vi "Text control 2 v5.8_pump-specific.vi"() -> ()   [LabVIEW 2016]
panel:
  in  "Tab Control":enum32{"Main", "Other parameters"}(tab)
  out "Line running":i32
  out "Total lines":i32
  out "Path":path=path "C:/users/rlp38/09Apr2009LTtesting/test2.txt"
  out "I vs Vg":cluster{"Y data in":dbl[], "X data in":dbl[]}[](graph)
  out "Is max":dbl format="%.2e"
  out "Id max":dbl format="%.2e"
  out "Ig max":dbl format="%.2e"
  out "Imax vs time":cluster{"Y data in":dbl[], "X data in":dbl[]}[](graph)
  out "Imin vs time":cluster{"Y data in":dbl[], "X data in":dbl[]}[](graph)
  out "I vs Vd":cluster{"Y data in":dbl[], "X data in":dbl[]}[](graph)
  in  "Script":string="#-------------------------------------------------------\n# SPM pump cleaning script\n#\n# Version 0.5\n# Author: Dimitrios Simatos\n# Last updated: 2018-01-05\n#-------------------------------------------------------\n# Description\n#\n# This script is designed to run the cleaning sequence of the SPM OEM pump.\n# This script needs to be run 4 times!\n#-------------------------------------------------------\n# Changes\n#\n# Placed initialization and hard stop commands in the beginning.\n#-------------------------------------------------------\n# Important points\n#\n# Never leave any liquid in the pump to dry after the experiments. If they dry, the residue may block the valve.\n# Always run the cleaning cycle after the experiments.\n# Use clockwise rotation when going up in valve port numbers and vice versa.\n#-------------------------------------------------------\n# Things to do before running the script\n#\n# Set time units to minutes.\n# Set filenames.\n# Replace the tubing, if necessary.\n#-------------------------------------------------------\n# Port connections\n#\n# Port 1: Waste\n# Port 2: Waste\n# Port 3: Various cleaning liquids\n# Port 4: Waste\n# Port 5: Waste\n# Port 6: Waste\n#\n# Between each of the 4 runs, the settings of Port 3 will change, according to the cleaning protocol.\n# The settings for Port 3 are:\n# 1st run: 1% v/v solution of sodium hypochlorite in ultrapure water\n# 2nd run: 0.1% w/v solution of sodium dodecyl sulfate in ultrapure water\n# 3rd run: Ultrapure water\n# 4th run: Waste (in air, not immersed in liquid)\n#-------------------------------------------------------\n# Cleaning protocol for the SPM OEM pump (from the manual)\n#\n# A cleaning procedure should be performed at the end of each day or in between two different experiments.\n# An effective cleaning can be performed in the following manner:\n# • Bleach solution to kill microorganisms\n# 1. Prepare a solution of 1% chlorine bleach and deionized water\n#    NOTE: Prepare a 1% v/v solution of sodium hypochlorite in deionized water\n# 2. Prepare a reservoir and place 1 tubing in the bleach solution and 5 tubings in a waste recipient\n# 3. Pick up the bleach solution through 1 port to entirely fill the syringe\n# 4. Sequentially output the syringe content through the remaining ports and throw it to the waste\n# 5. Repeat operation at least 2 times\n# • Detergent solution to remove debris\n# 1. Prepare a solution of 0.1% detergent and deionized water\n#    NOTE: Prepare a 0.1% w/v solution of sodium dodecyl sulfate in deionized water\n# 2. Move the tubing from the bleach solution reservoir and place it into a reservoir of detergent solution\n# 3. Pick up the detergent solution through 1 port to entirely fill the syringe\n# 4. Sequentially output the detergent solution through the remaining ports into the waste recipient\n# 5. Repeat operation at least 2 times\n# • Rinsing water to prepare the pump for your next experiment\n# 1. Move the tubing from the detergent solution reservoir and place it into a reservoir of deionized water\n# 2. Pick up the rinsing solution through 1 port to entirely fill the syringe\n# 3. Sequentially output the rinse water through the remaining ports into the waste recipient\n# 4. Repeat operation at least 2 times\n# • Replace the tubing, if necessary\n#-------------------------------------------------------\n# Pumping cycles and execution time\n#\n# Execution time for a single cycle: 6 x (1 min + 10 sec) = 7 minutes\n# Total execution time: 4 x 7 = 28 minutes\n# Since the script has to run 4 times, the cleaning lasts for: 4 x 28 = 112 minutes\n# Air must be the last to be pumped through the valve, to remove all liquids.\n# There are 4 pumping cycles. Each one draws a different liquid through port 3 and pumps it sequentially through ports 1,2,4,5,6.\n# During the sequential pumping, each port receives 200 ml of liquid (20% of the total syringe volume = 600 \"plunger units\")\n# The device must be disconnected from the port during the cleaning procedure.\n# All cycles are similar, except cycle 1 has the initialization command uncommented and the first report valve command commented.\n#-------------------------------------------------------\n# Volume of liquid needed\n#\n# Volume of liquid needed per cycle: 1 ml\n# Total volume of liquid needed per script run: 4 x 1 = 4 ml\n# Since the script has to run 4 times, the first 3 with different liquids, I need:\n# 4 ml of 1% v/v solution of sodium hypochlorite in ultrapure water\n# 4 ml of 0.1% w/v solution of sodium dodecyl sulfate in ultrapure water\n# 4 ml of ultrapure water\n#-------------------------------------------------------\n# Parameters\n#\n# Syringe size: 1 ml\n# Step resolution N = 0.01 mm\n# Drawing flow V = 300 pulses/second (6000 ul/min)\n# Pumping flow V = 300 pulses/second (6000 ul/min)\n#-------------------------------------------------------\n# Pump initialization\npump /1T #hard stop pump\npump /1ZR #initialize pump\n#-------------------------------------------------------\n# Cycle 1\n# Fill the syringe\npump /1Q #query pump\npump /1? #report absolute plunger position\n#pump /1?6 #report valve position\nwait-min 1 #wait 1 minute\npump /1N0R #set step resolution: 0.01 mm\npump /1Q #query pump\npump /1? #report absolute plunger position (the plunger should be at 0)\npump /1?6 #report valve position\nwait 1000 #wait 1 second\npump /1V300R #choose speed: 300 steps/s (6000 ul/min)\npump /1Q #query pump\nwait 1000 #wait 1 second\npump /1I3R #go to port 3, clockwise rotation\npump /1Q #query pump\npump /1?6 #report valve position\nwait 1000 #wait 1 second\npump /1A3000R #go to absolute position 3000 (= draw 1 ml)\nwait 30000 #wait 30 seconds\npump /1Q #query pump\npump /1? #report absolute plunger position (the plunger should have finished moving)\n#pump /1?6 #report valve position\n# The sequential pumping begins\n# Port 1\npump /1O1R #switch to port 1, counterclockwise rotation\npump /1Q #query pump\npump /1?6 #report valve position\npump /1A2400R #go to absolute position 2400 (= pump 200 ul)\npump /1Q #query pump\npump /1? #report absolute plunger position (the plunger should be moving to 0)\nwait-min 1 #wait 1 minute\npump /1? #report absolute plunger position (the plunger should have finished moving)\n# Port 2\npump /1I2R #switch to port 2, clockwise rotation\npump /1Q #query pump\npump /1?6 #report valve position\npump /1A1800R #go to absolute position 1800 (= pump 200 ul)\npump /1Q #query pump\npump /1? #report absolute plunger position (the plunger should be moving to 0)\nwait-min 1 #wait 1 minute\npump /1? #report absolute plunger position (the plunger should have finished moving)\n# Port 4\npump /1I4R #switch to port 4, clockwise rotation\npump /1Q #query pump\npump /1?6 #report valve position\npump /1A1200R #go to absolute position 1200 (= pump 200 ul)\npump /1Q #query pump\npump /1? #report absolute plunger position (the plunger should be moving to 0)\nwait-min 1 #wait 1 minute\npump /1? #report absolute plunger position (the plunger should have finished moving)\n# Port 5\npump /1I5R #switch to port 5, clockwise rotation\npump /1Q #query pump\npump /1?6 #report valve position\npump /1A600R #go to absolute position 600 (= pump 200 ul)\npump /1Q #query pump\npump /1? #report absolute plunger position (the plunger should be moving to 0)\nwait-min 1 #wait 1 minute\npump /1? #report absolute plunger position (the plunger should have finished moving)\n# Port 6\npump /1I6R #switch to port 6, clockwise rotation\npump /1Q #query pump\npump /1?6 #report valve position\npump /1A0R #go to absolute position 0 (= pump 200 ul)\npump /1Q #query pump\npump /1? #report absolute plunger position (the plunger should be moving to 0)\nwait-min 1 #wait 1 minute\npump /1? #report absolute plunger position (the plunger should have finished moving)\n#-------------------------------------------------------\n# Cycle 2\n# Fill the syringe\n#pump /1ZR #initialize pump\npump /1Q #query pump\npump /1? #report absolute plunger position\npump /1?6 #report valve position\nwait-min 1 #wait 1 minute\npump /1N0R #set step resolution: 0.01 mm\npump /1Q #query pump\npump /1? #report absolute plunger position (the plunger should be at 0)\npump /1?6 #report valve position\nwait 1000 #wait 1 second\npump /1V300R #choose speed: 300 steps/s (6000 ul/min)\npump /1Q #query pump\nwait 1000 #wait 1 second\npump /1O3R #go to port 3, counterclockwise rotation\npump /1Q #query pump\npump /1?6 #report valve position\nwait 1000 #wait 1 second\npump /1A3000R #go to absolute position 3000 (= draw 1 ml)\nwait 30000 #wait 30 seconds\npump /1Q #query pump\npump /1? #report absolute plunger position (the plunger should have finished moving)\n#pump /1?6 #report valve position\n# The sequential pumping begins\n# Port 1\npump /1O1R #switch to port 1, counterclockwise rotation\npump /1Q #query pump\npump /1?6 #report valve position\npump /1A2400R #go to absolute position 2400 (= pump 200 ul)\npump /1Q #query pump\npump /1? #report absolute plunger position (the plunger should be moving to 0)\nwait-min 1 #wait 1 minute\npump /1? #report absolute plunger position (the plunger should have finished moving)\n# Port 2\npump /1I2R #switch to port 2, clockwise rotation\npump /1Q #query pump\npump /1?6 #report valve position\npump /1A1800R #go to absolute position 1800 (= pump 200 ul)\npump /1Q #query pump\npump /1? #report absolute plunger position (the plunger should be moving to 0)\nwait-min 1 #wait 1 minute\npump /1? #report absolute plunger position (the plunger should have finished moving)\n# Port 4\npump /1I4R #switch to port 4, clockwise rotation\npump /1Q #query pump\npump /1?6 #report valve position\npump /1A1200R #go to absolute position 1200 (= pump 200 ul)\npump /1Q #query pump\npump /1? #report absolute plunger position (the plunger should be moving to 0)\nwait-min 1 #wait 1 minute\npump /1? #report absolute plunger position (the plunger should have finished moving)\n# Port 5\npump /1I5R #switch to port 5, clockwise rotation\npump /1Q #query pump\npump /1?6 #report valve position\npump /1A600R #go to absolute position 600 (= pump 200 ul)\npump /1Q #query pump\npump /1? #report absolute plunger position (the plunger should be moving to 0)\nwait-min 1 #wait 1 minute\npump /1? #report absolute plunger position (the plunger should have finished moving)\n# Port 6\npump /1I6R #switch to port 6, clockwise rotation\npump /1Q #query pump\npump /1?6 #report valve position\npump /1A0R #go to absolute position 0 (= pump 200 ul)\npump /1Q #query pump\npump /1? #report absolute plunger position (the plunger should be moving to 0)\nwait-min 1 #wait 1 minute\npump /1? #report absolute plunger position (the plunger should have finished moving)\n#-------------------------------------------------------\n# Cycle 3\n# Fill the syringe\n#pump /1ZR #initialize pump\npump /1Q #query pump\npump /1? #report absolute plunger position\npump /1?6 #report valve position\nwait-min 1 #wait 1 minute\npump /1N0R #set step resolution: 0.01 mm\npump /1Q #query pump\npump /1? #report absolute plunger position (the plunger should be at 0)\npump /1?6 #report valve position\nwait 1000 #wait 1 second\npump /1V300R #choose speed: 300 steps/s (6000 ul/min)\npump /1Q #query pump\nwait 1000 #wait 1 second\npump /1O3R #go to port 3, counterclockwise rotation\npump /1Q #query pump\npump /1?6 #report valve position\nwait 1000 #wait 1 second\npump /1A3000R #go to absolute position 3000 (= draw 1 ml)\nwait 30000 #wait 30 seconds\npump /1Q #query pump\npump /1? #report absolute plunger position (the plunger should have finished moving)\n#pump /1?6 #report valve position\n# The sequential pumping begins\n# Port 1\npump /1O1R #switch to port 1, counterclockwise rotation\npump /1Q #query pump\npump /1?6 #report valve position\npump /1A2400R #go to absolute position 2400 (= pump 200 ul)\npump /1Q #query pump\npump /1? #report absolute plunger position (the plunger should be moving to 0)\nwait-min 1 #wait 1 minute\npump /1? #report absolute plunger position (the plunger should have finished moving)\n# Port 2\npump /1I2R #switch to port 2, clockwise rotation\npump /1Q #query pump\npump /1?6 #report valve position\npump /1A1800R #go to absolute position 1800 (= pump 200 ul)\npump /1Q #query pump\npump /1? #report absolute plunger position (the plunger should be moving to 0)\nwait-min 1 #wait 1 minute\npump /1? #report absolute plunger position (the plunger should have finished moving)\n# Port 4\npump /1I4R #switch to port 4, clockwise rotation\npump /1Q #query pump\npump /1?6 #report valve position\npump /1A1200R #go to absolute position 1200 (= pump 200 ul)\npump /1Q #query pump\npump /1? #report absolute plunger position (the plunger should be moving to 0)\nwait-min 1 #wait 1 minute\npump /1? #report absolute plunger position (the plunger should have finished moving)\n# Port 5\npump /1I5R #switch to port 5, clockwise rotation\npump /1Q #query pump\npump /1?6 #report valve position\npump /1A600R #go to absolute position 600 (= pump 200 ul)\npump /1Q #query pump\npump /1? #report absolute plunger position (the plunger should be moving to 0)\nwait-min 1 #wait 1 minute\npump /1? #report absolute plunger position (the plunger should have finished moving)\n# Port 6\npump /1I6R #switch to port 6, clockwise rotation\npump /1Q #query pump\npump /1?6 #report valve position\npump /1A0R #go to absolute position 0 (= pump 200 ul)\npump /1Q #query pump\npump /1? #report absolute plunger position (the plunger should be moving to 0)\nwait-min 1 #wait 1 minute\npump /1? #report absolute plunger position (the plunger should have finished moving)\n#-------------------------------------------------------\n# Cycle 4\n# Fill the syringe\n#pump /1ZR #initialize pump\npump /1Q #query pump\npump /1? #report absolute plunger position\npump /1?6 #report valve position\nwait-min 1 #wait 1 minute\npump /1N0R #set step resolution: 0.01 mm\npump /1Q #query pump\npump /1? #report absolute plunger position (the plunger should be at 0)\npump /1?6 #report valve position\nwait 1000 #wait 1 second\npump /1V300R #choose speed: 300 steps/s (6000 ul/min)\npump /1Q #query pump\nwait 1000 #wait 1 second\npump /1O3R #go to port 3, counterclockwise rotation\npump /1Q #query pump\npump /1?6 #report valve position\nwait 1000 #wait 1 second\npump /1A3000R #go to absolute position 3000 (= draw 1 ml)\nwait 30000 #wait 30 seconds\npump /1Q #query pump\npump /1? #report absolute plunger position (the plunger should have finished moving)\n#pump /1?6 #report valve position\n# The sequential pumping begins\n# Port 1\npump /1O1R #switch to port 1, counterclockwise rotation\npump /1Q #query pump\npump /1?6 #report valve position\npump /1A2400R #go to absolute position 2400 (= pump 200 ul)\npump /1Q #query pump\npump /1? #report absolute plunger position (the plunger should be moving to 0)\nwait-min 1 #wait 1 minute\npump /1? #report absolute plunger position (the plunger should have finished moving)\n# Port 2\npump /1I2R #switch to port 2, clockwise rotation\npump /1Q #query pump\npump /1?6 #report valve position\npump /1A1800R #go to absolute position 1800 (= pump 200 ul)\npump /1Q #query pump\npump /1? #report absolute plunger position (the plunger should be moving to 0)\nwait-min 1 #wait 1 minute\npump /1? #report absolute plunger position (the plunger should have finished moving)\n# Port 4\npump /1I4R #switch to port 4, clockwise rotation\npump /1Q #query pump\npump /1?6 #report valve position\npump /1A1200R #go to absolute position 1200 (= pump 200 ul)\npump /1Q #query pump\npump /1? #report absolute plunger position (the plunger should be moving to 0)\nwait-min 1 #wait 1 minute\npump /1? #report absolute plunger position (the plunger should have finished moving)\n# Port 5\npump /1I5R #switch to port 5, clockwise rotation\npump /1Q #query pump\npump /1?6 #report valve position\npump /1A600R #go to absolute position 600 (= pump 200 ul)\npump /1Q #query pump\npump /1? #report absolute plunger position (the plunger should be moving to 0)\nwait-min 1 #wait 1 minute\npump /1? #report absolute plunger position (the plunger should have finished moving)\n# Port 6\npump /1I6R #switch to port 6, clockwise rotation\npump /1Q #query pump\npump /1?6 #report valve position\npump /1A0R #go to absolute position 0 (= pump 200 ul)\npump /1Q #query pump\npump /1? #report absolute plunger position (the plunger should be moving to 0)\nwait-min 1 #wait 1 minute\npump /1? #report absolute plunger position (the plunger should have finished moving)\n#-------------------------------------------------------"
  out "Command running:":string
  out "Serial port data":string
  out "Elapsed Time":dbl caption="Elapsed Time (s)"
  in  "Units":u16(ring)=1 items=["Seconds", "Minutes", "Hours"]
  in  "Time Offset":dbl caption="Set Start Time (s)"
  in  "Reset":bool
  in  "Auto Reset":bool
  in  "integration time":u32(slide) max=2 step=1 scale=0.0..2.0
  in  "Interrupt run":bool
  out "Absolute plunger position vs time":cluster{"Y data in":dbl[], "X data in":dbl[]}[](graph)
  out "Valve position vs time":cluster{"Y data in":dbl[], "X data in":dbl[]}[](graph)
  out "Is on":dbl format="%.2e"
  out "Id on":dbl format="%.2e"
  out "Ig on":dbl format="%.2e"
  out "Ion vs time":cluster{"Y data in":dbl[], "X data in":dbl[]}[](graph)
  out "Ioff vs time":cluster{"Y data in":dbl[], "X data in":dbl[]}[](graph)
  out "Ig min":dbl format="%.2e"
  out "Id min":dbl format="%.2e"
  out "Is min":dbl format="%.2e"
  out "Is off":dbl format="%.2e"
  out "Id off":dbl format="%.2e"
  out "Ig off":dbl format="%.2e"
  in  "Integration time (long)":dbl=0.32 min=0.04 max=2.0 step=0.02 format="%.2f"
  in  "Integration time (short)":dbl=0.0019 min=8e-05 max=0.0019 step=8e-05 format="%^.0e"
  in  "Gate: Compliance":dbl=0.001 format="%.8f"
  in  "Drain: Compliance":dbl=0.001 format="%.8f"
  in  "Hard stop pump":bool
  in  "Halt pump":bool
  in  "Gate Range\nmode":u16(ring) items=["Auto", "Limited", "Fixed"]
  in  "Gate Range":u8(slide)=6 max=11 scale=0.0..11.0
  in  "Source/Drain\nRange mode":u16(ring) items=["Auto", "Limited", "Fixed"]
  in  "Source/Drain Range":u8(slide)=6 max=11 scale=0.0..11.0
  in  "Panel Controls":T1={"Emergency Stop"=refnum, "TransGraph Max"=1e-05, "Text/Graph (text=false)"=TRUE} {"TransGraph Max" format="%.2e"}
  in  "Panel Controls 2":T2={"Emergency Stop"=refnum, "TransGraph Max"=1e-05, "Text/Graph (text=false)"=TRUE, "TransGraph Min"=1e-11} {"TransGraph Min" format="%.2e"; "TransGraph Max" format="%.2e"}
  in  "SMU4":cluster{"on/off":bool, "Voltage":dbl} {"Voltage" min=-100.0 max=100.0 format="%.2f"}
  in  "Full Reset":bool
  in  "Standby":T3
  out "error out":errorcluster
  in  "Delay before read (ms)":u32=1000
  in  "byte count":u32=64
  in  "Serial End Mode for Reads":u16(ring)=2 items=["None", "LastBit", "TermChar"]
  in  "Timeout (ms)":u32=10000
  in  "Enable Termination\nChar (T)":bool=TRUE
  in  "Termination char\n(0xA = '\\n' = LF)\n(0xD = '\\r' = CR)":u8=13 format="%.0x"
  in  "flow control":u16(ring) items=["None"=0, "XON/XOFF"=1, "RTS/CTS"=2, "DTR/DSR"=4]
  in  "stop bits":u16(ring)=10 items=["1.0"=10, "1.5"=15, "2.0"=20]
  in  "parity":u16(ring) items=["None", "Odd", "Even", "Mark", "Space"]
  in  "data bits":u16=8 min=5 max=8 step=1
  in  "VISA resource name":refnum<visa-resource-name>="COM6"
  in  "baud rate":u32=9600
  in  "Filename (variable part)":string="step_1_up-H2O_initial_"
  in  "Suffix (script)":string="step_1_up-H2O_initial_script.txt"
  out "Timings Indicator":T4
  in  "Timings (overwritten by the Front Panel)":T5={"integration time"=0, "Short/Long integration time"=0.00064, "hold time (sec)"=0.0, "delay time (sec)"=0.0, "Step Time (0 disables)"=0.0, "sweep method"=0, "Pulse period"=0.005, "Base voltage"=0.0, "Pulse width"=0.0005} {"Pulse width" min=0.0005 max=0.1 step=0.0001 format="%.4f"; "Base voltage" format="%^.4e"; "Pulse period" min=0.005 max=1.0 step=0.0001 format="%.4f"; "sweep method" items=["Continuous", "Pulsed"]; "Step Time (0 disables)" format="%.2f"; "delay time (sec)" format="%.4f"; "hold time (sec)" format="%.4f"; "Short/Long integration time" format="%^.0e"; "integration time" scale=0.0..2.0}
  in  "Gate":T6={"Gate Start"=0.0, "Gate Stop"=2.0, "Gate Step (linear only)"=1.0, "Gate Compliance"=0.0001, "Gate PComp"=0.0, "Range mode"=0, "Range"=6} {"Range" max=11 scale=0.0..11.0; "Range mode" items=["Auto", "Limited", "Fixed"]; "Gate PComp" format="%^.2e"; "Gate Compliance" format="%^.2e"; "Gate Step (linear only)" format="%^.4e"; "Gate Stop" format="%^.4e"; "Gate Start" format="%^.4e"}
  in  "Drain 2":T7={"Drain Start"=0.0, "Drain Stop"=2.0, "Drain Compliance"=0.0001, "Drain Step"=1.0, "Drain PComp"=0.0, "Range mode"=0, "Range"=6} {"Range" max=11 scale=0.0..11.0; "Range mode" items=["Auto", "Limited", "Fixed"]; "Drain PComp" format="%^.2e"; "Drain Step" format="%^.4e"; "Drain Compliance" format="%^.2e"; "Drain Stop" format="%^.4e"; "Drain Start" format="%^.4e"}
  # "Syntax:\nitime [s|m|l] time(sec): [s|m|l] determines the integration time setting (small|medium|long) and time sets the value.\nNOTE: The value of the integration time has to be within the range allowed by its category, otherwise, the closest value will be used. (e.g. if the itime is set to short with a very long integration time value, the actual value used will be the maximum short integration time.\nIntegration times:\n    Short: Default: 640 us. Range: 8E-5 - 1.92E-3 seconds.\n    Medium: Fixed at 1 NPL cycle (0.02 seconds).\n    Long: Default: 16 NPL cycles (0.32 seconds). Range: 2-100 NPL cycles (0.04 seconds - 2 seconds).\ngaterangemode [a|l|f]\ndrainrangemode [a|l|f]\npulsed [on|off] PulsePeriod(sec) PulseBaseVoltage PulseONWidth(sec)\nstandby [on l off]\nwait NumMilliseconds\nwait-min NumMinutes\n# texthere = comment\ntransfer [s|d] VgStart VgStop VgStep VdStart VdStop VdStep\noutput [s|d] VgStart VgStop VgStep VdStart VdStop VdStep\nsample Vg Vd NumSamples Time(s) SampleInterval(s)\nsamplei Idg NumSamples Time(s) SampleInterval(s) VDGcompliance\n100 samples is approximately 13 seconds with medium integration\n# if in doubt use SampleInterval(s) = 0.004\nstressV VG VD IGcompliance IDcompliance Duration(sec)\nstressI IDG VDGcompliance Duration(sec)\nvsu2pulse Bias Duration(s)\npulsedstressV [s|d] VEstop VgON VgOFF Period(s) PulseONwidth(s) Vd\nsample-fpp Vg Vd NumSamples Time\nresample-fpp Vg Vd\ntransfer-fpp [s|d] VgStart VgStop VgStep VdStart VdStop VdStep\noutput-fpp [s|d] VgStart VgStop VgStep VdStart VdStop VdStep\nserial SerialPortCommand\npump SerialPortCommand for the SPM pump\n\nSPM Pump Syntax (<x>: pump number, use 1 if only one pump):\nif the command syntax contains [R], then append the letter R to the command\n/<x>Q: query (a query command should follow each command)\n/<x>Z[R] or /<x>Y[R]: initialize pump\n/<x>N<n>[R] (<n>=0,1): <0> (<1>) microstep 0.01 mm (0.00125 mm) resolution\n/<x>I<n> (<n>=0-6): turn to port number n (clockwise)\n/<x>O<n> (<n>=0-6): turn to port number n (counterclockwise)\n/<x>X: Re-execute last command string\n/<x>G<n>[R] (<n>=0-60000): repeat command sequence (default: 0, 0=loop forever)\n/<x>g: Mark the start of a repeat sequence (max = 10)\n/<x>M<n>[R] (<n>=0-86400000): delay command execution by n milliseconds\n/<x>H: Halt; Pause the sequence after finishing the current move\n/<x>T: Hardstop; Interrupt the current move and suppress it from the sequence\n/<x>A<n>[R] (<n>=0-3000 with N=0, 0-24000 with N=1): absolute position\n/<x>P<n>[R] (<n>=0-3000 with N=0, 0-24000 with N=1): relative pickup\n/<x>D<n>[R] (<n>=0-3000 with N=0, 0-24000 with N=1): relative dispense\n/<x>V<n>[R] (<n>=1-1600 default: 150): set peak speed (pulses/sec)\nNOTE: The lowest speed limit is 1 pulse/sec, not 5, as the manual states.\n/<x>S<n>[R] (<n>=10-40 default: 22): set speed (NOT in pulses/sec, look in manual)\nNOTE: When controlled with absolute position, one does not need to pay special attention to the syringe that is mounted on the pump.\nWithdraw from lower stage (ports 3, 5), dispense from higher stage (ports 2, 4, 6).\nConnect Port 1 to waste."
  # "Time"
  # "1\n2\n3\n4\n5\n6\n7\n8\n9\n10\n11\n12\n13\n14\n15\n16\n17\n18\n19\n20"
  # "Serial port settings"
  # "Filename settings"
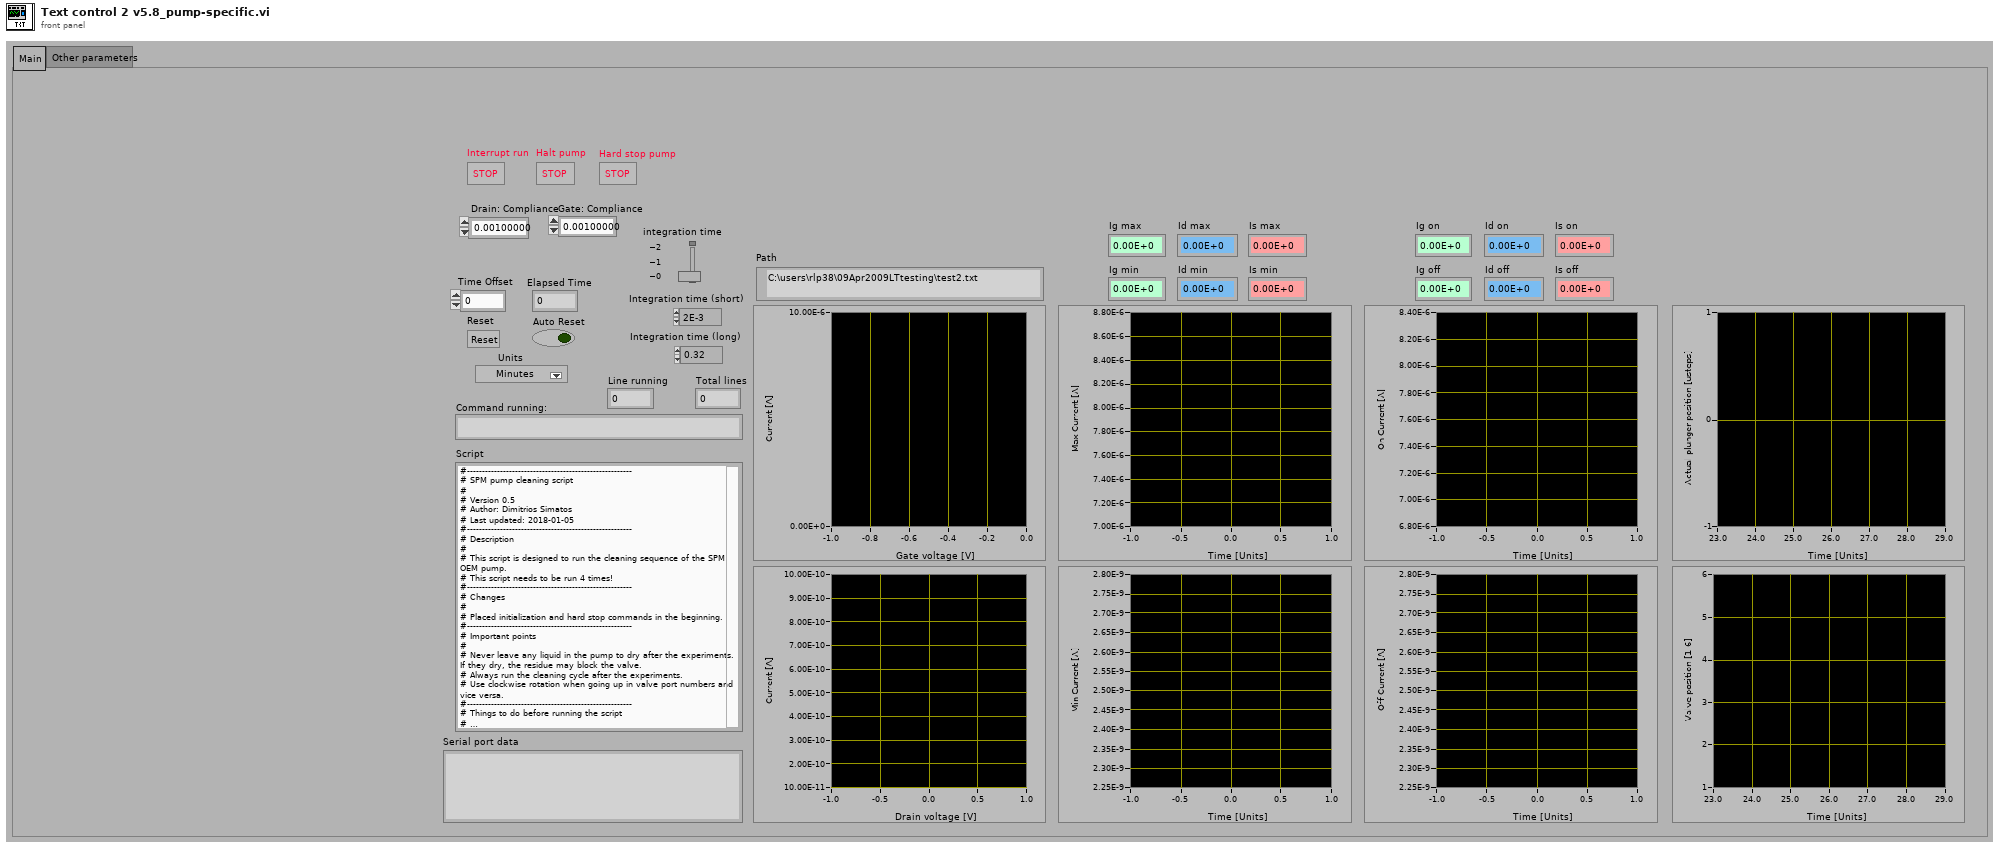
[diagram p1: front panel]
types:
  T1 = cluster{"Emergency Stop":refnum<vi>, "TransGraph Max":dbl, "Text/Graph (text=false)":bool}
  T2 = cluster{"Emergency Stop":refnum<vi>, "TransGraph Max":dbl, "Text/Graph (text=false)":bool, "TransGraph Min":dbl}
  T3 = cluster{"Gate Standby":bool, "Drain Standby":bool}
  T4 = cluster{"integration time (0:s, 1:m, 2:l)":u32, "Short/Long integration time":dbl, "hold time (sec)":dbl, "delay time (sec)":dbl, "Step Time (0 disables)":dbl, "sweep method":u16, "Pulse period":dbl, "Base voltage":dbl, "Pulse width":dbl}
  T5 = cluster{"integration time":u32, "Short/Long integration time":dbl, "hold time (sec)":dbl, "delay time (sec)":dbl, "Step Time (0 disables)":dbl, "sweep method":u16, "Pulse period":dbl, "Base voltage":dbl, "Pulse width":dbl}
  T6 = cluster{"Gate Start":dbl, "Gate Stop":dbl, "Gate Step (linear only)":dbl, "Gate Compliance":dbl, "Gate PComp":dbl, "Range mode":u16, "Range":u8}
  T7 = cluster{"Drain Start":dbl, "Drain Stop":dbl, "Drain Compliance":dbl, "Drain Step":dbl, "Drain PComp":dbl, "Range mode":u16, "Range":u8}
  T8 = enum16{"open", "replace", "create", "open or create", "replace or create", "replace or create with confirmation"}
  T9 = cluster{"V2 Start":dbl, "V2 Step":dbl, "Number of points":i32}
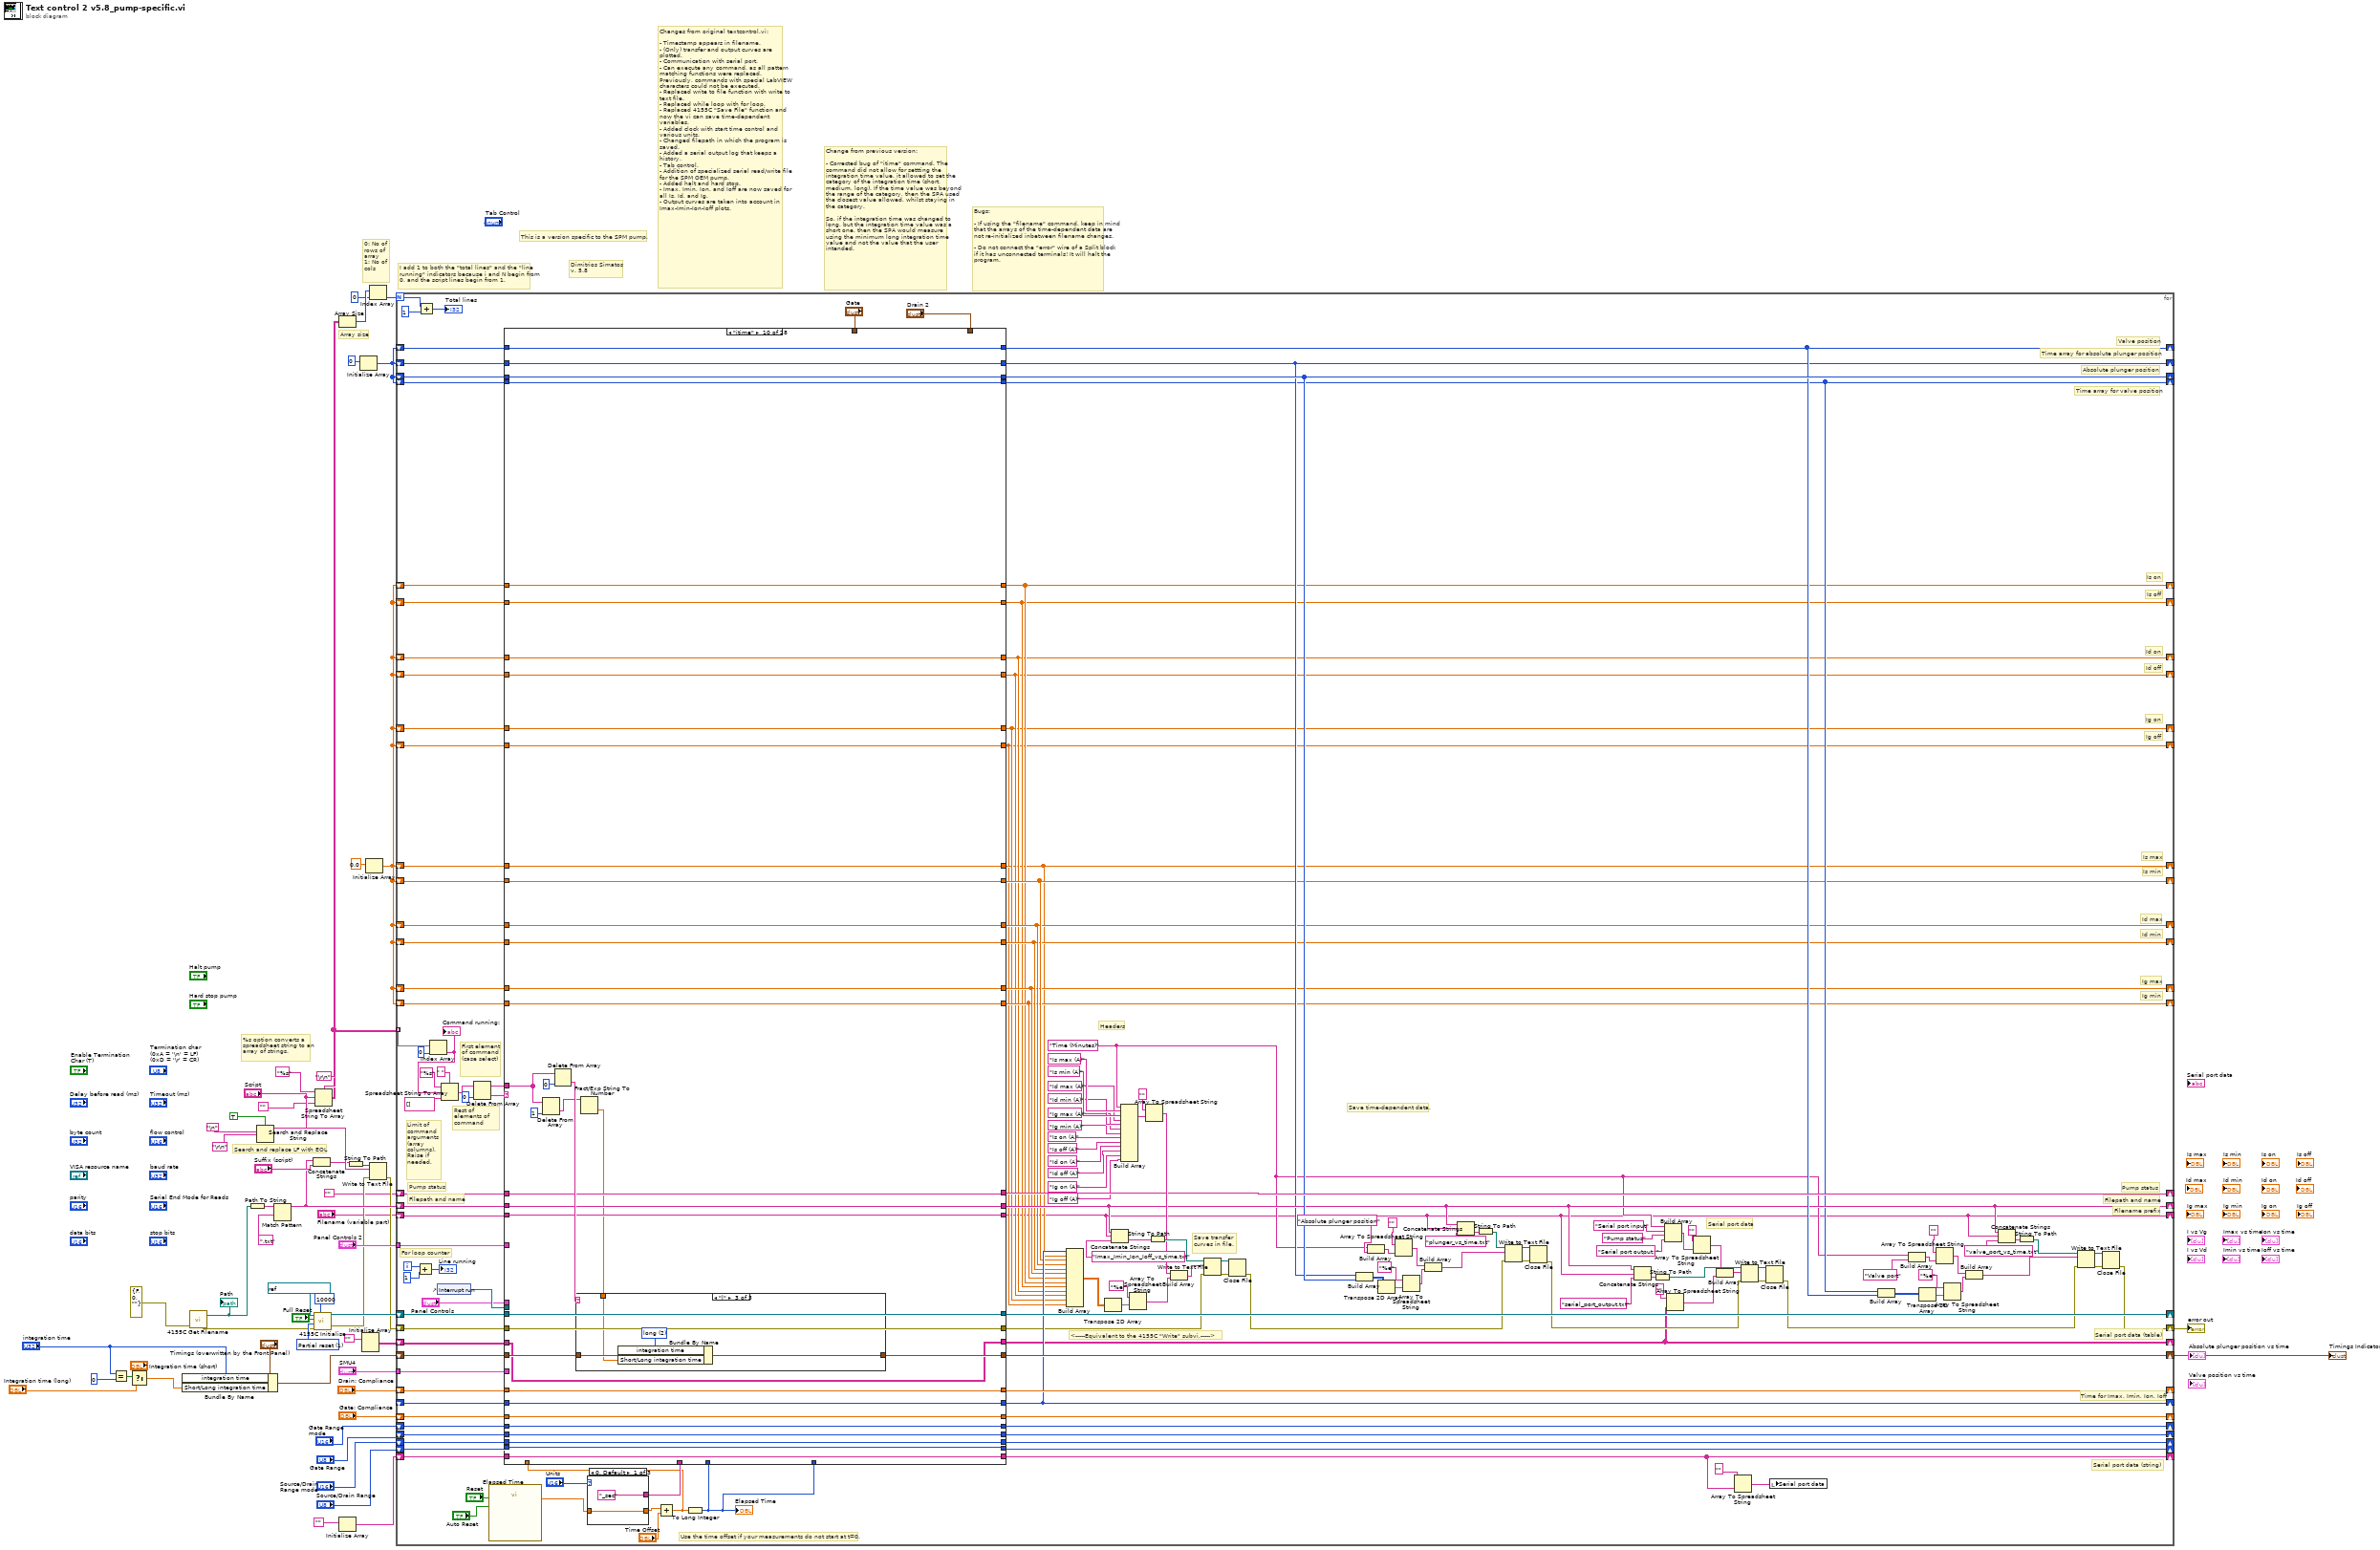
[diagram p0: block diagram]
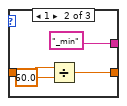
[diagram p2: hidden frame]
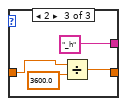
[diagram p3: hidden frame]
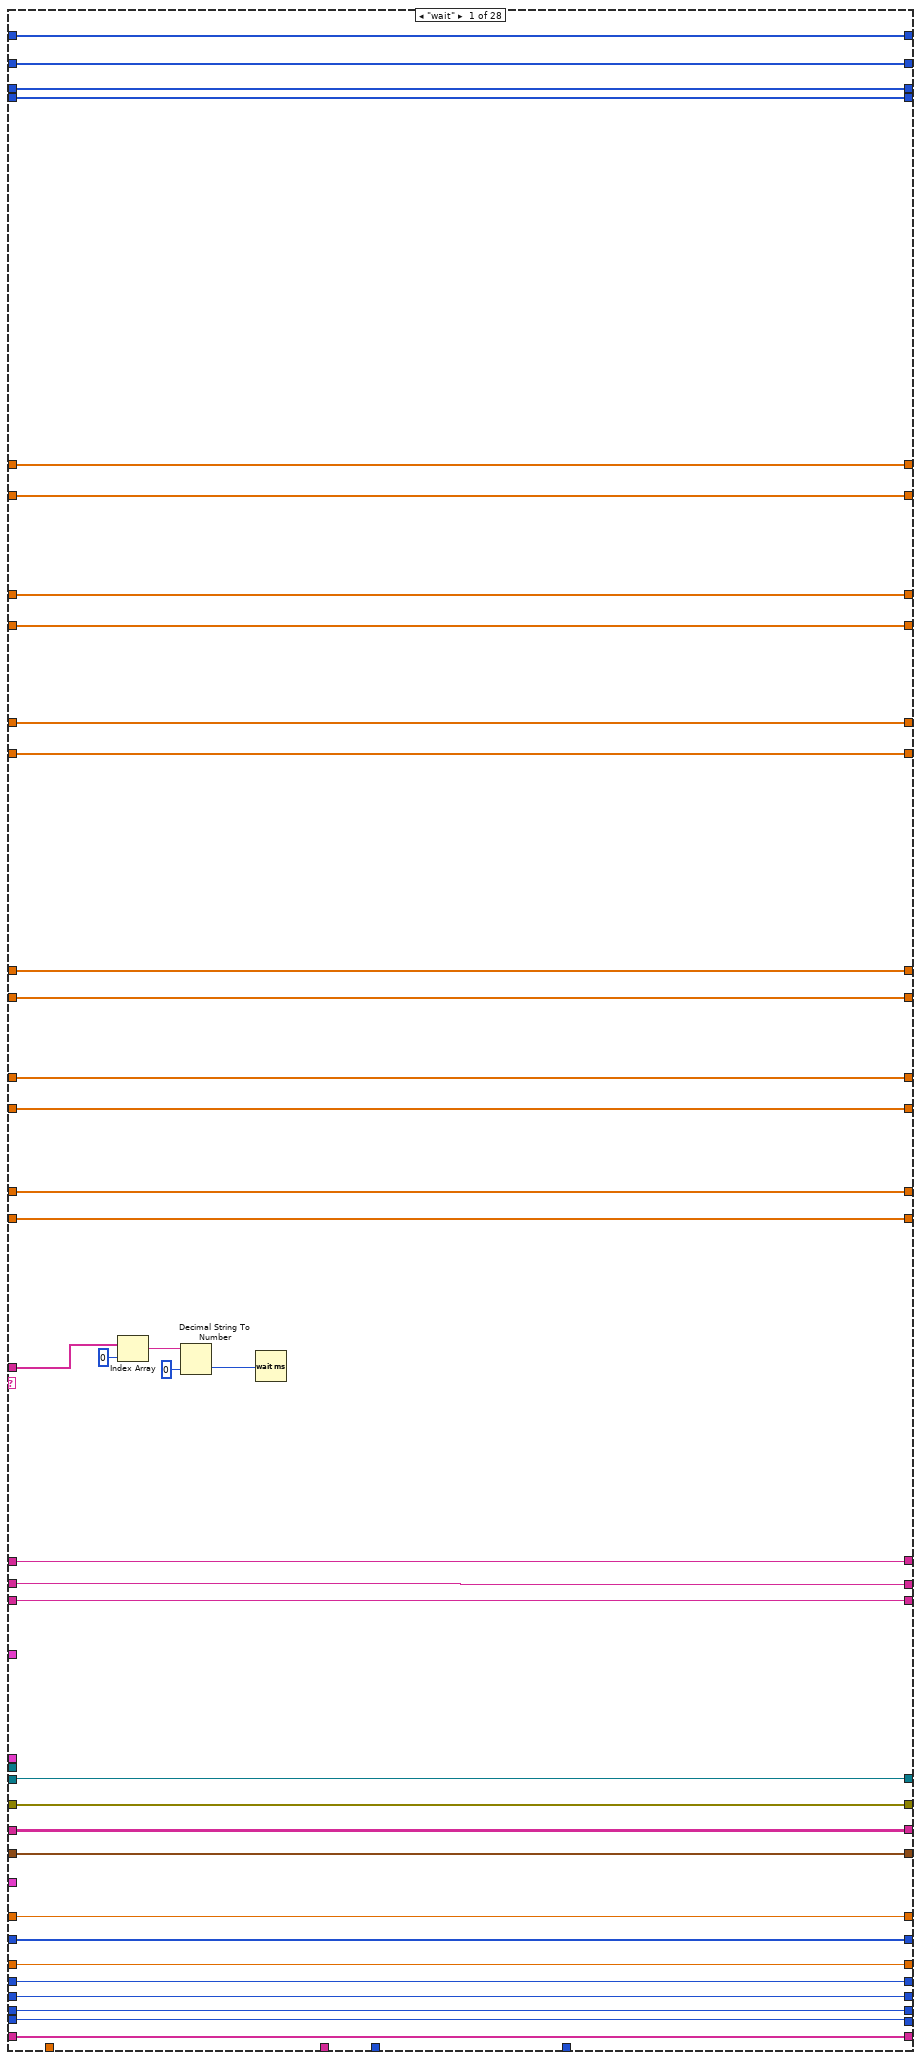
[diagram p4: hidden frame]
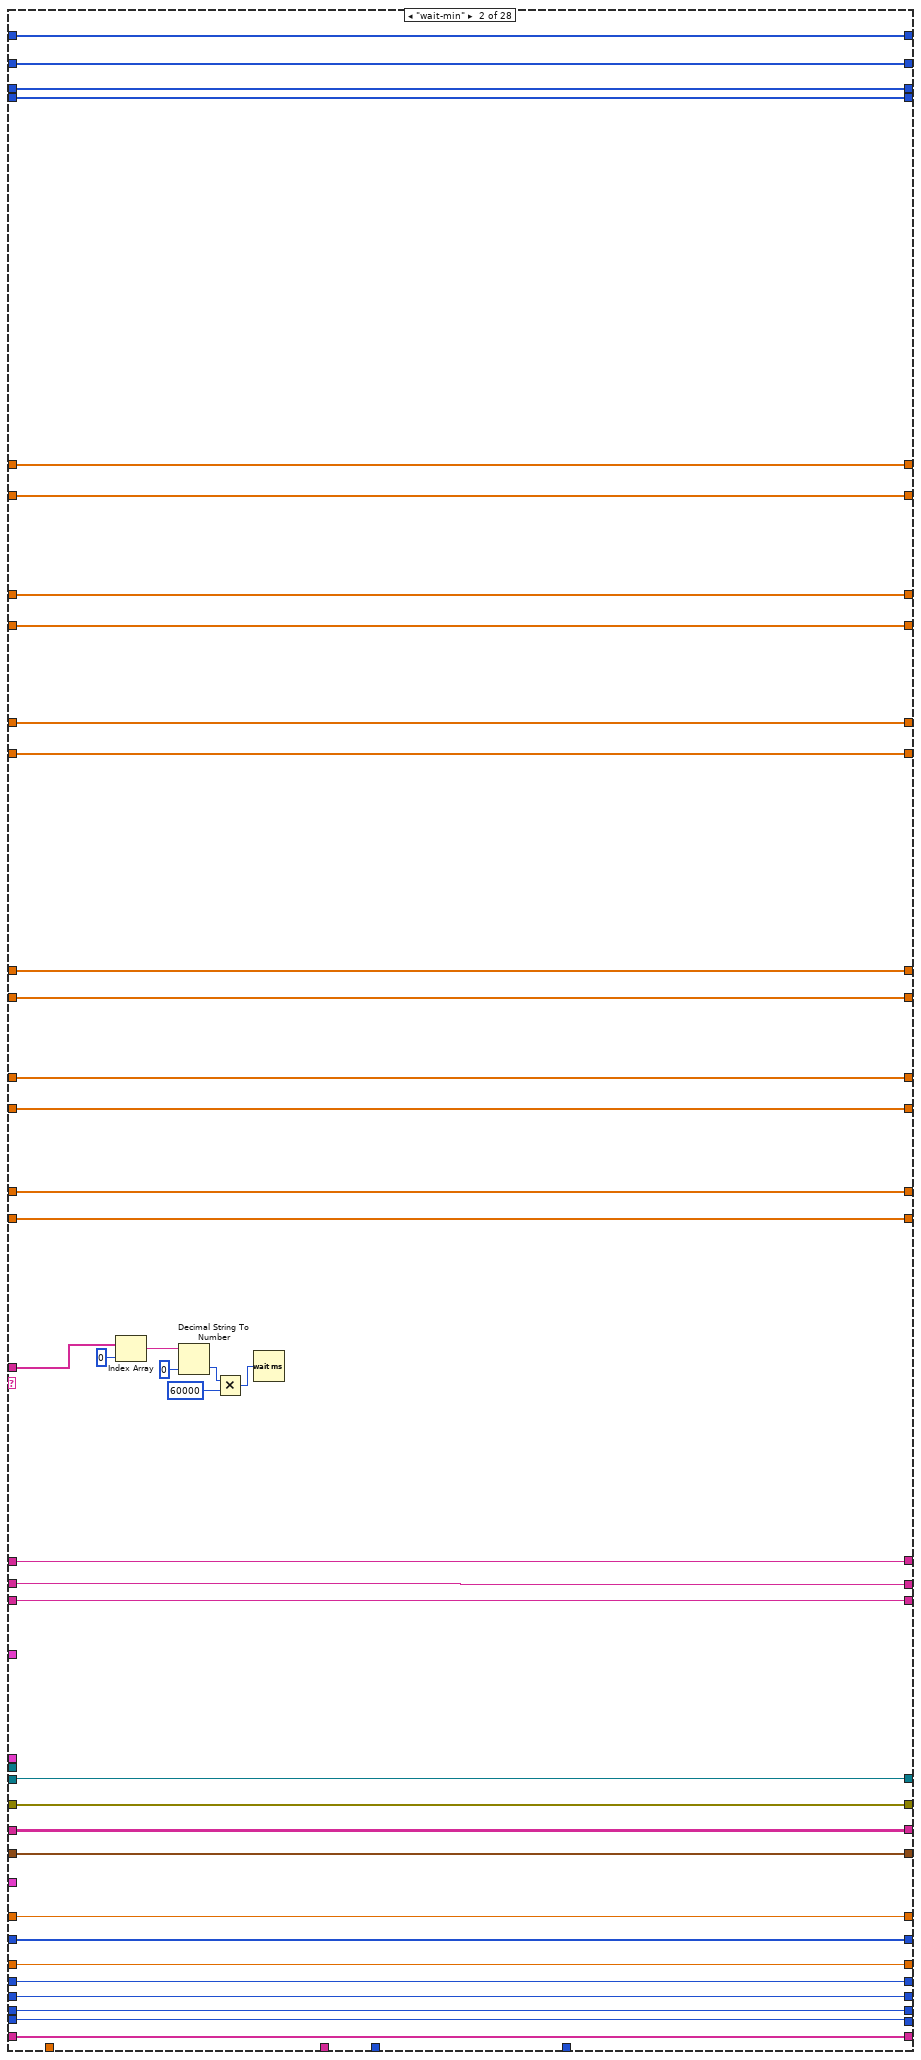
[diagram p5: hidden frame]
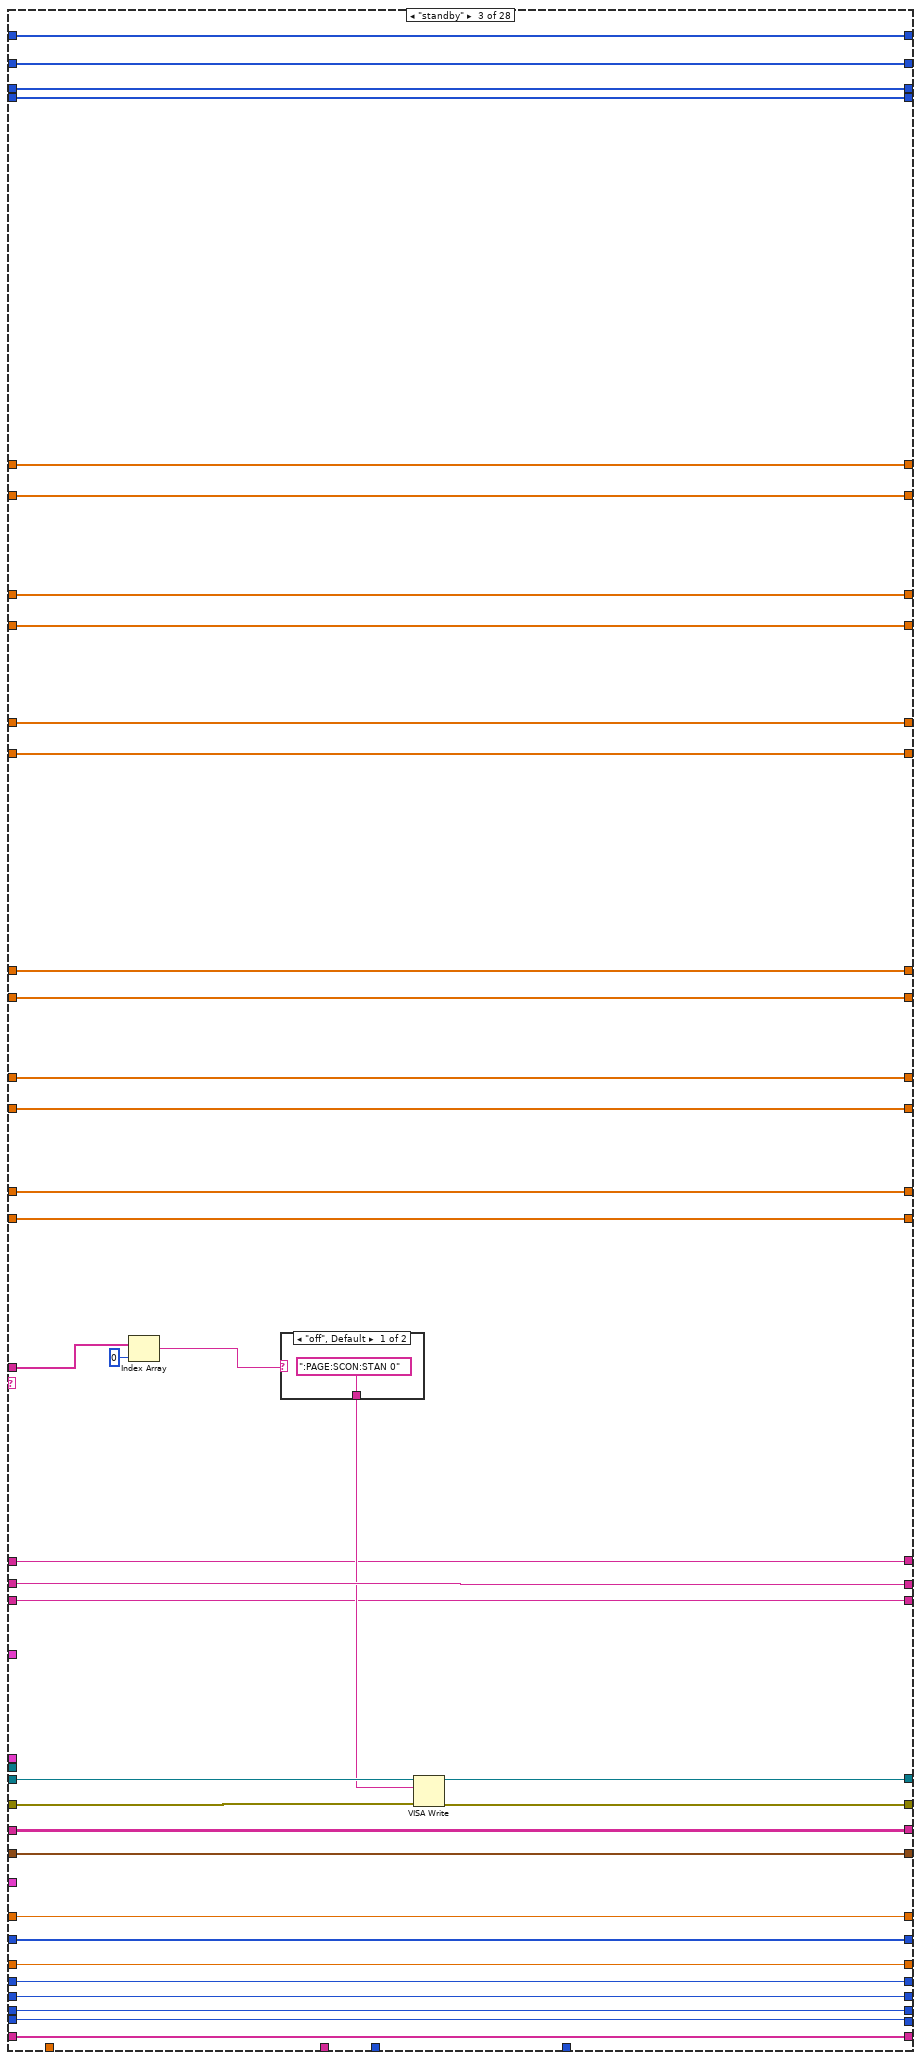
[diagram p6: hidden frame]
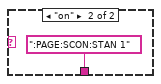
[diagram p7: hidden frame]
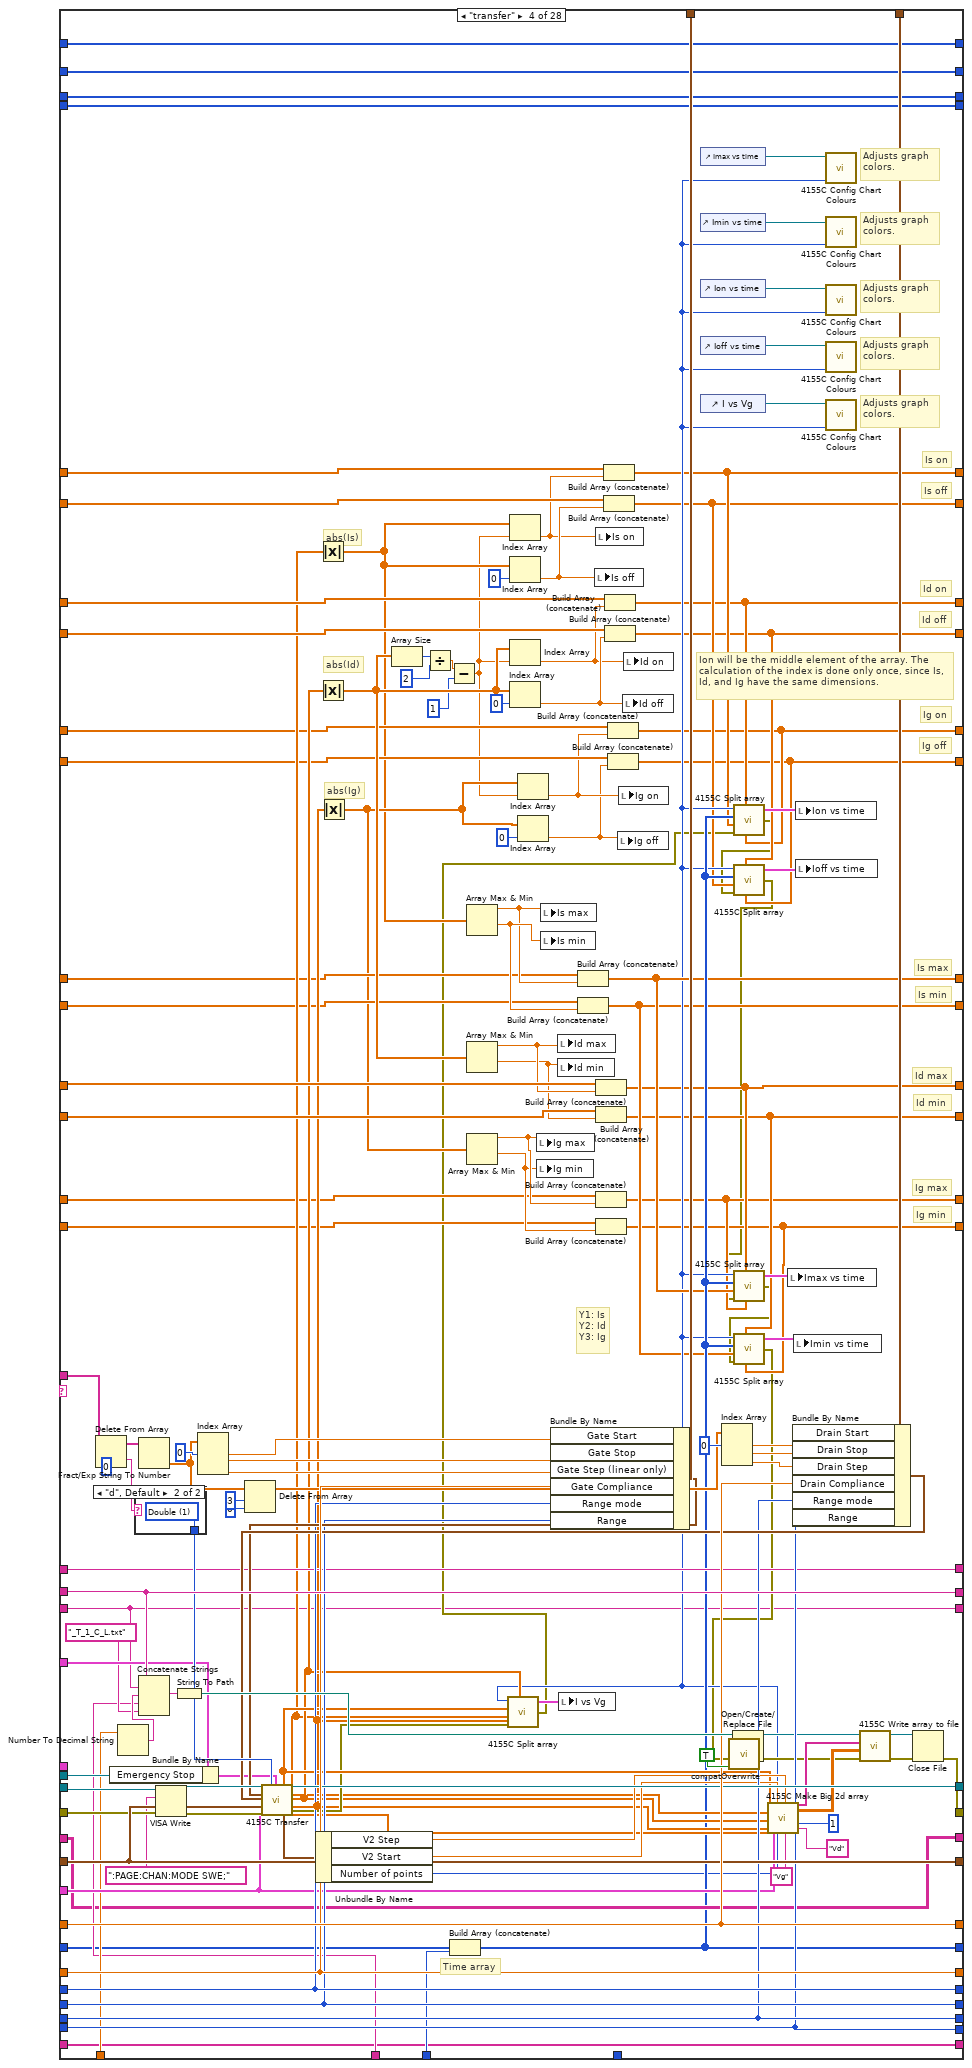
[diagram p8: hidden frame]
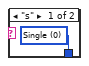
[diagram p9: hidden frame]
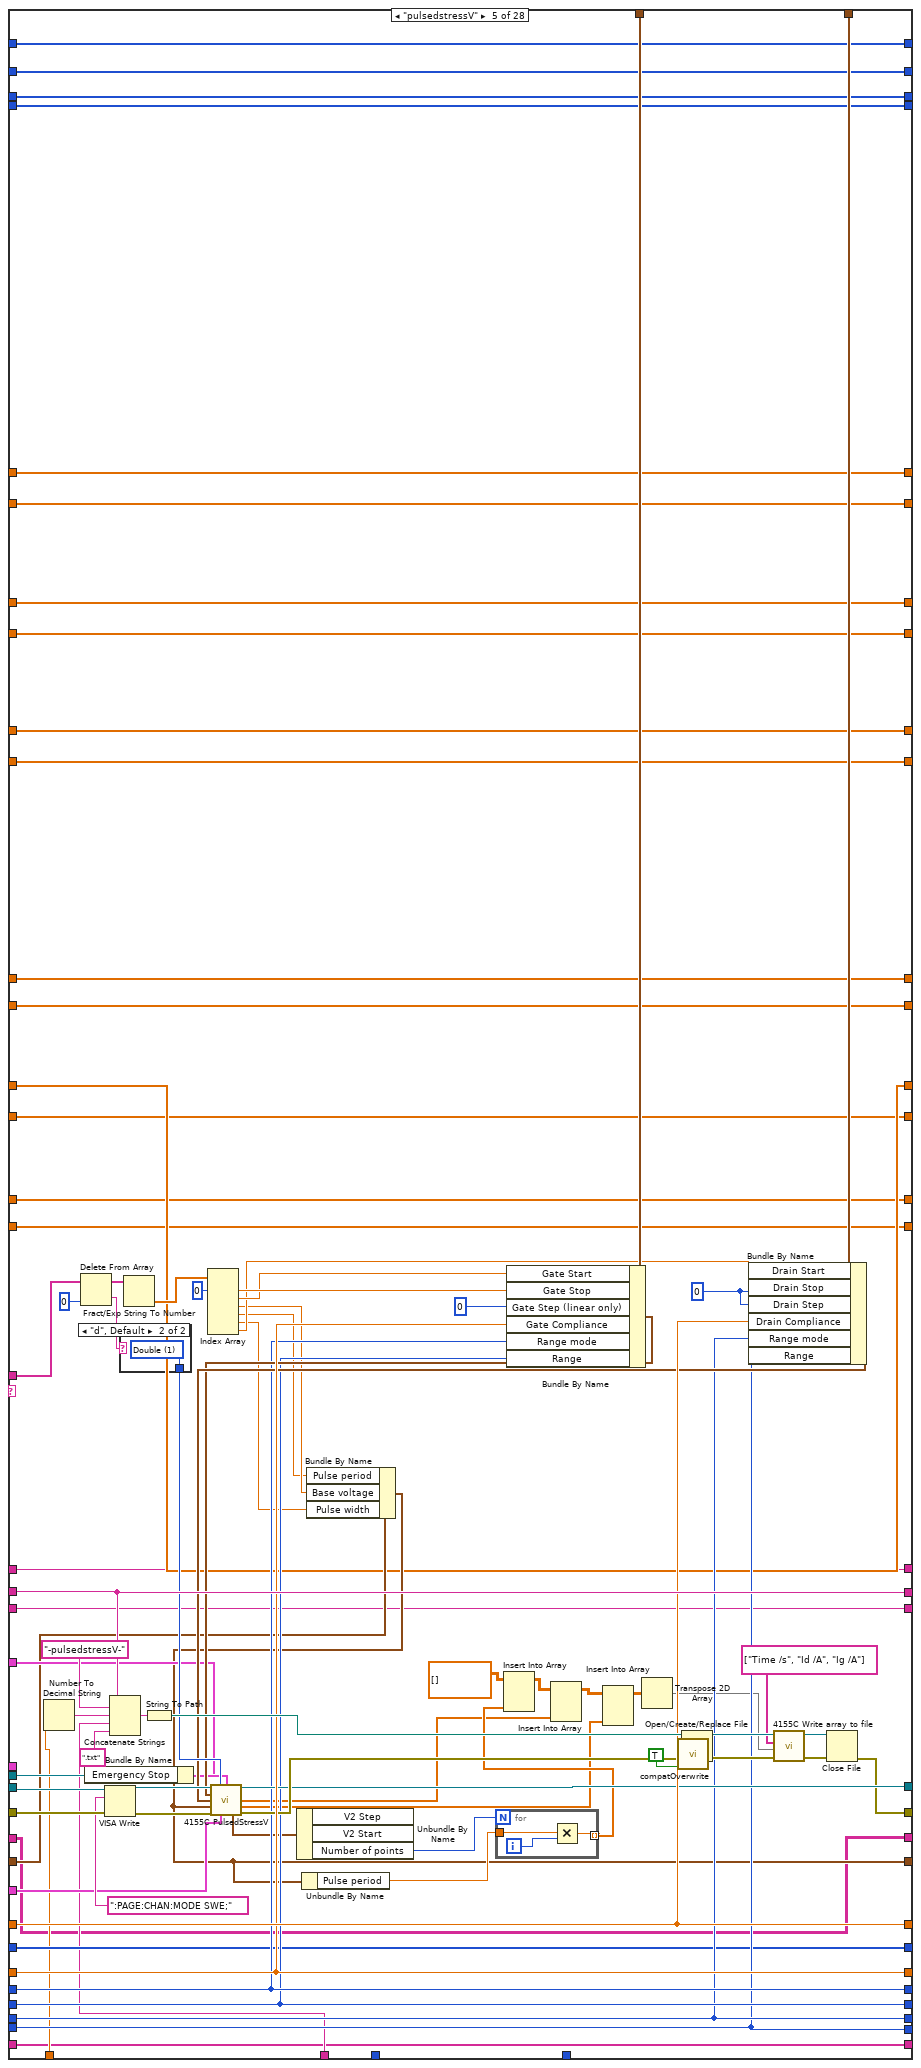
[diagram p10: hidden frame]
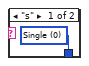
[diagram p11: hidden frame]
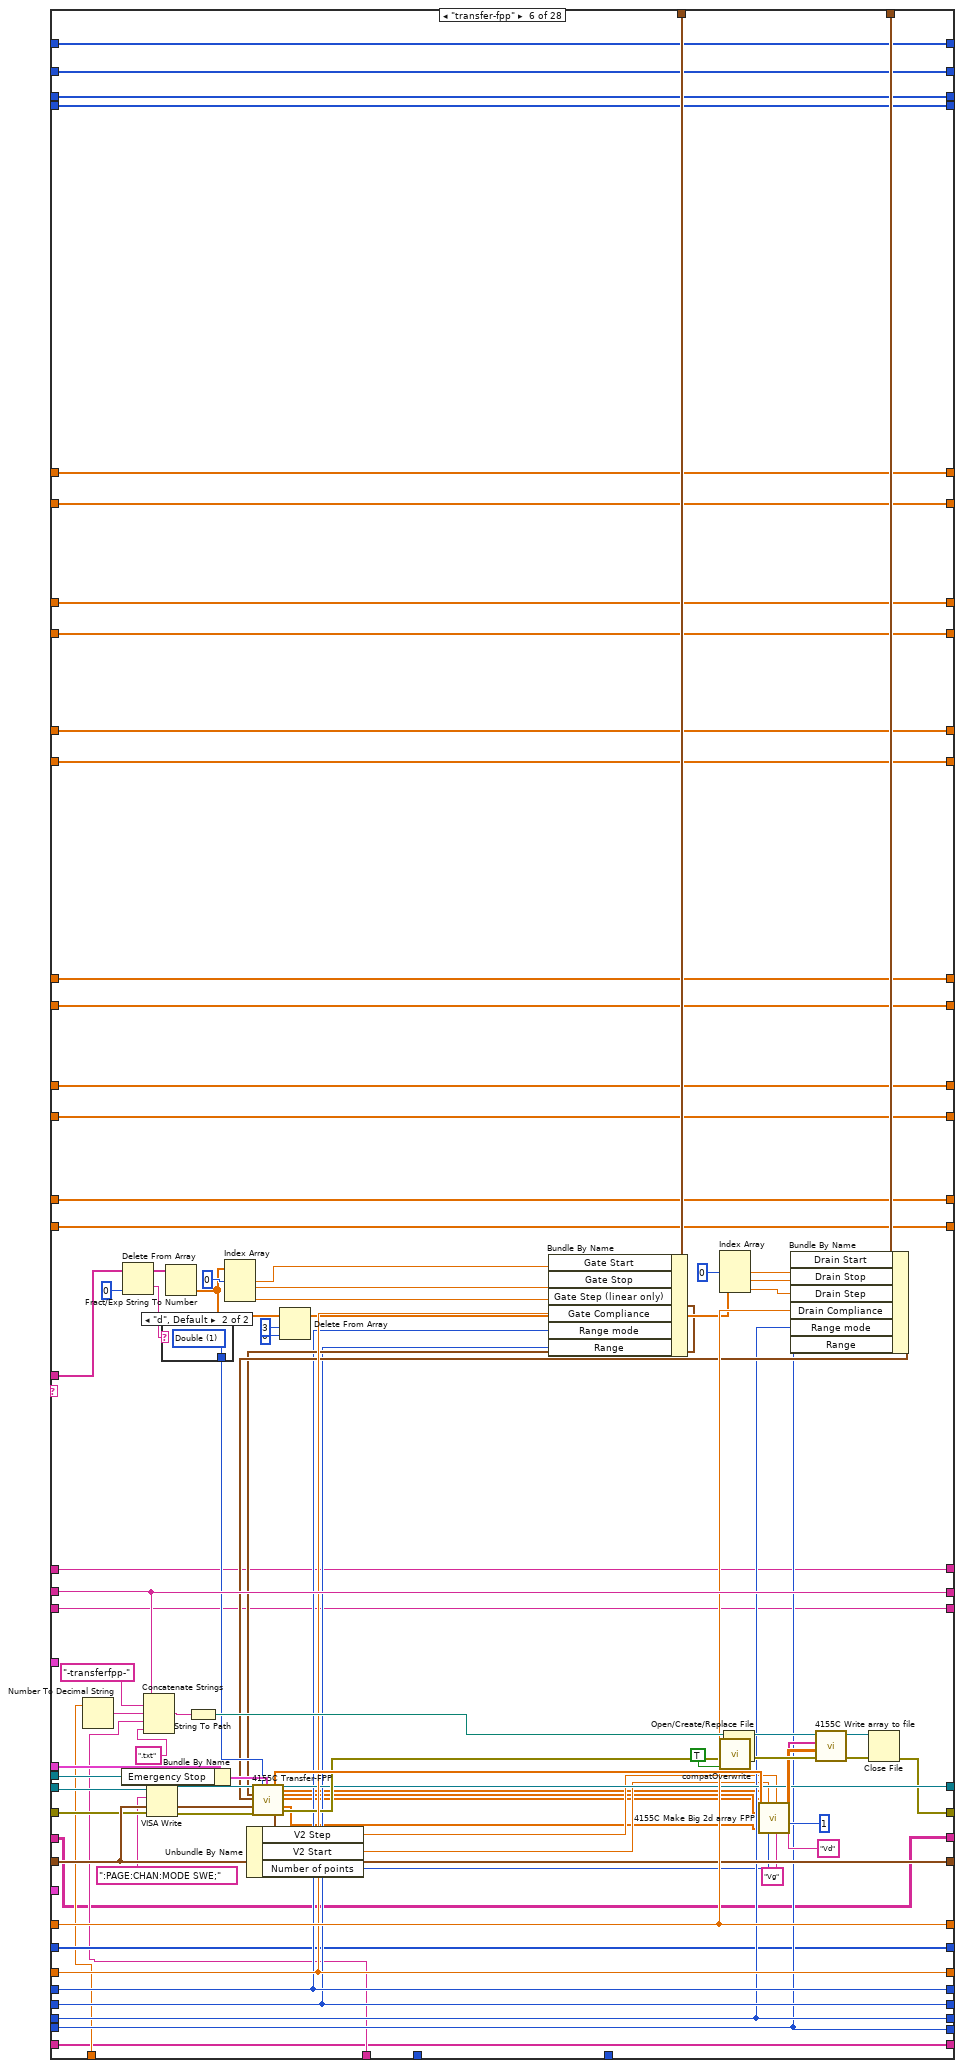
[diagram p12: hidden frame]
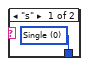
[diagram p13: hidden frame]
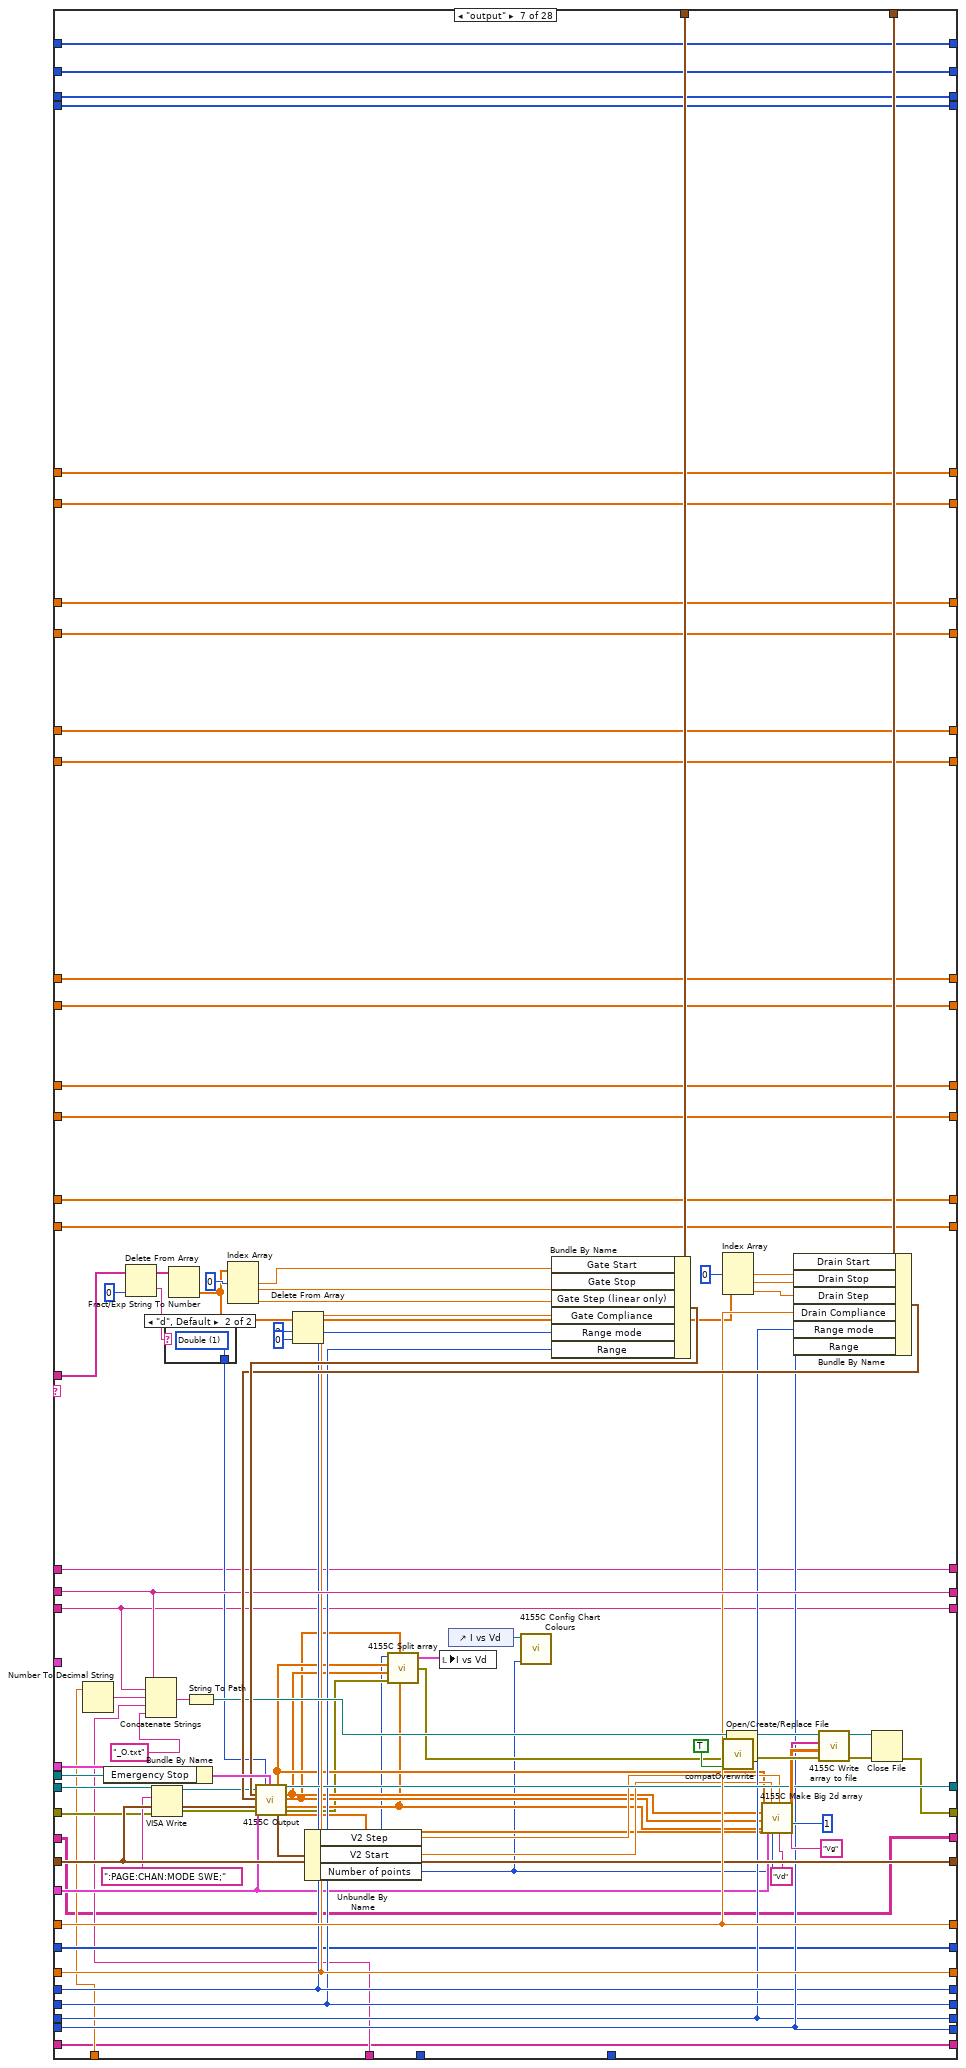
[diagram p14: hidden frame]
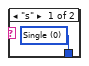
[diagram p15: hidden frame]
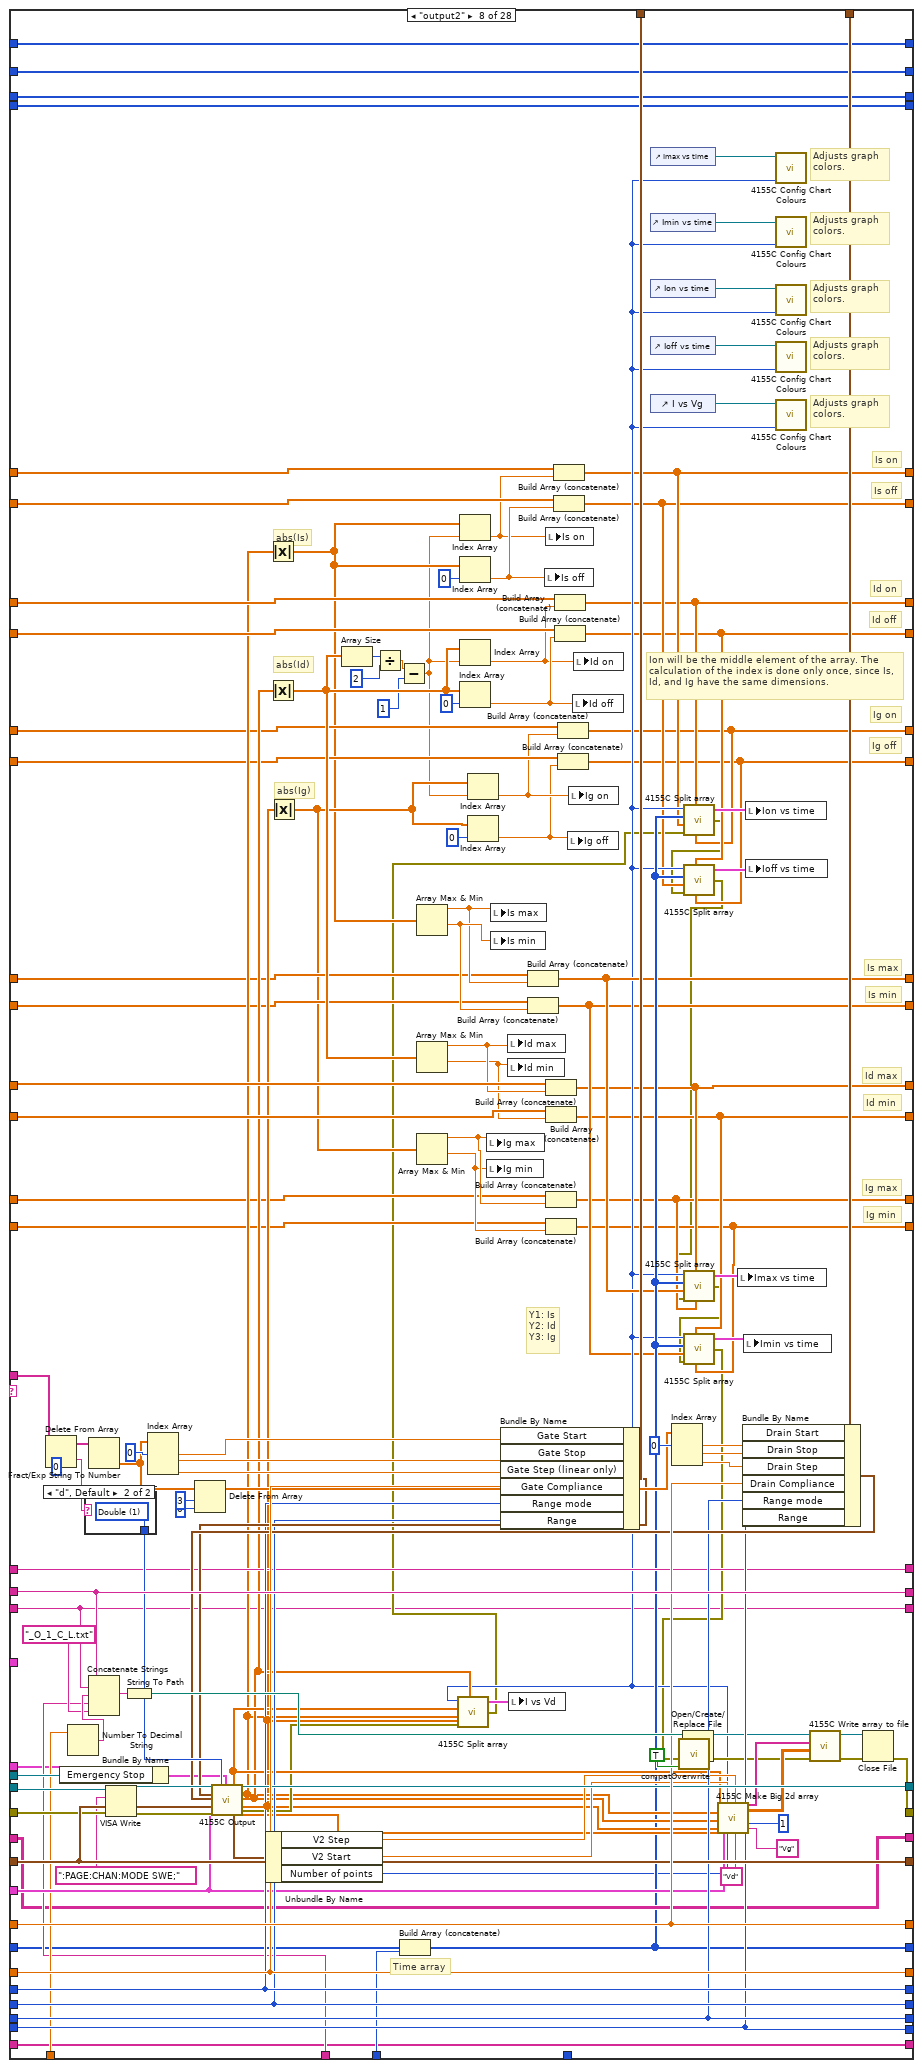
[diagram p16: hidden frame]
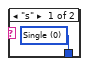
[diagram p17: hidden frame]
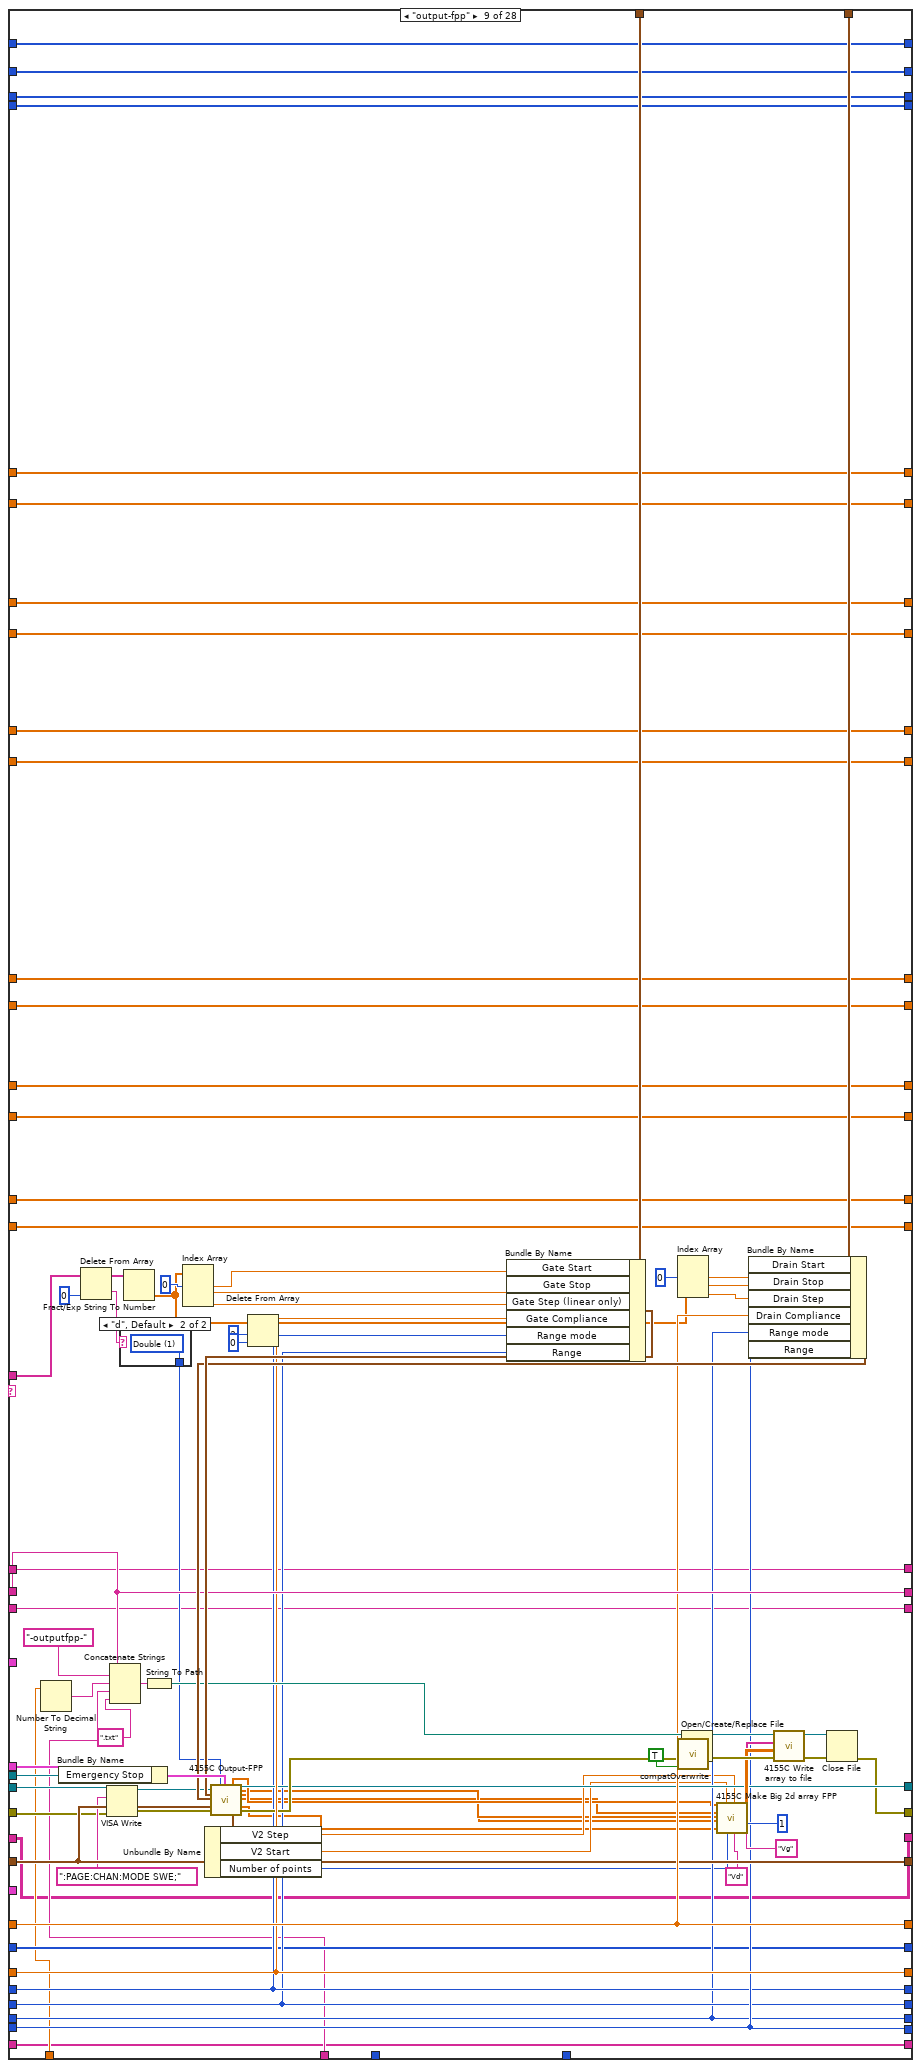
[diagram p18: hidden frame]
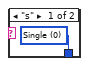
[diagram p19: hidden frame]
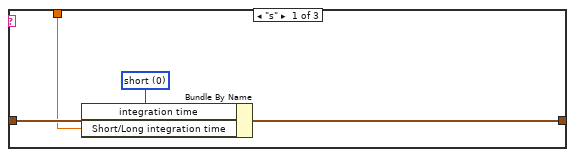
[diagram p20: hidden frame]
diagram:
  w51 = u16 1 items=["Reset All", "Partial reset"] ("Type of reset")
  # "Change from previous version:\n\n- Corrected bug of \"itime\" command. The command did not allow for settting the integration time value, it allowed to set the category of the integration time (short, medium, long). If the time value was beyond the range of the category, then the SPA used the closest value allowed, whilst staying in the category. \n\nSo, if the integration time was changed to long, but the integration time value was a short one, then the SPA would measure using the minimum long integration time value and not the value that the user intended."
  # "This is a version specific to the SPM pump."
  # "I add 1 to both the \"total lines\" and the \"line running\" indicators because i and N begin from 0, and the script lines begin from 1."
  # "Bugs:\n\n- If using the \"filename\" command, keep in mind that the arrays of the time-dependent data are not re-initialized inbetween filename changes. \n\n- Do not connect the \"error\" wire of a Split block if it has unconnected terminals! It will halt the program."
  # "Array size"
  # "%s option converts a spreadsheet string to an array of strings."
  # "0: No of rows of array\n1: No of cols"
  # "Dimitrios Simatos\nv. 5.8"
  # "Changes from original textcontrol.vi:\n\n- Timestamp appears in filename.\n- (Only) transfer and output curves are plotted.\n- Communication with serial port.\n- Can execute any command, as all pattern matching functions were replaced. Previously, commands with special LabVIEW characters could not be executed.\n- Replaced write to file function with write to text file.\n- Replaced while loop with for loop.\n- Replaced 4155C \"Save File\" function and now the vi can save time-dependent variables.\n- Added clock with start time control and various units.\n- Changed filepath in which the program is saved.\n- Added a serial output log that keeps a history.\n- Tab control.\n- Addition of specialized serial read/write file for the SPM OEM pump.\n- Added halt and hard stop.\n- Imax, Imin, Ion, and Ioff are now saved for all Is, Id, and Ig.\n- Output curves are taken into account in Imax-Imin-Ion-Ioff plots."
  # "Search and replace LF with EOL"
  n1 = Equal?(x="integration time", y=u32 0) -> (x = y?=w52:bool)
  n2 = Select(t="Integration time (short)", s=w52, f="Integration time (long)") -> (s? t:f=w1:dbl)
  n3 = Bundle By Name(cluster="Timings (overwritten by the Front Panel)", "integration time"="integration time", "Short/Long integration time"=w1) -> (w44:T5)
  n4 = call "4155C Get Filename.vi"("error in (no error)"=errorcluster {"status"=FALSE, "code"=0, "source"=""}) -> ("error out"=w46:errorcluster, "path"=w21:path)  [unwired: 2 in, 1 out]
  "Path" <- w21
  n5 = Path To String(path=w21) -> (string=w22:string)
  n6 = Search and Replace String(replace all?=TRUE ("replace all? (F)"), input string="Script", search string="\n", replace string="\r\n") -> (result string=w34:string)  [unwired: 4 in, 3 out]
  n7 = Match Pattern(string=w22, regular expression=".txt") -> (before substring=w17:string)  [unwired: 1 in, 3 out]
  n8 = Concatenate Strings(w17, "Suffix (script)") -> (w16:string)
  n9 = call "4155C Initialise.vi"("VISA resource name in"=refnum<visa-resource-name> "GPIB0::14::INSTR", "Reset"="Full Reset", "Type of reset"=w51, "error in (no error)"=w46, "VISA Timeout Value"=u32 10000) -> ("VISA Resource Name out"=w45:refnum<visa-resource-name>, "error out"=w14:errorcluster)
  n10 = Spreadsheet String To Array(delimiter (Tab)="\r\n", format string="%s", spreadsheet string="Script", array type (2D Dbl)="") -> (array=w25:string[][])
  n11 = Array Size(array=w25) -> (size(s)=w29:i32[])
  n12 = Initialize Array("") -> (w6:string[])  [unwired: 1 in]
  n13 = String To Path(string=w16) -> (path=w15:path)
  n14 = Initialize Array(0 ("element")) -> (w8:i32[])  [unwired: 1 in]
  n15 = Initialize Array("") -> (w4:string[][])  [unwired: 2 in]
  n16 = Initialize Array(0.0 ("element")) -> (w10:dbl[])  [unwired: 1 in]
  n17 = Index Array(array=w29, index=0) -> (element=w27:i32)
  n18 = Write to Text File(file (use dialog)=w15, text=w34, error in=w14) -> (error out=w13:errorcluster)  [unwired: 1 in, 2 out]
  n19 = for {
    N: w27 -> [w165]
    tunnel: "SMU4" -> [w201]
    shift-left: "Source/Drain Range" -> [w206]
    shift-right: [w202] -> _
    shift-left: "Source/Drain\nRange mode" -> [w207]
    shift-right: [w203] -> _
    shift-left: "Gate Range" -> [w208]
    shift-right: [w204] -> _
    shift-left: "Gate Range\nmode" -> [w209]
    shift-right: [w205] -> _
    shift-left: "Gate: Compliance" -> [w218]
    shift-right: [w214] -> _
    shift-left: "Drain: Compliance" -> [w219]
    shift-right: [w215] -> _
    shift-left: w44 -> [w220]
    shift-right: [w216] -> w2
    shift-left: w13 -> [w221]
    shift-right: [w111] -> w20
    shift-left: w45 -> [w222]
    shift-right: [w217] -> _
    shift-left: w17 -> [w223]
    shift-right: [w115] -> _
    tunnel: "Panel Controls 2" -> [w200]
    shift-right: [w73] -> _
    shift-left: w10 -> [w199]
    shift-right: [w135] -> _
    shift-left: _ -> [w195]
    tunnel: w25 -> [w194] mode=indexing
    shift-right: [w72] -> _
    shift-left: w10 -> [w171]
    shift-right: [w105] -> _
    shift-left: w6 -> [w157]
    shift-right: [w136] -> _
    shift-left: w8 -> [w152]
    shift-right: [w117] -> _
    shift-left: w8 -> [w151]
    shift-right: [w150] -> _
    shift-left: "" -> [w149]
    shift-right: [w110] -> _
    shift-left: w8 -> [w132]
    shift-right: [w109] -> _
    shift-left: w8 -> [w116]
    shift-right: [w106] -> _
    shift-left: w4 -> [w108]
    shift-right: [w66] -> _
    shift-left: w10 -> [w94]
    shift-right: [w67] -> _
    shift-left: w10 -> [w93]
    shift-right: [w71] -> _
    shift-left: w10 -> [w82]
    shift-right: [w70] -> _
    shift-left: w10 -> [w81]
    shift-right: [w64] -> _
    shift-left: w10 -> [w80]
    shift-right: [w74] -> _
    shift-left: w10 -> [w79]
    shift-right: [w65] -> _
    shift-left: w10 -> [w78]
    shift-right: [w63] -> _
    shift-left: w10 -> [w77]
    shift-right: [w69] -> _
    shift-left: w10 -> [w76]
    shift-right: [w68] -> _
    shift-left: w10 -> [w75]
    shift-right: [w58] -> _
    shift-left: "Filename (variable part)" -> [w57]
    i -> [w160]
    w96 = "Time (Minutes)" ("element")
    # "Filename prefix"
    # "Is off"
    # "Is on"
    # "Ig off"
    # "Ig on"
    # "Is min"
    # "Is max"
    # "Ig min"
    # "Ig max"
    # "Id min"
    # "Id max"
    # "Id off"
    # "Id on"
    # "Pump status"
    # "Filepath and name"
    # "Pump status"
    # "Limit of command arguments (array columns). Raise if needed."
    # "Serial port data (string)"
    # "Serial port data (table)"
    # "Time array for valve position"
    # "Time array for absolute plunger position"
    # "Valve position"
    # "Absolute plunger position"
    # "Serial port data"
    # "For loop counter"
    # "<-----Equivalent to the 4155C \"Write\" subvi.----->"
    # "Headers"
    # "Save transfer curves in file."
    # "Filepath and name"
    # "Save time-dependent data."
    # "Use the time offset if your measurements do not start at t=0."
    # "Time for Imax, Imin, Ion, Ioff"
    # "Rest of elements of command"
    # "First element of command\n(case select)"
    n20 = Add(x=w160, y=1) -> (x+y=→"Line running":i32)
    n21 = Add(x=w165, y=1) -> (x+y=→"Total lines":i32)
    n22 = Index Array(array=w194, index=0 ("line index")) -> (element=w189:string)
    "Command running:" <- w189
    n23 = control-ref of="Interrupt run"() -> (w213:refnum<vi>)
    n24 = Spreadsheet String To Array(delimiter (Tab)=" ", format string="%s", spreadsheet string=w189, array type (2D Dbl)=string[] []) -> (array=w187:string[])
    n25 = Delete From Array(array=w187, index=0) -> (deleted portion=w95:string, array with subset deleted=w186:string[])  [unwired: 1 in]
    n26 = call "Elapsed Time"("Reset"="Reset", "Auto Reset"="Auto Reset") -> ("Elapsed Time (s)"=w196:dbl)  [unwired: 10 in, 7 out]
    n27 = case shown="0, Default" "Units" {
      tunnel: ["_sec" "_min" "_h"] -> w197
      tunnel: [w224 w228 w231] -> w167
      tunnel: w196 -> [w224 w227 w232]
      frame 0, Default {
      }
      frame 1 {
        n28 = Divide(x=w227, y=60.0) -> (x/y=w228:dbl)
      }
      frame 2 {
        n29 = Divide(x=w232, y=3600.0) -> (x/y=w231:dbl)
      }
    }
    n30 = Add(x=w167, y="Time Offset") -> (x+y=w166:dbl)
    n31 = To Long Integer(number=w166) -> (32bit integer=w133:i32)
    "Elapsed Time" <- w133
    n32 = case shown="\"itime\"" w95 {
      tunnel: w186 -> [w269 w307 w344 w476 w500 w646 w740 w892 w970 w997 w1077 w1123 w1167 w1207 w1240 _ _ w1401 w1481 _ w1584 w1647 w1708 w1797 w1878 w1917 w1987 w2041]
      tunnel: w223 -> [w264 w303 w342 w483 w565 w654 w747 w899 w978 w1020 w1066 w1115 w1160 w1201 w1233 w1271 w1332 w1379 w1463 w1513 w1571 w1634 w1696 w1791 w1874 w1919 w1989 w2043]
      tunnel: w222 -> [w263 w302 w333 w454 w550 w623 w716 w870 w946 w1021 w1067 w1116 w1161 w1202 w1234 w1276 w1334 w1407 w1487 w1517 w1590 w1653 w1714 w1803 w1832 w1923 w1993 w2045]
      tunnel: w221 -> [w262 w301 w332 w453 w549 w622 w713 w869 w943 w1022 w1068 w1117 w1162 w1203 w1235 w1275 w1305 w1406 w1486 w1516 w1589 w1652 w1713 w1802 w1831 w1922 w1992 w2046]
      tunnel: w220 -> [w261 w300 w341 w479 w525 w650 w743 w895 w974 w1030 w1076 w1114 w1159 w1200 w1232 w1274 w1329 w1370 w1455 w1522 w1564 w1627 w1689 w1790 w1873 w1924 w1994 w2048]
      tunnel: w219 -> [w260 w299 w340 w481 w563 w652 w745 w897 w976 w1029 w1075 w1122 w1166 w1206 w1239 w1273 w1314 w1405 w1485 w1525 w1588 w1651 w1712 w1801 w1882 w1925 w1995 w2049]
      tunnel: w218 -> [w259 w298 w339 w480 w562 w651 w744 w896 w975 w1028 w1074 w1121 w1165 w1205 w1238 w1272 w1315 w1380 w1464 w1524 w1572 w1635 w1697 w1792 w1875 w1927 w1996 w2051]
      tunnel: [w263 w302 w331 w478 w560 w648 w742 w894 w972 w1021 w1067 w1116 w1161 w1202 w1234 w1276 w1334 w1371 w1437 w1515 w1565 w1628 w1690 w1743 w1834 w1923 w1993 w2045] -> w217
      tunnel: [w262 w301 w330 w477 w559 w647 w741 w893 w971 w1022 w1068 w1117 w1162 w1203 w1235 w1275 w1304 w1381 w1438 w1514 w1573 w1636 w1698 w1742 w1833 w1921 w1991 w2046] -> w131
      tunnel: [w261 w300 w341 w479 w521 w650 w743 w895 w974 w1023 w1069 w1114 w1159 w1200 w1232 w1274 w1329 w1370 w1455 w1522 w1564 w1627 w1689 w1790 w1873 w1924 w1994 w2048] -> w216
      tunnel: [w260 w299 w340 w481 w563 w652 w745 w897 w976 w1029 w1075 w1122 w1166 w1206 w1239 w1273 w1314 w1405 w1485 w1525 w1588 w1651 w1712 w1801 w1882 w1925 w1995 w2049] -> w215
      tunnel: [w259 w298 w339 w480 w562 w651 w744 w896 w975 w1028 w1074 w1121 w1165 w1205 w1238 w1272 w1315 w1380 w1464 w1524 w1572 w1635 w1697 w1792 w1875 w1927 w1996 w2051] -> w214
      tunnel: [w264 w303 w342 w483 w565 w654 w747 w899 w978 w1020 w1066 w1115 w1160 w1201 w1233 w1271 w1332 w1379 w1463 w1513 w1571 w1634 w1696 w1791 w1874 w1919 w1989 w2043] -> w115
      tunnel: w213 -> [_ _ _ w485 w569 w659 w750 w901 w982 _ _ _ _ _ _ _ _ w1376 w1460 _ w1570 w1633 w1695 w1763 w1850 _ _ _]
      tunnel: "Gate" -> [_ _ _ w463 w553 w633 w727 w879 w957 _ _ _ _ _ _ _ _ _ _ _ _ _ _ _ _ _ _ _]
      tunnel: "Drain 2" -> [_ _ _ w462 w552 w632 w726 w878 w956 _ _ _ _ _ _ _ _ _ _ _ _ _ _ _ _ _ _ _]
      tunnel: "Panel Controls" -> [_ _ _ _ _ w631 w725 w763 w955 _ _ _ _ _ _ _ _ _ _ _ _ _ _ _ _ _ _ _]
      tunnel: w209 -> [w258 w297 w338 w447 w543 w616 w711 w863 w941 w1027 w1073 _ w1158 w1199 w1231 w1270 w1316 w1366 w1451 w1518 w1560 w1623 w1685 w1786 w1869 w1928 w1997 w2052]
      tunnel: w208 -> [w257 w296 w337 w446 w542 w615 w710 w862 w940 w1026 w1072 w1120 _ w1190 w1237 w1269 w1317 w1367 w1452 w1519 w1561 w1624 w1686 w1787 w1870 w1929 w1998 w2053]
      tunnel: w207 -> [w256 w295 w336 w445 w541 w614 w709 w861 w939 w1025 w1071 w1119 w1164 w1204 _ w1268 w1318 w1368 w1453 w1520 w1562 w1625 w1687 w1788 w1871 w1930 w1999 w2054]
      tunnel: w206 -> [w255 w294 w335 w444 w540 w613 w712 w860 w942 w1024 w1070 w1118 w1163 _ w1236 w1267 w1319 w1369 w1454 w1521 w1563 w1626 w1688 w1789 w1872 w1931 w2000 w2055]
      tunnel: [w258 w297 w338 w447 w543 w616 w711 w863 w941 w1027 w1073 w1113 w1158 w1199 w1231 w1270 w1316 w1366 w1451 w1518 w1560 w1623 w1685 w1786 w1869 w1928 w1997 w2052] -> w205
      tunnel: [w257 w296 w337 w446 w542 w615 w710 w862 w940 w1026 w1072 w1120 w1150 w1190 w1237 w1269 w1317 w1367 w1452 w1519 w1561 w1624 w1686 w1787 w1870 w1929 w1998 w2053] -> w204
      tunnel: [w256 w295 w336 w445 w541 w614 w709 w861 w939 w1025 w1071 w1119 w1164 w1204 w1230 w1268 w1318 w1368 w1453 w1520 w1562 w1625 w1687 w1788 w1871 w1930 w1999 w2054] -> w203
      tunnel: [w255 w294 w335 w444 w540 w613 w712 w860 w942 w1024 w1070 w1118 w1163 w1191 w1236 w1267 w1319 w1369 w1454 w1521 w1563 w1626 w1688 w1789 w1872 w1931 w2000 w2055] -> w202
      tunnel: w201 -> [_ _ _ w439 w537 _ w705 w855 _ _ _ _ _ _ _ _ _ _ _ _ _ _ _ _ _ _ _ _]
      tunnel: w200 -> [_ _ _ w437 w536 _ _ _ _ _ _ _ _ _ _ _ _ _ _ _ _ _ _ _ _ _ _ _]
      tunnel: [w254 w290 w328 w365 w513 w603 w702 w782 w928 w1019 w1064 w1112 w1149 w1189 w1229 w1266 w1300 w1358 w1416 w1512 w1549 w1616 w1679 w1740 w1827 w1920 w1990 w2060] -> w73
      tunnel: w199 -> [w254 w290 w328 w434 w513 w603 w702 w851 w928 w1019 w1064 w1112 w1149 w1189 w1229 w1266 w1300 w1358 w1416 w1512 w1549 w1616 w1679 w1740 w1827 w1920 w1990 w2060]
      tunnel: w166 -> [_ _ _ w431 w510 w601 w699 w848 w925 _ _ _ _ _ _ _ w1298 w1356 w1433 _ w1546 w1613 w1676 w1737 w1823 _ _ _]
      tunnel: w197 -> [_ _ _ w428 w509 w599 w698 w845 w924 _ _ _ _ _ _ _ w1296 w1354 w1432 _ w1545 w1612 w1675 w1736 w1824 _ w1958 _]
      tunnel: w133 -> [_ _ _ w423 _ _ _ w840 _ _ _ _ _ _ _ _ _ _ _ _ _ _ _ _ _ _ w1961 _]
      tunnel: [w253 w289 w327 w373 w512 w602 w701 w790 w927 w1018 w1063 w1111 w1148 w1188 w1228 w1265 w1299 w1357 w1435 w1511 w1548 w1615 w1678 w1739 w1826 w1926 w1970 w2050] -> w135
      tunnel: w195 -> [w253 w289 w327 w427 w512 w602 w701 w844 w927 w1018 w1063 w1111 w1148 w1188 w1228 w1265 w1299 w1357 w1435 w1511 w1548 w1615 w1678 w1739 w1826 w1926 w1970 w2050]
      tunnel: [w252 w288 w326 w364 w508 w598 w697 w781 w923 w1017 w1062 w1110 w1147 w1187 w1227 w1264 w1295 w1353 w1415 w1510 w1544 w1611 w1674 w1735 w1822 w1915 w1986 w2059] -> w72
      tunnel: w171 -> [w252 w288 w326 w421 w508 w598 w697 w838 w923 w1017 w1062 w1110 w1147 w1187 w1227 w1264 w1295 w1353 w1415 w1510 w1544 w1611 w1674 w1735 w1822 w1915 w1986 w2059]
      tunnel: [w251 w287 w325 w414 w507 w597 w687 w831 w922 w1016 w1061 w1109 w1146 w1186 w1226 w1263 w1294 w1352 w1431 w1509 w1543 w1610 w1673 w1734 w1821 w1914 w1985 w2056] -> w105
      tunnel: w157 -> [w251 w287 w325 w414 w507 w597 w687 w831 w922 w1016 w1061 w1109 w1146 w1186 w1226 w1263 w1294 w1352 w1431 w1509 w1543 w1610 w1673 w1734 w1821 w1913 w1959 w2056]
      tunnel: [w250 w286 w324 w413 w506 w596 w686 w830 w921 w1015 w1060 w1108 w1145 w1185 w1225 w1262 w1293 w1351 w1430 w1508 w1542 w1609 w1672 w1733 w1820 w1899 w1972 w2070] -> w136
      tunnel: w152 -> [w250 w286 w324 w413 w506 w596 w686 w830 w921 w1015 w1060 w1108 w1145 w1185 w1225 w1262 w1293 w1351 w1430 w1508 w1542 w1609 w1672 w1733 w1820 w1899 w1971 w2070]
      tunnel: [w249 w285 w323 w412 w505 w595 w685 w829 w920 w1014 w1059 w1107 w1144 w1184 w1224 w1261 w1292 w1350 w1429 w1507 w1541 w1608 w1671 w1732 w1819 w1898 w1954 w2072] -> w117
      tunnel: w151 -> [w249 w285 w323 w412 w505 w595 w685 w829 w920 w1014 w1059 w1107 w1144 w1184 w1224 w1261 w1292 w1350 w1429 w1507 w1541 w1608 w1671 w1732 w1819 w1898 w1952 w2072]
      tunnel: [w248 w284 w322 w411 w504 w594 w684 w828 w919 w1013 w1058 w1106 w1143 w1183 w1223 w1260 w1291 w1349 w1428 w1506 w1540 w1607 w1670 w1731 w1818 w1897 w1951 w2044] -> w150
      tunnel: w149 -> [w248 w284 w322 w411 w504 w594 w684 w828 w919 w1013 w1058 w1106 w1143 w1183 w1223 w1260 w1291 w1349 w1428 w1506 w1540 w1607 w1670 w1731 w1818 w1897 w1962 w2044]
      tunnel: w133 -> [_ _ _ _ _ _ _ _ _ _ _ _ _ _ _ _ _ _ _ _ _ _ _ _ _ _ w1950 _]
      tunnel: w132 -> [w247 w283 w321 w410 w503 w593 w683 w827 w918 w1012 w1057 w1105 w1142 w1182 w1222 w1259 w1290 w1348 w1427 w1505 w1539 w1606 w1669 w1730 w1817 w1896 w1949 w2071]
      tunnel: [w247 w283 w321 w410 w503 w593 w683 w827 w918 w1012 w1057 w1105 w1142 w1182 w1222 w1259 w1290 w1348 w1427 w1505 w1539 w1606 w1669 w1730 w1817 w1896 w1948 w2071] -> w110
      tunnel: [w246 w282 w320 w409 w502 w592 w682 w826 w917 w1011 w1056 w1104 w1141 w1181 w1221 w1258 w1289 w1347 w1426 w1504 w1538 w1605 w1668 w1729 w1816 w1895 w1947 w2069] -> w109
      tunnel: w116 -> [w246 w282 w320 w409 w502 w592 w682 w826 w917 w1011 w1056 w1104 w1141 w1181 w1221 w1258 w1289 w1347 w1426 w1504 w1538 w1605 w1668 w1729 w1816 w1895 w1946 w2069]
      tunnel: [w245 w281 w319 w408 w501 w591 w681 w825 w916 w1010 w1055 w1103 w1140 w1180 w1220 w1257 w1288 w1346 w1425 w1503 w1537 w1604 w1667 w1728 w1815 w1894 w1944 w2047] -> w106
      tunnel: w108 -> [w245 w281 w319 w408 w501 w591 w681 w825 w916 w1010 w1055 w1103 w1140 w1180 w1220 w1257 w1288 w1346 w1425 w1503 w1537 w1604 w1667 w1728 w1815 w1894 w1943 w2047]
      tunnel: [w243 w279 w317 w358 w498 w589 w679 w775 w914 w1008 w1054 w1102 w1138 w1178 w1218 w1255 w1286 w1345 w1424 w1502 w1536 w1603 w1665 w1727 w1814 w1893 w1942 w2065] -> w66
      tunnel: w94 -> [w243 w279 w317 w404 w498 w589 w679 w821 w914 w1008 w1054 w1102 w1138 w1178 w1218 w1255 w1286 w1345 w1424 w1502 w1536 w1603 w1665 w1727 w1814 w1893 w1942 w2065]
      tunnel: [w244 w280 w318 w359 w499 w590 w680 w776 w915 w1009 w1053 w1101 w1139 w1179 w1219 w1256 w1287 w1344 w1423 w1501 w1535 w1602 w1666 w1726 w1813 w1892 w1941 w2066] -> w67
      tunnel: w93 -> [w244 w280 w318 w403 w499 w590 w680 w820 w915 w1009 w1053 w1101 w1139 w1179 w1219 w1256 w1287 w1344 w1423 w1501 w1535 w1602 w1666 w1726 w1813 w1892 w1941 w2066]
      tunnel: [w236 w272 w310 w363 w495 w587 w677 w780 w912 w1001 w1051 w1099 w1136 w1176 w1216 w1253 w1279 w1337 w1414 w1500 w1528 w1595 w1658 w1719 w1808 w1885 w1940 w2058] -> w71
      tunnel: w82 -> [w236 w272 w310 w393 w495 w587 w677 w810 w912 w1001 w1051 w1099 w1136 w1176 w1216 w1253 w1279 w1337 w1414 w1500 w1528 w1595 w1658 w1719 w1808 w1885 w1940 w2058]
      tunnel: [w235 w271 w309 w362 w496 w588 w678 w779 w913 w1000 w1052 w1100 w1137 w1177 w1217 w1254 w1278 w1336 w1413 w1499 w1527 w1594 w1657 w1718 w1807 w1884 w1939 w2057] -> w70
      tunnel: w81 -> [w235 w271 w309 w392 w496 w588 w678 w809 w913 w1000 w1052 w1100 w1137 w1177 w1217 w1254 w1278 w1336 w1413 w1499 w1527 w1594 w1657 w1718 w1807 w1884 w1939 w2057]
      tunnel: [w238 w274 w312 w368 w494 w585 w675 w785 w910 w1006 w1049 w1097 w1134 w1174 w1214 w1251 w1281 w1339 w1418 w1494 w1530 w1597 w1660 w1721 w1806 w1889 w1937 w2062] -> w64
      tunnel: w80 -> [w238 w274 w312 w389 w494 w585 w675 w806 w910 w1006 w1049 w1097 w1134 w1174 w1214 w1251 w1281 w1339 w1418 w1494 w1530 w1597 w1660 w1721 w1806 w1889 w1937 w2062]
      tunnel: [w237 w273 w311 w366 w497 w586 w676 w783 w911 w1007 w1050 w1098 w1135 w1175 w1215 w1252 w1280 w1338 w1417 w1493 w1529 w1596 w1659 w1720 w1805 w1888 w1938 w2061] -> w74
      tunnel: w79 -> [w237 w273 w311 w388 w497 w586 w676 w805 w911 w1007 w1050 w1098 w1135 w1175 w1215 w1252 w1280 w1338 w1417 w1493 w1529 w1596 w1659 w1720 w1805 w1888 w1938 w2061]
      tunnel: [w240 w276 w314 w357 w493 w583 w673 w774 w908 w1004 w1047 w1095 w1132 w1172 w1212 w1249 w1283 w1341 w1420 w1496 w1532 w1599 w1662 w1723 w1810 w1891 w1935 w2064] -> w65
      tunnel: w78 -> [w240 w276 w314 w385 w493 w583 w673 w802 w908 w1004 w1047 w1095 w1132 w1172 w1212 w1249 w1283 w1341 w1420 w1496 w1532 w1599 w1662 w1723 w1810 w1891 w1935 w2064]
      tunnel: [w239 w275 w313 w356 w492 w584 w674 w773 w909 w1005 w1048 w1096 w1133 w1173 w1213 w1250 w1282 w1340 w1419 w1495 w1531 w1598 w1661 w1722 w1809 w1890 w1936 w2063] -> w63
      tunnel: w77 -> [w239 w275 w313 w384 w492 w584 w674 w801 w909 w1005 w1048 w1096 w1133 w1173 w1213 w1250 w1282 w1340 w1419 w1495 w1531 w1598 w1661 w1722 w1809 w1890 w1936 w2063]
      tunnel: [w242 w278 w316 w361 w491 w581 w671 w778 w906 w1002 w1045 w1093 w1130 w1170 w1210 w1247 w1285 w1343 w1422 w1498 w1534 w1601 w1664 w1725 w1812 w1887 w1933 w2068] -> w69
      tunnel: w76 -> [w242 w278 w316 w381 w491 w581 w671 w798 w906 w1002 w1045 w1093 w1130 w1170 w1210 w1247 w1285 w1343 w1422 w1498 w1534 w1601 w1664 w1725 w1812 w1887 w1933 w2068]
      tunnel: [w241 w277 w315 w360 w490 w582 w672 w777 w907 w1003 w1046 w1094 w1131 w1171 w1211 w1248 w1284 w1342 w1421 w1497 w1533 w1600 w1663 w1724 w1811 w1886 w1934 w2067] -> w68
      tunnel: w75 -> [w241 w277 w315 w380 w490 w582 w672 w797 w907 w1003 w1046 w1094 w1131 w1171 w1211 w1248 w1284 w1342 w1421 w1497 w1533 w1600 w1663 w1724 w1811 w1886 w1934 w2067]
      tunnel: w57 -> [w234 w270 w308 w347 w489 w580 w670 w764 w905 w999 w1044 w1092 w1129 w1169 w1209 w1246 w1277 w1335 w1412 w1492 w1526 w1593 w1656 w1717 w1804 w1883 w1932 _]
      tunnel: [w234 w270 w308 w347 w489 w580 w670 w764 w905 w999 w1044 w1092 w1129 w1169 w1209 w1246 w1277 w1335 w1412 w1492 w1526 w1593 w1656 w1717 w1804 w1883 w1932 w2040] -> w58
      frame "wait" {
        n33 = Index Array(array=w269, index=0 ("Index")) -> (element=w267:string)
        n34 = Decimal String To Number(string=w267, default (0L)=u32 0) -> (number=w266:u32)  [unwired: 1 in, 1 out]
        n35 = Wait (ms)(milliseconds to wait=w266) -> ()  [unwired: 1 out]
      }
      frame "wait-min" {
        n36 = Index Array(array=w307, index=0 ("Index")) -> (element=w305:string)
        n37 = Decimal String To Number(string=w305, default (0L)=u32 0) -> (number=w293:u32)  [unwired: 1 in, 1 out]
        n38 = Multiply(x=w293, y=u32 60000) -> (x*y=w292:u32)
        n39 = Wait (ms)(milliseconds to wait=w292) -> ()  [unwired: 1 out]
      }
      frame "standby" {
        n40 = Index Array(array=w344, index=0 ("Index")) -> (element=w334:string)
        n41 = case shown="\"off\", Default" w334 {
          tunnel: [":PAGE:SCON:STAN 0" ":PAGE:SCON:STAN 1"] -> w329
          frame "off", Default {
          }
          frame "on" {
          }
        }
        n42 = VISA Write(VISA resource name=w333, write buffer=w329, error in (no error)=w332) -> (VISA resource name out=w331:refnum<visa-resource-name>, error out=w330:errorcluster)  [unwired: 1 out]
      }
      frame "transfer" {
        # "Adjusts graph colors."
        # "Adjusts graph colors."
        # "Is off"
        # "Is on"
        # "Ion will be the middle element of the array. The calculation of the index is done only once, since Is, Id, and Ig have the same dimensions."
        # "Ig off"
        # "Ig on"
        # "Is min"
        # "Is max"
        # "Ig min"
        # "Ig max"
        # "abs(Ig)"
        # "abs(Is)"
        # "Id min"
        # "Id max"
        # "Y1: Is\nY2: Id\nY3: Ig"
        # "abs(Id)"
        # "Adjusts graph colors."
        # "Adjusts graph colors."
        # "Id off"
        # "Id on"
        # "Adjusts graph colors."
        # "Time array"
        n43 = Delete From Array(array=w476, index=0 ("Index")) -> (deleted portion=w474:string, array with subset deleted=w473:string[])  [unwired: 1 in]
        n44 = Bundle By Name(cluster=w437, "Emergency Stop"=w485) -> (w438:T2)
        n45 = Number To Decimal String(number=w431) -> (decimal integer string=w430:string)  [unwired: 1 in]
        n46 = case shown="\"d\", Default" w474 {
          tunnel: [w487 w488] -> w472
          frame "s" {
            w487 = u16 0 items=["Single", "Double"] ("sweep mode")
          }
          frame "d", Default {
            w488 = u16 1 items=["Single", "Double"] ("sweep mode")
          }
        }
        n47 = Fract/Exp String To Number(string=w473) -> (number=w458:dbl[])  [unwired: 3 in, 1 out]
        n48 = Concatenate Strings(w483, w347, w430, w428, "_T_1_C_L.txt" ("Suffix (transfer)")) -> (w484:string)
        n49 = VISA Write(VISA resource name=w454, write buffer=":PAGE:CHAN:MODE SWE;" ("write buffer (\"\")"), error in (no error)=w453) -> (VISA resource name out=w451:refnum<visa-resource-name>, error out=w452:errorcluster)  [unwired: 1 out]
        n50 = String To Path(string=w484) -> (path=w482:path)
        n51 = Index Array(array=w458, index #1=0 ("Index")) -> (element #1=w471:dbl, element #2=w470:dbl, element #3=w469:dbl)  [unwired: 2 in]
        n52 = Delete From Array(array=w458, length=3 ("Length"), index=0 ("Index")) -> (array with subset deleted=w456:dbl[])  [unwired: 1 out]
        n53 = Build Array (concatenate)(w427, w423) -> (w373:i32[])
        n54 = Bundle By Name(cluster=w463, "Gate Start"=w471, "Gate Stop"=w470, "Gate Step (linear only)"=w469, "Gate Compliance"=w480, "Range mode"=w447, "Range"=w446) -> (w448:T6)
        n55 = control-ref of="Imax vs time"() -> (w402:refnum<vi>)
        n56 = control-ref of="Imin vs time"() -> (w401:refnum<vi>)
        n57 = control-ref of="Ion vs time"() -> (w370:refnum<vi>)
        n58 = control-ref of="Ioff vs time"() -> (w369:refnum<vi>)
        n59 = control-ref of="I vs Vg"() -> (w432:refnum<vi>)
        n60 = Index Array(array=w456, index #1=0 ("Index")) -> (element #1=w466:dbl, element #2=w465:dbl, element #3=w464:dbl)  [unwired: 2 in]
        n61 = call <vilib>:"compatOverwrite.vi"("overwrite (F)"=TRUE) -> ("overwrite?"=w436:T8)
        n62 = Bundle By Name(cluster=w462, "Drain Start"=w466, "Drain Stop"=w465, "Drain Step"=w464, "Drain Compliance"=w481, "Range mode"=w445, "Range"=w444) -> (w449:T7)
        n63 = call "4155C Transfer.vi"("VISA resource name in"=w451, "Gate"=w448, "Drain"=w449, "Timings"=w479, "error in (no error)"=w452, "SMU4"=w439, "sweep mode"=w472, "Panel Controls"=w438) -> ("VG"=w435:dbl[], "Outparams"=w443:T9, "VISA Resource Name out"=w478:refnum<visa-resource-name>, "IS"=w398:dbl[], "ID"=w400:dbl[], "IG"=w397:dbl[], "error out"=w424:errorcluster, "SMU4"=w440:dbl[])  [unwired: 12 in]
        n64 = Unbundle By Name(w443) -> ("V2 Step"=w442:dbl, "V2 Start"=w441:dbl, "Number of points"=w367:i32)
        n65 = Absolute Value(x=w398) -> (abs(x)=w383:dbl[])
        n66 = Absolute Value(x=w400) -> (abs(x)=w399:dbl[])
        n67 = Absolute Value(x=w397) -> (abs(x)=w386:dbl[])
        n68 = Array Size(array=w399) -> (size(s)=w407:i32)
        n69 = Divide(x=w407, y=2) -> (x/y=w350:dbl)
        n70 = Subtract(x=w350, y=1) -> (x-y=w349:dbl)
        n71 = Array Max & Min(array=w383) -> (max value=w390:dbl, min value=w391:dbl)  [unwired: 2 out]
        n72 = Array Max & Min(array=w399) -> (max value=w433:dbl, min value=w396:dbl)  [unwired: 2 out]
        n73 = Array Max & Min(array=w386) -> (max value=w395:dbl, min value=w394:dbl)  [unwired: 2 out]
        n74 = call "4155C Split array.vi"("Number of VAR2 steps"=w367, "Y2 data in"=w400, "X data in"=w435, "Y1 data in"=w398, "Y3 data in"=w397, "error in (no error)"=w424) -> ("Array of clusters"=w426:cluster{"Y data in":dbl[], "X data in":dbl[]}[], "error out"=w355:errorcluster)  [unwired: 1 in]
        n75 = Index Array(array=w383, index=w349) -> (element=w374:dbl)
        n76 = Index Array(array=w383, index=0) -> (element=w375:dbl)
        n77 = Index Array(array=w399, index=w349) -> (element=w376:dbl)
        n78 = Index Array(array=w399, index=0) -> (element=w377:dbl)
        n79 = Index Array(array=w386, index=w349) -> (element=w379:dbl)
        n80 = Index Array(array=w386, index=0) -> (element=w378:dbl)
        n81 = local write "Ig max"(w395) -> ()
        n82 = local write "Ig min"(w394) -> ()
        n83 = local write "Is max"(w390) -> ()
        n84 = local write "Is min"(w391) -> ()
        n85 = local write "Id max"(w433) -> ()
        n86 = local write "Id min"(w396) -> ()
        n87 = local write "I vs Vg"(w426) -> ()
        n88 = Build Array (concatenate)(w389, w390) -> (w368:dbl[])
        n89 = Build Array (concatenate)(w388, w391) -> (w366:dbl[])
        n90 = local write "Is off"(w375) -> ()
        n91 = local write "Is on"(w374) -> ()
        n92 = Build Array (concatenate)(w434, w433) -> (w365:dbl[])
        n93 = Build Array (concatenate)(w421, w396) -> (w364:dbl[])
        n94 = Build Array (concatenate)(w393, w395) -> (w363:dbl[])
        n95 = Build Array (concatenate)(w392, w394) -> (w362:dbl[])
        n96 = Build Array (concatenate)(w381, w374) -> (w361:dbl[])
        n97 = Build Array (concatenate)(w380, w375) -> (w360:dbl[])
        n98 = Build Array (concatenate)(w403, w376) -> (w359:dbl[])
        n99 = Build Array (concatenate)(w404, w377) -> (w358:dbl[])
        n100 = Build Array (concatenate)(w385, w379) -> (w357:dbl[])
        n101 = Build Array (concatenate)(w384, w378) -> (w356:dbl[])
        n102 = local write "Ig off"(w378) -> ()
        n103 = local write "Ig on"(w379) -> ()
        n104 = local write "Id off"(w377) -> ()
        n105 = local write "Id on"(w376) -> ()
        n106 = call "4155C Split array.vi"("Number of VAR2 steps"=w367, "Y2 data in"=w359, "X data in"=w373, "Y1 data in"=w361, "Y3 data in"=w357, "error in (no error)"=w355) -> ("Array of clusters"=w371:cluster{"Y data in":dbl[], "X data in":dbl[]}[], "error out"=w354:errorcluster)  [unwired: 1 in]
        n107 = call "4155C Split array.vi"("Number of VAR2 steps"=w367, "Y2 data in"=w358, "X data in"=w373, "Y1 data in"=w360, "Y3 data in"=w356, "error in (no error)"=w354) -> ("Array of clusters"=w372:cluster{"Y data in":dbl[], "X data in":dbl[]}[], "error out"=w353:errorcluster)  [unwired: 1 in]
        n108 = call "4155C Split array.vi"("Number of VAR2 steps"=w367, "Y2 data in"=w365, "X data in"=w373, "Y1 data in"=w368, "Y3 data in"=w363, "error in (no error)"=w353) -> ("Array of clusters"=w425:cluster{"Y data in":dbl[], "X data in":dbl[]}[], "error out"=w352:errorcluster)  [unwired: 1 in]
        n109 = call "4155C Split array.vi"("Number of VAR2 steps"=w367, "Y2 data in"=w364, "X data in"=w373, "Y1 data in"=w366, "Y3 data in"=w362, "error in (no error)"=w352) -> ("Array of clusters"=w422:cluster{"Y data in":dbl[], "X data in":dbl[]}[], "error out"=w351:errorcluster)  [unwired: 1 in]
        n110 = Open/Create/Replace File(file path (use dialog)=w482, error in=w351, operation (0:open)=w436) -> (refnum out=w419:refnum<file>, error out=w417:errorcluster)  [unwired: 3 in, 1 out]
        n111 = call "4155C Make Big 2d array.vi"("1D Var1"=w435, "1d IS"=w398, "1d ID"=w400, "1d IG"=w397, "1d SMU4"=w440, "SMU4"=w439, "VAR2 START"=w441, "Number of VAR2 steps"=w367, "VAR2 STEP"=w442, "VAR1 Name"="Vg", "Decimal places in header"=i8 1, "VAR2 Name"="Vd") -> ("Header array"=w420:string[], "Data array"=w418:dbl[][])  [unwired: 14 in]
        n112 = local write "Imax vs time"(w425) -> ()
        n113 = local write "Imin vs time"(w422) -> ()
        n114 = local write "Ion vs time"(w371) -> ()
        n115 = local write "Ioff vs time"(w372) -> ()
        n116 = call "4155C Config Chart Colours.vi"("Numeric"=w367, "XY Graph 2"=w402) -> ()  [unwired: 6 in]
        n117 = call "4155C Config Chart Colours.vi"("Numeric"=w367, "XY Graph 2"=w401) -> ()  [unwired: 6 in]
        n118 = call "4155C Config Chart Colours.vi"("Numeric"=w367, "XY Graph 2"=w370) -> ()  [unwired: 6 in]
        n119 = call "4155C Config Chart Colours.vi"("Numeric"=w367, "XY Graph 2"=w369) -> ()  [unwired: 6 in]
        n120 = call "4155C Config Chart Colours.vi"("Numeric"=w367, "XY Graph 2"=w432) -> ()  [unwired: 6 in]
        n121 = call "4155C Write array to file.vi"("Byte Stream File Refnum"=w419, "Header"=w420, "Data Array"=w418, "error in (no error)"=w417) -> ("dup refnum"=w416:refnum<file>, "error out"=w415:errorcluster)  [unwired: 1 in]
        n122 = Close File(refnum=w416, error in=w415) -> (error out=w477:errorcluster)  [unwired: 1 out]
      }
      frame "pulsedstressV" {
        w519 = 0
        n123 = Number To Decimal String(number=w510) -> (decimal integer string=w566:string)  [unwired: 1 in]
        n124 = Delete From Array(array=w500, index=0 ("Index")) -> (deleted portion=w557:string, array with subset deleted=w556:string[])  [unwired: 1 in]
        n125 = Bundle By Name(cluster=w536, "Emergency Stop"=w569) -> (w538:T2)
        n126 = VISA Write(VISA resource name=w550, write buffer=":PAGE:CHAN:MODE SWE;" ("write buffer (\"\")"), error in (no error)=w549) -> (VISA resource name out=w547:refnum<visa-resource-name>, error out=w548:errorcluster)  [unwired: 1 out]
        n127 = Concatenate Strings(w565, "-pulsedstressV-" ("Substring"), w566, w509, ".txt" ("Substring")) -> (w568:string)
        n128 = case shown="\"d\", Default" w557 {
          tunnel: [w578 w579] -> w555
          frame "s" {
            w578 = u16 0 items=["Single", "Double"] ("sweep mode")
          }
          frame "d", Default {
            w579 = u16 1 items=["Single", "Double"] ("sweep mode")
          }
        }
        n129 = Fract/Exp String To Number(string=w556) -> (number=w551:dbl[])  [unwired: 3 in, 1 out]
        n130 = String To Path(string=w568) -> (path=w564:path)
        n131 = Index Array(array=w551, index #1=0 ("Index")) -> (element #1=w528:dbl, element #2=w527:dbl, element #3=w524:dbl, element #4=w523:dbl, element #5=w522:dbl, element #6=w526:dbl)  [unwired: 5 in]
        n132 = Bundle By Name(cluster=w525, "Pulse period"=w523, "Base voltage"=w524, "Pulse width"=w522) -> (w521:T5)
        n133 = Unbundle By Name(w521) -> ("Pulse period"=w529:dbl)
        n134 = Bundle By Name(cluster=w553, "Gate Start"=w527, "Gate Stop"=w528, "Gate Step (linear only)"=0, "Gate Compliance"=w562, "Range mode"=w543, "Range"=w542) -> (w544:T6)
        n135 = call <vilib>:"compatOverwrite.vi"("overwrite (F)"=TRUE) -> ("overwrite?"=w514:T8)
        n136 = Bundle By Name(cluster=w552, "Drain Start"=w526, "Drain Stop"=w519, "Drain Step"=w519, "Drain Compliance"=w563, "Range mode"=w541, "Range"=w540) -> (w545:T7)
        n137 = call "4155C PulsedStressV.vi"("VISA resource name in"=w547, "sweep mode"=w555, "Panel Controls"=w538, "Gate"=w544, "Drain"=w545, "Timings"=w521, "error in (no error)"=w548, "SMU4"=w537) -> ("VISA Resource Name out"=w560:refnum<visa-resource-name>, "ID"=w517:dbl[], "IG"=w515:dbl[], "Outparams"=w539:T9, "error out"=w561:errorcluster)  [unwired: 3 in]
        n138 = Unbundle By Name(w539) -> ("Number of points"=w516:i32)  [unwired: 2 out]
        n139 = for {
          N: w516 -> [_]
          tunnel: [w575] -> w518 mode=indexing
          tunnel: w529 -> [w577]
          i -> [w576]
          n140 = Multiply(x=w577, y=w576) -> (x*y=w575:dbl)
        }
        n141 = Insert Into Array(array=dbl[][] [] ("Input Array"), new element=w518) -> (w530:dbl[][])  [unwired: 2 in]
        n142 = Insert Into Array(array=w530, new element=w517) -> (w535:dbl[][])  [unwired: 2 in]
        n143 = Insert Into Array(array=w535, new element=w515) -> (w534:dbl[][])  [unwired: 2 in]
        n144 = Transpose 2D Array(2D array=w534) -> (transposed array=w533:dbl[][])
        n145 = Open/Create/Replace File(file path (use dialog)=w564, error in=w561, operation (0:open)=w514) -> (refnum out=w572:refnum<file>, error out=w573:errorcluster)  [unwired: 3 in, 1 out]
        n146 = call "4155C Write array to file.vi"("Byte Stream File Refnum"=w572, "Header"=string[] ["Time /s", "Id /A", "Ig /A"], "Data Array"=w533, "error in (no error)"=w573) -> ("dup refnum"=w570:refnum<file>, "error out"=w571:errorcluster)  [unwired: 1 in]
        n147 = Close File(refnum=w570, error in=w571) -> (error out=w559:errorcluster)  [unwired: 1 out]
      }
      frame "transfer-fpp" {
        n148 = Number To Decimal String(number=w601) -> (decimal integer string=w655:string)  [unwired: 1 in]
        n149 = Bundle By Name(cluster=w631, "Emergency Stop"=w659) -> (w667:T1)
        n150 = Delete From Array(array=w646, index=0 ("Index")) -> (deleted portion=w644:string, array with subset deleted=w643:string[])  [unwired: 1 in]
        n151 = Concatenate Strings(w654, "-transferfpp-" ("Substring"), w655, w599, ".txt" ("Substring")) -> (w657:string)
        n152 = VISA Write(VISA resource name=w623, write buffer=":PAGE:CHAN:MODE SWE;" ("write buffer (\"\")"), error in (no error)=w622) -> (VISA resource name out=w620:refnum<visa-resource-name>, error out=w621:errorcluster)  [unwired: 1 out]
        n153 = case shown="\"d\", Default" w644 {
          tunnel: [w668 w669] -> w642
          frame "s" {
            w668 = u16 0 items=["Single", "Double"] ("sweep mode")
          }
          frame "d", Default {
            w669 = u16 1 items=["Single", "Double"] ("sweep mode")
          }
        }
        n154 = Fract/Exp String To Number(string=w643) -> (number=w627:dbl[])  [unwired: 3 in, 1 out]
        n155 = String To Path(string=w657) -> (path=w653:path)
        n156 = Index Array(array=w627, index #1=0 ("Index")) -> (element #1=w641:dbl, element #2=w640:dbl, element #3=w639:dbl)  [unwired: 2 in]
        n157 = Delete From Array(array=w627, length=3 ("Length"), index=0 ("Index")) -> (array with subset deleted=w625:dbl[])  [unwired: 1 out]
        n158 = Bundle By Name(cluster=w633, "Gate Start"=w641, "Gate Stop"=w640, "Gate Step (linear only)"=w639, "Gate Compliance"=w651, "Range mode"=w616, "Range"=w615) -> (w617:T6)
        n159 = Index Array(array=w625, index #1=0 ("Index")) -> (element #1=w636:dbl, element #2=w635:dbl, element #3=w634:dbl)  [unwired: 2 in]
        n160 = call <vilib>:"compatOverwrite.vi"("overwrite (F)"=TRUE) -> ("overwrite?"=w604:T8)
        n161 = Bundle By Name(cluster=w632, "Drain Start"=w636, "Drain Stop"=w635, "Drain Step"=w634, "Drain Compliance"=w652, "Range mode"=w614, "Range"=w613) -> (w618:T7)
        n162 = call "4155C Transfer-FPP.vi"("VISA resource name in"=w620, "Gate"=w617, "Drain"=w618, "Timings"=w650, "error in (no error)"=w621, "sweep mode"=w642, "Panel Controls"=w667) -> ("VG"=w658:dbl[], "Outparams"=w612:T9, "VISA Resource Name out"=w648:refnum<visa-resource-name>, "Vprobe2"=w608:dbl[], "ID"=w607:dbl[], "IG"=w606:dbl[], "Vprobe1"=w605:dbl[], "error out"=w649:errorcluster)  [unwired: 13 in]
        n163 = Unbundle By Name(w612) -> ("V2 Step"=w611:dbl, "V2 Start"=w610:dbl, "Number of points"=w609:i32)
        n164 = Open/Create/Replace File(file path (use dialog)=w653, error in=w649, operation (0:open)=w604) -> (refnum out=w664:refnum<file>, error out=w665:errorcluster)  [unwired: 3 in, 1 out]
        n165 = call "4155C Make Big 2d array FPP.vi"("1D Var1"=w658, "1d ID"=w607, "1d Vp2"=w608, "1d IG"=w606, "1d Vp1"=w605, "VAR2 START"=w610, "Number of VAR2 steps"=w609, "VAR2 STEP"=w611, "VAR1 Name"="Vg", "Decimal places in header"=i8 1, "VAR2 Name"="Vd") -> ("Header array"=w660:string[], "Data array"=w661:dbl[][])  [unwired: 15 in]
        n166 = call "4155C Write array to file.vi"("Byte Stream File Refnum"=w664, "Header"=w660, "Data Array"=w661, "error in (no error)"=w665) -> ("dup refnum"=w662:refnum<file>, "error out"=w663:errorcluster)  [unwired: 1 in]
        n167 = Close File(refnum=w662, error in=w663) -> (error out=w647:errorcluster)  [unwired: 1 out]
      }
      frame "output" {
        n168 = Number To Decimal String(number=w699) -> (decimal integer string=w748:string)  [unwired: 1 in]
        n169 = Bundle By Name(cluster=w725, "Emergency Stop"=w750) -> (w760:T1)
        n170 = Delete From Array(array=w740, index=0 ("Index")) -> (deleted portion=w738:string, array with subset deleted=w737:string[])  [unwired: 1 in]
        n171 = Concatenate Strings(w747, w670, w748, w698, "_O.txt" ("Suffix (output)")) -> (w749:string)
        n172 = VISA Write(VISA resource name=w716, write buffer=":PAGE:CHAN:MODE SWE;" ("write buffer (\"\")"), error in (no error)=w713) -> (VISA resource name out=w715:refnum<visa-resource-name>, error out=w714:errorcluster)  [unwired: 1 out]
        n173 = case shown="\"d\", Default" w738 {
          tunnel: [w761 w762] -> w736
          frame "s" {
            w761 = u16 0 items=["Single", "Double"] ("sweep mode")
          }
          frame "d", Default {
            w762 = u16 1 items=["Single", "Double"] ("sweep mode")
          }
        }
        n174 = Fract/Exp String To Number(string=w737) -> (number=w719:dbl[])  [unwired: 3 in, 1 out]
        n175 = String To Path(string=w749) -> (path=w746:path)
        n176 = Index Array(array=w719, index #1=0 ("Index")) -> (element #1=w735:dbl, element #2=w734:dbl, element #3=w733:dbl)  [unwired: 2 in]
        n177 = Delete From Array(array=w719, length=3 ("Length"), index=0 ("Index")) -> (array with subset deleted=w718:dbl[])  [unwired: 1 out]
        n178 = control-ref of="I vs Vd"() -> (w689:refnum<vi>)
        n179 = Bundle By Name(cluster=w727, "Gate Start"=w735, "Gate Stop"=w734, "Gate Step (linear only)"=w733, "Gate Compliance"=w744, "Range mode"=w711, "Range"=w710) -> (w759:T6)
        n180 = Index Array(array=w718, index #1=0 ("Index")) -> (element #1=w730:dbl, element #2=w729:dbl, element #3=w728:dbl)  [unwired: 2 in]
        n181 = call <vilib>:"compatOverwrite.vi"("overwrite (F)"=TRUE) -> ("overwrite?"=w703:T8)
        n182 = Bundle By Name(cluster=w726, "Drain Start"=w730, "Drain Stop"=w729, "Drain Step"=w728, "Drain Compliance"=w745, "Range mode"=w709, "Range"=w712) -> (w758:T7)
        n183 = call "4155C Output.vi"("VISA resource name in"=w715, "Gate"=w759, "Drain"=w758, "Timings"=w743, "error in (no error)"=w714, "SMU4"=w705, "sweep mode"=w736, "Panel controls"=w760) -> ("VD"=w696:dbl[], "Outparams"=w707:T9, "VISA Resource Name out"=w742:refnum<visa-resource-name>, "IS"=w695:dbl[], "ID"=w694:dbl[], "IG"=w693:dbl[], "error out"=w691:errorcluster, "SMU4"=w704:dbl[])  [unwired: 12 in]
        n184 = Unbundle By Name(w707) -> ("V2 Step"=w708:dbl, "V2 Start"=w706:dbl, "Number of points"=w688:i32)
        n185 = call "4155C Split array.vi"("Number of VAR2 steps"=w688, "Y2 data in"=w694, "X data in"=w696, "Y1 data in"=w695, "Y3 data in"=w693, "error in (no error)"=w691) -> ("Array of clusters"=w692:cluster{"Y data in":dbl[], "X data in":dbl[]}[], "error out"=w690:errorcluster)  [unwired: 1 in]
        n186 = local write "I vs Vd"(w692) -> ()
        n187 = call "4155C Config Chart Colours.vi"("Numeric"=w688, "XY Graph 2"=w689) -> ()  [unwired: 6 in]
        n188 = Open/Create/Replace File(file path (use dialog)=w746, error in=w690, operation (0:open)=w703) -> (refnum out=w755:refnum<file>, error out=w756:errorcluster)  [unwired: 3 in, 1 out]
        n189 = call "4155C Make Big 2d array.vi"("1D Var1"=w696, "1d IS"=w695, "1d ID"=w694, "1d IG"=w693, "1d SMU4"=w704, "SMU4"=w705, "VAR2 START"=w706, "Number of VAR2 steps"=w688, "VAR2 STEP"=w708, "VAR1 Name"="Vd", "Decimal places in header"=i8 1, "VAR2 Name"="Vg") -> ("Header array"=w751:string[], "Data array"=w752:dbl[][])  [unwired: 14 in]
        n190 = call "4155C Write array to file.vi"("Byte Stream File Refnum"=w755, "Header"=w751, "Data Array"=w752, "error in (no error)"=w756) -> ("dup refnum"=w753:refnum<file>, "error out"=w754:errorcluster)  [unwired: 1 in]
        n191 = Close File(refnum=w753, error in=w754) -> (error out=w741:errorcluster)  [unwired: 1 out]
      }
      frame "output2" {
        # "Adjusts graph colors."
        # "Adjusts graph colors."
        # "Is off"
        # "Is on"
        # "Ion will be the middle element of the array. The calculation of the index is done only once, since Is, Id, and Ig have the same dimensions."
        # "Ig off"
        # "Ig on"
        # "Is min"
        # "Is max"
        # "Ig min"
        # "Ig max"
        # "abs(Ig)"
        # "abs(Is)"
        # "Id min"
        # "Id max"
        # "Y1: Is\nY2: Id\nY3: Ig"
        # "abs(Id)"
        # "Adjusts graph colors."
        # "Adjusts graph colors."
        # "Id off"
        # "Id on"
        # "Adjusts graph colors."
        # "Time array"
        n192 = Delete From Array(array=w892, index=0 ("Index")) -> (deleted portion=w890:string, array with subset deleted=w889:string[])  [unwired: 1 in]
        n193 = Bundle By Name(cluster=w763, "Emergency Stop"=w901) -> (w854:T1)
        n194 = Number To Decimal String(number=w848) -> (decimal integer string=w847:string)  [unwired: 1 in]
        n195 = case shown="\"d\", Default" w890 {
          tunnel: [w903 w904] -> w888
          frame "s" {
            w903 = u16 0 items=["Single", "Double"] ("sweep mode")
          }
          frame "d", Default {
            w904 = u16 1 items=["Single", "Double"] ("sweep mode")
          }
        }
        n196 = Fract/Exp String To Number(string=w889) -> (number=w874:dbl[])  [unwired: 3 in, 1 out]
        n197 = Concatenate Strings(w899, w764, w847, w845, "_O_1_C_L.txt" ("Suffix (transfer)")) -> (w900:string)
        n198 = VISA Write(VISA resource name=w870, write buffer=":PAGE:CHAN:MODE SWE;" ("write buffer (\"\")"), error in (no error)=w869) -> (VISA resource name out=w867:refnum<visa-resource-name>, error out=w868:errorcluster)  [unwired: 1 out]
        n199 = String To Path(string=w900) -> (path=w898:path)
        n200 = Index Array(array=w874, index #1=0 ("Index")) -> (element #1=w887:dbl, element #2=w886:dbl, element #3=w885:dbl)  [unwired: 2 in]
        n201 = Delete From Array(array=w874, length=3 ("Length"), index=0 ("Index")) -> (array with subset deleted=w872:dbl[])  [unwired: 1 out]
        n202 = Build Array (concatenate)(w844, w840) -> (w790:i32[])
        n203 = Bundle By Name(cluster=w879, "Gate Start"=w887, "Gate Stop"=w886, "Gate Step (linear only)"=w885, "Gate Compliance"=w896, "Range mode"=w863, "Range"=w862) -> (w864:T6)
        n204 = control-ref of="Imax vs time"() -> (w819:refnum<vi>)
        n205 = control-ref of="Imin vs time"() -> (w818:refnum<vi>)
        n206 = control-ref of="Ion vs time"() -> (w787:refnum<vi>)
        n207 = control-ref of="Ioff vs time"() -> (w786:refnum<vi>)
        n208 = control-ref of="I vs Vg"() -> (w849:refnum<vi>)
        n209 = Index Array(array=w872, index #1=0 ("Index")) -> (element #1=w882:dbl, element #2=w881:dbl, element #3=w880:dbl)  [unwired: 2 in]
        n210 = call <vilib>:"compatOverwrite.vi"("overwrite (F)"=TRUE) -> ("overwrite?"=w853:T8)
        n211 = Bundle By Name(cluster=w878, "Drain Start"=w882, "Drain Stop"=w881, "Drain Step"=w880, "Drain Compliance"=w897, "Range mode"=w861, "Range"=w860) -> (w865:T7)
        n212 = call "4155C Output.vi"("VISA resource name in"=w867, "Gate"=w864, "Drain"=w865, "Timings"=w895, "error in (no error)"=w868, "SMU4"=w855, "sweep mode"=w888, "Panel controls"=w854) -> ("VD"=w852:dbl[], "Outparams"=w859:T9, "VISA Resource Name out"=w894:refnum<visa-resource-name>, "IS"=w815:dbl[], "ID"=w817:dbl[], "IG"=w814:dbl[], "error out"=w841:errorcluster, "SMU4"=w856:dbl[])  [unwired: 12 in]
        n213 = Unbundle By Name(w859) -> ("V2 Step"=w858:dbl, "V2 Start"=w857:dbl, "Number of points"=w784:i32)
        n214 = Absolute Value(x=w815) -> (abs(x)=w800:dbl[])
        n215 = Absolute Value(x=w817) -> (abs(x)=w816:dbl[])
        n216 = Absolute Value(x=w814) -> (abs(x)=w803:dbl[])
        n217 = Array Size(array=w816) -> (size(s)=w824:i32)
        n218 = Divide(x=w824, y=2) -> (x/y=w767:dbl)
        n219 = Subtract(x=w767, y=1) -> (x-y=w766:dbl)
        n220 = Array Max & Min(array=w800) -> (max value=w807:dbl, min value=w808:dbl)  [unwired: 2 out]
        n221 = Array Max & Min(array=w816) -> (max value=w850:dbl, min value=w813:dbl)  [unwired: 2 out]
        n222 = Array Max & Min(array=w803) -> (max value=w812:dbl, min value=w811:dbl)  [unwired: 2 out]
        n223 = call "4155C Split array.vi"("Number of VAR2 steps"=w784, "Y2 data in"=w817, "X data in"=w852, "Y1 data in"=w815, "Y3 data in"=w814, "error in (no error)"=w841) -> ("Array of clusters"=w843:cluster{"Y data in":dbl[], "X data in":dbl[]}[], "error out"=w772:errorcluster)  [unwired: 1 in]
        n224 = Index Array(array=w800, index=w766) -> (element=w791:dbl)
        n225 = Index Array(array=w800, index=0) -> (element=w792:dbl)
        n226 = Index Array(array=w816, index=w766) -> (element=w793:dbl)
        n227 = Index Array(array=w816, index=0) -> (element=w794:dbl)
        n228 = Index Array(array=w803, index=w766) -> (element=w796:dbl)
        n229 = Index Array(array=w803, index=0) -> (element=w795:dbl)
        n230 = local write "Ig max"(w812) -> ()
        n231 = local write "Ig min"(w811) -> ()
        n232 = local write "Is max"(w807) -> ()
        n233 = local write "Is min"(w808) -> ()
        n234 = local write "Id max"(w850) -> ()
        n235 = local write "Id min"(w813) -> ()
        n236 = local write "I vs Vd"(w843) -> ()
        n237 = Build Array (concatenate)(w806, w807) -> (w785:dbl[])
        n238 = Build Array (concatenate)(w805, w808) -> (w783:dbl[])
        n239 = local write "Is off"(w792) -> ()
        n240 = local write "Is on"(w791) -> ()
        n241 = Build Array (concatenate)(w851, w850) -> (w782:dbl[])
        n242 = Build Array (concatenate)(w838, w813) -> (w781:dbl[])
        n243 = Build Array (concatenate)(w810, w812) -> (w780:dbl[])
        n244 = Build Array (concatenate)(w809, w811) -> (w779:dbl[])
        n245 = Build Array (concatenate)(w798, w791) -> (w778:dbl[])
        n246 = Build Array (concatenate)(w797, w792) -> (w777:dbl[])
        n247 = Build Array (concatenate)(w820, w793) -> (w776:dbl[])
        n248 = Build Array (concatenate)(w821, w794) -> (w775:dbl[])
        n249 = Build Array (concatenate)(w802, w796) -> (w774:dbl[])
        n250 = Build Array (concatenate)(w801, w795) -> (w773:dbl[])
        n251 = local write "Ig off"(w795) -> ()
        n252 = local write "Ig on"(w796) -> ()
        n253 = local write "Id off"(w794) -> ()
        n254 = local write "Id on"(w793) -> ()
        n255 = call "4155C Split array.vi"("Number of VAR2 steps"=w784, "Y2 data in"=w776, "X data in"=w790, "Y1 data in"=w778, "Y3 data in"=w774, "error in (no error)"=w772) -> ("Array of clusters"=w788:cluster{"Y data in":dbl[], "X data in":dbl[]}[], "error out"=w771:errorcluster)  [unwired: 1 in]
        n256 = call "4155C Split array.vi"("Number of VAR2 steps"=w784, "Y2 data in"=w775, "X data in"=w790, "Y1 data in"=w777, "Y3 data in"=w773, "error in (no error)"=w771) -> ("Array of clusters"=w789:cluster{"Y data in":dbl[], "X data in":dbl[]}[], "error out"=w770:errorcluster)  [unwired: 1 in]
        n257 = call "4155C Split array.vi"("Number of VAR2 steps"=w784, "Y2 data in"=w782, "X data in"=w790, "Y1 data in"=w785, "Y3 data in"=w780, "error in (no error)"=w770) -> ("Array of clusters"=w842:cluster{"Y data in":dbl[], "X data in":dbl[]}[], "error out"=w769:errorcluster)  [unwired: 1 in]
        n258 = call "4155C Split array.vi"("Number of VAR2 steps"=w784, "Y2 data in"=w781, "X data in"=w790, "Y1 data in"=w783, "Y3 data in"=w779, "error in (no error)"=w769) -> ("Array of clusters"=w839:cluster{"Y data in":dbl[], "X data in":dbl[]}[], "error out"=w768:errorcluster)  [unwired: 1 in]
        n259 = Open/Create/Replace File(file path (use dialog)=w898, error in=w768, operation (0:open)=w853) -> (refnum out=w836:refnum<file>, error out=w834:errorcluster)  [unwired: 3 in, 1 out]
        n260 = call "4155C Make Big 2d array.vi"("1D Var1"=w852, "1d IS"=w815, "1d ID"=w817, "1d IG"=w814, "1d SMU4"=w856, "SMU4"=w855, "VAR2 START"=w857, "Number of VAR2 steps"=w784, "VAR2 STEP"=w858, "VAR1 Name"="Vd", "Decimal places in header"=i8 1, "VAR2 Name"="Vg") -> ("Header array"=w837:string[], "Data array"=w835:dbl[][])  [unwired: 14 in]
        n261 = local write "Imax vs time"(w842) -> ()
        n262 = local write "Imin vs time"(w839) -> ()
        n263 = local write "Ion vs time"(w788) -> ()
        n264 = local write "Ioff vs time"(w789) -> ()
        n265 = call "4155C Config Chart Colours.vi"("Numeric"=w784, "XY Graph 2"=w819) -> ()  [unwired: 6 in]
        n266 = call "4155C Config Chart Colours.vi"("Numeric"=w784, "XY Graph 2"=w818) -> ()  [unwired: 6 in]
        n267 = call "4155C Config Chart Colours.vi"("Numeric"=w784, "XY Graph 2"=w787) -> ()  [unwired: 6 in]
        n268 = call "4155C Config Chart Colours.vi"("Numeric"=w784, "XY Graph 2"=w786) -> ()  [unwired: 6 in]
        n269 = call "4155C Config Chart Colours.vi"("Numeric"=w784, "XY Graph 2"=w849) -> ()  [unwired: 6 in]
        n270 = call "4155C Write array to file.vi"("Byte Stream File Refnum"=w836, "Header"=w837, "Data Array"=w835, "error in (no error)"=w834) -> ("dup refnum"=w833:refnum<file>, "error out"=w832:errorcluster)  [unwired: 1 in]
        n271 = Close File(refnum=w833, error in=w832) -> (error out=w893:errorcluster)  [unwired: 1 out]
      }
      frame "output-fpp" {
        n272 = Number To Decimal String(number=w925) -> (decimal integer string=w979:string)  [unwired: 1 in]
        n273 = Bundle By Name(cluster=w955, "Emergency Stop"=w982) -> (w992:T1)
        n274 = Delete From Array(array=w970, index=0 ("Index")) -> (deleted portion=w968:string, array with subset deleted=w967:string[])  [unwired: 1 in]
        n275 = VISA Write(VISA resource name=w946, write buffer=":PAGE:CHAN:MODE SWE;" ("write buffer (\"\")"), error in (no error)=w943) -> (VISA resource name out=w945:refnum<visa-resource-name>, error out=w944:errorcluster)  [unwired: 1 out]
        n276 = Concatenate Strings(w978, "-outputfpp-" ("Substring"), w979, w924, ".txt" ("Substring")) -> (w981:string)
        n277 = case shown="\"d\", Default" w968 {
          tunnel: [w993 w994] -> w966
          frame "s" {
            w993 = u16 0 items=["Single", "Double"] ("sweep mode")
          }
          frame "d", Default {
            w994 = u16 1 items=["Single", "Double"] ("sweep mode")
          }
        }
        n278 = Fract/Exp String To Number(string=w967) -> (number=w949:dbl[])  [unwired: 3 in, 1 out]
        n279 = String To Path(string=w981) -> (path=w977:path)
        n280 = Index Array(array=w949, index #1=0 ("Index")) -> (element #1=w965:dbl, element #2=w964:dbl, element #3=w963:dbl)  [unwired: 2 in]
        n281 = Delete From Array(array=w949, length=3 ("Length"), index=0 ("Index")) -> (array with subset deleted=w948:dbl[])  [unwired: 1 out]
        n282 = Bundle By Name(cluster=w957, "Gate Start"=w965, "Gate Stop"=w964, "Gate Step (linear only)"=w963, "Gate Compliance"=w975, "Range mode"=w941, "Range"=w940) -> (w991:T6)
        n283 = Index Array(array=w948, index #1=0 ("Index")) -> (element #1=w960:dbl, element #2=w959:dbl, element #3=w958:dbl)  [unwired: 2 in]
        n284 = call <vilib>:"compatOverwrite.vi"("overwrite (F)"=TRUE) -> ("overwrite?"=w929:T8)
        n285 = Bundle By Name(cluster=w956, "Drain Start"=w960, "Drain Stop"=w959, "Drain Step"=w958, "Drain Compliance"=w976, "Range mode"=w939, "Range"=w942) -> (w990:T7)
        n286 = call "4155C Output-FPP.vi"("VISA resource name in"=w945, "Gate"=w991, "Drain"=w990, "Timings"=w974, "error in (no error)"=w944, "sweep mode"=w966, "Panel controls"=w992) -> ("VD"=w934:dbl[], "Outparams"=w937:T9, "VISA Resource Name out"=w972:refnum<visa-resource-name>, "Vprobe2"=w933:dbl[], "ID"=w932:dbl[], "IG"=w931:dbl[], "Vprobe1"=w930:dbl[], "error out"=w973:errorcluster)  [unwired: 13 in]
        n287 = Unbundle By Name(w937) -> ("V2 Step"=w938:dbl, "V2 Start"=w936:dbl, "Number of points"=w935:i32)
        n288 = Open/Create/Replace File(file path (use dialog)=w977, error in=w973, operation (0:open)=w929) -> (refnum out=w987:refnum<file>, error out=w988:errorcluster)  [unwired: 3 in, 1 out]
        n289 = call "4155C Make Big 2d array FPP.vi"("1D Var1"=w934, "1d ID"=w932, "1d Vp2"=w933, "1d IG"=w931, "1d Vp1"=w930, "VAR2 START"=w936, "Number of VAR2 steps"=w935, "VAR2 STEP"=w938, "VAR1 Name"="Vd", "Decimal places in header"=i8 1, "VAR2 Name"="Vg") -> ("Header array"=w983:string[], "Data array"=w984:dbl[][])  [unwired: 15 in]
        n290 = call "4155C Write array to file.vi"("Byte Stream File Refnum"=w987, "Header"=w983, "Data Array"=w984, "error in (no error)"=w988) -> ("dup refnum"=w985:refnum<file>, "error out"=w986:errorcluster)  [unwired: 1 in]
        n291 = Close File(refnum=w985, error in=w986) -> (error out=w971:errorcluster)  [unwired: 1 out]
      }
      frame "itime" {
        n292 = Delete From Array(array=w997, index=1) -> (deleted portion=w996:string)  [unwired: 1 in, 1 out]
        n293 = Delete From Array(array=w997, index=0 ("Index")) -> (deleted portion=w1031:string)  [unwired: 1 in, 1 out]
        n294 = Fract/Exp String To Number(string=w996) -> (number=w995:dbl)  [unwired: 3 in, 1 out]
        n295 = case shown="\"l\"" w1031 {
          tunnel: w1030 -> [w1036 w1038 w1042]
          tunnel: [w1035 w1037 w1041] -> w1023
          tunnel: w995 -> [w1033 _ w1040]
          frame "s" {
            w1034 = u32 0 items=["short  ", "medium  ", "long  "] ("integration time 2")
            n296 = Bundle By Name(cluster=w1036, "integration time"=w1034, "Short/Long integration time"=w1033) -> (w1035:T5)
          }
          frame "m", Default {
            w1039 = u32 1 items=["short  ", "medium  ", "long  "] ("integration time 2")
            n297 = Bundle By Name(cluster=w1038, "integration time"=w1039) -> (w1037:T5)
          }
          frame "l" {
            w1043 = u32 2 items=["short  ", "medium  ", "long  "] ("integration time 2")
            n298 = Bundle By Name(cluster=w1042, "integration time"=w1043, "Short/Long integration time"=w1040) -> (w1041:T5)
          }
        }
      }
      frame "pulsed" {
        n299 = Delete From Array(array=w1077, index=0 ("Index")) -> (deleted portion=w1078:string, array with subset deleted=w1065:string[])  [unwired: 1 in]
        n300 = case shown="\"on\", Default" w1078 {
          tunnel: w1076 -> [w1088 w1091]
          tunnel: [w1087 w1090] -> w1069
          tunnel: w1065 -> [w1085 _]
          frame "on", Default {
            w1086 = u16 1 items=["Continuous", "Pulsed"] ("sweep method")
            n301 = Fract/Exp String To Number(string=w1085) -> (number=w1083:dbl[])  [unwired: 3 in, 1 out]
            n302 = Index Array(array=w1083, index #1=0 ("Index")) -> (element #1=w1082:dbl, element #2=w1081:dbl, element #3=w1080:dbl)  [unwired: 2 in]
            n303 = Bundle By Name(cluster=w1088, "sweep method"=w1086, "Pulse period"=w1082, "Base voltage"=w1081, "Pulse width"=w1080) -> (w1087:T5)
          }
          frame "off" {
            w1089 = u16 0 items=["Continuous", "Pulsed"] ("sweep method")
            n304 = Bundle By Name(cluster=w1091, "sweep method"=w1089) -> (w1090:T5)
          }
        }
      }
      frame "gaterangemode" {
        n305 = Delete From Array(array=w1123, index=0 ("Index")) -> (deleted portion=w1124:string)  [unwired: 1 in, 1 out]
        n306 = case shown="\"f\"" w1124 {
          tunnel: [w1126 w1127 w1128] -> w1113
          frame "a", Default {
            w1126 = u16 0 items=["Auto", "Limited", "Fixed"] ("Gate Range\nmode 2")
          }
          frame "f" {
            w1127 = u16 2 items=["Auto", "Limited", "Fixed"] ("Gate Range\nmode 2")
          }
          frame "l" {
            w1128 = u16 1 items=["Auto", "Limited", "Fixed"] ("Gate Range\nmode 2")
          }
        }
      }
      frame "gaterange" {
        (unwired) u8 11 items=["10fA  ", "100fA  ", "1nA  ", "10nA", "100nA", "1uA", "10uA", "100uA", "1mA", "10mA", "100mA", "1A"] ("Gate Range 2")
        n307 = Delete From Array(array=w1167, index=0 ("Index")) -> (deleted portion=w1157:string)  [unwired: 1 in, 1 out]
        n308 = Scan Value(string=w1157, format string="") -> (value=w1155:dbl)  [unwired: 1 in, 1 out]
        n309 = Logarithm Base 10(1:w1155) -> (0:w1154:dbl)
        n310 = Round To Nearest(number=w1154) -> (nearest integer value=w1153:dbl)
        n311 = Add(x=w1153, y=11.0) -> (x+y=w1151:dbl)
        n312 = To Unsigned Byte Integer(number=w1151) -> (unsigned 8bit integer=w1150:u8)
      }
      frame "drainrange" {
        (unwired) u8 11 items=["10fA  ", "100fA  ", "1nA  ", "10nA", "100nA", "1uA", "10uA", "100uA", "1mA", "10mA", "100mA", "1A"] ("Gate Range 2")
        n313 = Delete From Array(array=w1207, index=0 ("Index")) -> (deleted portion=w1198:string)  [unwired: 1 in, 1 out]
        n314 = Scan Value(string=w1198, format string="") -> (value=w1196:dbl)  [unwired: 1 in, 1 out]
        n315 = Logarithm Base 10(1:w1196) -> (0:w1195:dbl)
        n316 = Round To Nearest(number=w1195) -> (nearest integer value=w1194:dbl)
        n317 = Add(x=w1194, y=11.0) -> (x+y=w1192:dbl)
        n318 = To Unsigned Byte Integer(number=w1192) -> (unsigned 8bit integer=w1191:u8)
      }
      frame "drainrangemode" {
        n319 = Delete From Array(array=w1240, index=0 ("Index")) -> (deleted portion=w1241:string)  [unwired: 1 in, 1 out]
        n320 = case shown="\"f\"" w1241 {
          tunnel: [w1243 w1244 w1245] -> w1230
          frame "a", Default {
            w1243 = u16 0 items=["Auto", "Limited", "Fixed"] ("Gate Range\nmode 2")
          }
          frame "f" {
            w1244 = u16 2 items=["Auto", "Limited", "Fixed"] ("Gate Range\nmode 2")
          }
          frame "l" {
            w1245 = u16 1 items=["Auto", "Limited", "Fixed"] ("Gate Range\nmode 2")
          }
        }
      }
      frame "Error", Default {
      }
      frame "logfile" {
        n321 = Number To Decimal String(number=w1298) -> (decimal integer string=w1333:string)  [unwired: 1 in]
        n322 = Concatenate Strings(w1332, "logfile" ("Substring"), w1333, w1296, ".txt" ("Substring")) -> (w1330:string)
        n323 = String To Path(string=w1330) -> (path=w1303:path)
        n324 = Unbundle(w1329) -> ("integration time"=w1328:u32, "Short/Long integration time"=w1327:dbl, "hold time (sec)"=w1326:dbl, "delay time (sec)"=w1325:dbl, "Step Time (0 disables)"=w1324:dbl, "sweep method"=w1323:u16, "Pulse period"=w1322:dbl, "Base voltage"=w1321:dbl, "Pulse width"=w1320:dbl)
        n325 = Build Array(w1328, w1327, w1326, w1325, w1324, w1323, w1322, w1321, w1320, w1314, w1315, w1316, w1317, w1318, w1319) -> (w1307:dbl[])
        n326 = Insert Into Array(array=dbl[][] [] ("Input Array"), new element=w1307) -> (w1306:dbl[][])  [unwired: 2 in]
        n327 = call <vilib>:"compatOverwrite.vi"("overwrite (F)"=TRUE) -> ("overwrite?"=w1301:T8)
        n328 = Open/Create/Replace File(file path (use dialog)=w1303, error in=w1305, operation (0:open)=w1301) -> (refnum out=w1311:refnum<file>, error out=w1310:errorcluster)  [unwired: 3 in, 1 out]
        n329 = call "4155C Write array to file.vi"("Byte Stream File Refnum"=w1311, "Header"=string[] ["Int Time", "Short/Long Itime", "Hold time", "Delay time", "Step time", "Sweep method", "Pulse period", "Base Voltage", "Pulse width", "Drain compliance", "Gate compliance", "Gate range mode", "Gate range", "S/D range mode", "S/D range"], "Data Array"=w1306, "error in (no error)"=w1310) -> ("dup refnum"=w1313:refnum<file>, "error out"=w1312:errorcluster)  [unwired: 1 in]
        n330 = Close File(refnum=w1313, error in=w1312) -> (error out=w1304:errorcluster)  [unwired: 1 out]
      }
      frame "sample" {
        n331 = Number To Decimal String(number=w1356) -> (decimal integer string=w1404:string)  [unwired: 1 in]
        n332 = Fract/Exp String To Number(string=w1401) -> (number=w1362:dbl[])  [unwired: 3 in, 1 out]
        n333 = Concatenate Strings(w1379, "-sample-" ("Substring"), w1404, w1354, ".txt" ("Substring")) -> (w1402:string)
        n334 = Index Array(array=w1362, index=0 ("Index")) -> (element=w1399:dbl)
        n335 = String To Path(string=w1402) -> (path=w1383:path)
        n336 = Index Array(array=w1362, index=2 ("Index")) -> (element=w1395:dbl)
        n337 = Index Array(array=w1362, index=3 ("Index")) -> (element=w1364:dbl)
        n338 = Index Array(array=w1362, index=4 ("Index")) -> (element=w1361:dbl)
        n339 = call "4155C Config Sampling Measurements.vi"("Sampling interval"=w1361, "Sample time"=w1364, "Display on/off"=TRUE, "Timings"=w1370, "Num Points"=w1395, "error in (no error)"=w1406, "Drain Compliance"=w1405, "Gate Compliance"=w1380, "VISA session"=w1407) -> ("error out"=w1408:errorcluster, "dup VISA resource name"=w1409:refnum<visa-resource-name>)  [unwired: 1 in]
        n340 = Index Array(array=w1362, index=1 ("Index")) -> (element=w1396:dbl)
        n341 = call "4155C Take Sample.vi"("Emergency Stop"=w1376, "error in (no error)"=w1408, "Vd"=w1396, "Vg"=w1399, "VISA resource name in"=w1409) -> ("error out"=w1374:errorcluster, "Id"=w1411:dbl[], "Ig"=w1385:dbl[], "VISA Resource Name out"=w1372:refnum<visa-resource-name>, "Is"=w1410:dbl[], "Time"=w1389:dbl[])  [unwired: 1 in]
        n342 = Insert Into Array(array=dbl[][] [] ("Input Array"), new element=w1389) -> (w1388:dbl[][])  [unwired: 2 in]
        n343 = Insert Into Array(array=w1388, new element=w1385) -> (w1387:dbl[][])  [unwired: 2 in]
        n344 = Insert Into Array(array=w1387, new element=w1411) -> (w1386:dbl[][])  [unwired: 2 in]
        n345 = VISA Write(VISA resource name=w1372, write buffer=":DISP ON" ("write buffer (\"\")"), error in (no error)=w1374) -> (VISA resource name out=w1371:refnum<visa-resource-name>, error out=w1373:errorcluster)  [unwired: 1 out]
        n346 = Insert Into Array(array=w1386, new element=w1410) -> (w1378:dbl[][])  [unwired: 2 in]
        n347 = Transpose 2D Array(2D array=w1378) -> (transposed array=w1377:dbl[][])
        n348 = call <vilib>:"compatOverwrite.vi"("overwrite (F)"=TRUE) -> ("overwrite?"=w1359:T8)
        n349 = Open/Create/Replace File(file path (use dialog)=w1383, error in=w1373, operation (0:open)=w1359) -> (refnum out=w1392:refnum<file>, error out=w1391:errorcluster)  [unwired: 3 in, 1 out]
        n350 = call "4155C Write array to file.vi"("Byte Stream File Refnum"=w1392, "Header"=string[] ["Time /s", "Ig /A", "Id /A", "Is /A"], "Data Array"=w1377, "error in (no error)"=w1391) -> ("dup refnum"=w1394:refnum<file>, "error out"=w1393:errorcluster)  [unwired: 1 in]
        n351 = Close File(refnum=w1394, error in=w1393) -> (error out=w1381:errorcluster)  [unwired: 1 out]
      }
      frame "samplei" {
        n352 = Number To Decimal String(number=w1433) -> (decimal integer string=w1484:string)  [unwired: 1 in]
        n353 = Concatenate Strings(w1463, "-samplei-" ("Substring"), w1484, w1432, ".txt" ("Substring")) -> (w1482:string)
        n354 = Fract/Exp String To Number(string=w1481) -> (number=w1448:dbl[])  [unwired: 3 in, 1 out]
        n355 = String To Path(string=w1482) -> (path=w1466:path)
        n356 = Index Array(array=w1448, index=4 ("Index")) -> (element=w1442:dbl)
        n357 = Index Array(array=w1448, index=3 ("Index")) -> (element=w1443:dbl)
        n358 = Index Array(array=w1448, index=1 ("Index")) -> (element=w1445:dbl)
        n359 = Index Array(array=w1448, index=0 ("Index")) -> (element=w1446:dbl)
        n360 = Index Array(array=w1448, index=2 ("Index")) -> (element=w1444:dbl)
        n361 = call "4155C Config SamplingI Measurements.vi"("Sample time"=w1444, "Display on/off"=TRUE, "Timings"=w1455, "Num Points"=w1445, "error in (no error)"=w1486, "Sampling interval"=w1443, "VISA session"=w1487) -> ("error out"=w1488:errorcluster, "dup VISA resource name"=w1489:refnum<visa-resource-name>)  [unwired: 3 in]
        n362 = call "4155C Take SampleI.vi"("Emergency Stop"=w1460, "error in (no error)"=w1488, "Idg 2"=w1446, "Vdg compliance 2"=w1442, "VISA resource name in"=w1489) -> ("error out"=w1458:errorcluster, "Idg"=w1491:dbl[], "Vdg"=w1468:dbl[], "VISA Resource Name out"=w1456:refnum<visa-resource-name>, "Is"=w1490:dbl[], "Time"=w1472:dbl[])  [unwired: 1 in]
        n363 = Insert Into Array(array=dbl[][] [] ("Input Array"), new element=w1472) -> (w1471:dbl[][])  [unwired: 2 in]
        n364 = Insert Into Array(array=w1471, new element=w1468) -> (w1470:dbl[][])  [unwired: 2 in]
        n365 = Insert Into Array(array=w1470, new element=w1491) -> (w1469:dbl[][])  [unwired: 2 in]
        n366 = VISA Write(VISA resource name=w1456, write buffer=":DISP ON" ("write buffer (\"\")"), error in (no error)=w1458) -> (VISA resource name out=w1441:refnum<visa-resource-name>, error out=w1457:errorcluster)  [unwired: 1 out]
        n367 = Insert Into Array(array=w1469, new element=w1490) -> (w1462:dbl[][])  [unwired: 2 in]
        n368 = call <vilib>:"compatOverwrite.vi"("overwrite (F)"=TRUE) -> ("overwrite?"=w1436:T8)
        n369 = Open/Create/Replace File(file path (use dialog)=w1466, error in=w1457, operation (0:open)=w1436) -> (refnum out=w1475:refnum<file>, error out=w1474:errorcluster)  [unwired: 3 in, 1 out]
        n370 = Transpose 2D Array(2D array=w1462) -> (transposed array=w1461:dbl[][])
        n371 = call "4155C Write array to file.vi"("Byte Stream File Refnum"=w1475, "Header"=string[] ["Time /s", "Vdg /V", "Idg /A", "Is /A"], "Data Array"=w1461, "error in (no error)"=w1474) -> ("dup refnum"=w1477:refnum<file>, "error out"=w1476:errorcluster)  [unwired: 1 in]
        n372 = Close File(refnum=w1477, error in=w1476) -> (error out=w1439:errorcluster)  [unwired: 1 out]
        n373 = VISA Write(VISA resource name=w1441, write buffer=";:PAGE:SCON:STAN OFF;:PAGE:CHAN:VSU2:DIS;" ("write buffer (\"\")"), error in (no error)=w1439) -> (VISA resource name out=w1437:refnum<visa-resource-name>, error out=w1438:errorcluster)  [unwired: 1 out]
      }
      frame "#" {
        n374 = VISA Write(VISA resource name=w1517, write buffer=":DISP ON" ("write buffer (\"\")"), error in (no error)=w1516) -> (VISA resource name out=w1515:refnum<visa-resource-name>, error out=w1514:errorcluster)  [unwired: 1 out]
      }
      frame "stressV" {
        n375 = Number To Decimal String(number=w1546) -> (decimal integer string=w1587:string)  [unwired: 1 in]
        n376 = Concatenate Strings(w1571, "-stressV-" ("Substring"), w1587, w1545, ".txt" ("Substring")) -> (w1585:string)
        n377 = Fract/Exp String To Number(string=w1584) -> (number=w1557:dbl[])  [unwired: 3 in, 1 out]
        n378 = String To Path(string=w1585) -> (path=w1575:path)
        n379 = Index Array(array=w1557, index=3 ("Index")) -> (element=w1554:dbl)
        n380 = Index Array(array=w1557, index=1 ("Index")) -> (element=w1552:dbl)
        n381 = Index Array(array=w1557, index=0 ("Index")) -> (element=w1551:dbl)
        n382 = Index Array(array=w1557, index=4 ("Index")) -> (element=w1556:dbl)
        n383 = Index Array(array=w1557, index=2 ("Index")) -> (element=w1553:dbl)
        n384 = call "4155C Config V Stress.vi"("VISA session"=w1590, "ID compliance"=w1554, "VD"=w1552, "VG"=w1551, "IG compliance"=w1553, "error in (no error)"=w1589, "Display on/off"=TRUE) -> ("dup VISA resource name"=w1592:refnum<visa-resource-name>, "error out"=w1591:errorcluster)
        n385 = call "4155C Apply Stress.vi"("error in (no error)"=w1591, "Duration"=w1556, "Emergency Stop"=w1570, "VISA resource name in"=w1592) -> ("error out"=w1568:errorcluster, "VISA Resource Name out"=w1566:refnum<visa-resource-name>)
        n386 = VISA Write(VISA resource name=w1566, write buffer=":DISP ON" ("write buffer (\"\")"), error in (no error)=w1568) -> (VISA resource name out=w1565:refnum<visa-resource-name>, error out=w1567:errorcluster)  [unwired: 1 out]
        n387 = call <vilib>:"compatOverwrite.vi"("overwrite (F)"=TRUE) -> ("overwrite?"=w1550:T8)
        n388 = Open/Create/Replace File(file path (use dialog)=w1575, error in=w1567, operation (0:open)=w1550) -> (refnum out=w1578:refnum<file>, error out=w1577:errorcluster)  [unwired: 3 in, 1 out]
        n389 = call "4155C Write array to file.vi"("Byte Stream File Refnum"=w1578, "Header"=string[] ["V stress completed successfully", ""], "error in (no error)"=w1577) -> ("dup refnum"=w1580:refnum<file>, "error out"=w1579:errorcluster)  [unwired: 2 in]
        n390 = Close File(refnum=w1580, error in=w1579) -> (error out=w1573:errorcluster)  [unwired: 1 out]
      }
      frame "stressI" {
        n391 = Number To Decimal String(number=w1613) -> (decimal integer string=w1650:string)  [unwired: 1 in]
        n392 = Concatenate Strings(w1634, "-stressI-" ("Substring"), w1650, w1612, ".txt" ("Substring")) -> (w1648:string)
        n393 = Fract/Exp String To Number(string=w1647) -> (number=w1622:dbl[])  [unwired: 3 in, 1 out]
        n394 = Index Array(array=w1622, index=1 ("Index")) -> (element=w1618:dbl)
        n395 = Index Array(array=w1622, index=0 ("Index")) -> (element=w1619:dbl)
        n396 = call "4155C Config I Stress.vi"("VISA session"=w1653, "IDG"=w1619, "VDG compliance"=w1618, "error in (no error)"=w1652, "Display on/off"=TRUE) -> ("dup VISA resource name"=w1655:refnum<visa-resource-name>, "error out"=w1654:errorcluster)
        n397 = Index Array(array=w1622, index=2 ("Index")) -> (element=w1620:dbl)
        n398 = String To Path(string=w1648) -> (path=w1638:path)
        n399 = call "4155C Apply Stress.vi"("error in (no error)"=w1654, "Duration"=w1620, "Emergency Stop"=w1633, "VISA resource name in"=w1655) -> ("error out"=w1631:errorcluster, "VISA Resource Name out"=w1629:refnum<visa-resource-name>)
        n400 = VISA Write(VISA resource name=w1629, write buffer=":DISP ON" ("write buffer (\"\")"), error in (no error)=w1631) -> (VISA resource name out=w1628:refnum<visa-resource-name>, error out=w1630:errorcluster)  [unwired: 1 out]
        n401 = call <vilib>:"compatOverwrite.vi"("overwrite (F)"=TRUE) -> ("overwrite?"=w1617:T8)
        n402 = Open/Create/Replace File(file path (use dialog)=w1638, error in=w1630, operation (0:open)=w1617) -> (refnum out=w1641:refnum<file>, error out=w1640:errorcluster)  [unwired: 3 in, 1 out]
        n403 = call "4155C Write array to file.vi"("Byte Stream File Refnum"=w1641, "Header"=string[] ["I stress completed successfully", ""], "error in (no error)"=w1640) -> ("dup refnum"=w1643:refnum<file>, "error out"=w1642:errorcluster)  [unwired: 2 in]
        n404 = Close File(refnum=w1643, error in=w1642) -> (error out=w1636:errorcluster)  [unwired: 1 out]
      }
      frame "vsu2pulse" {
        n405 = Number To Decimal String(number=w1676) -> (decimal integer string=w1711:string)  [unwired: 1 in]
        n406 = Concatenate Strings(w1696, "-vsu2-" ("Substring"), w1711, w1675, ".txt" ("Substring")) -> (w1709:string)
        n407 = Fract/Exp String To Number(string=w1708) -> (number=w1684:dbl[])  [unwired: 3 in, 1 out]
        n408 = String To Path(string=w1709) -> (path=w1700:path)
        n409 = Index Array(array=w1684, index=1 ("Index")) -> (element=w1683:dbl)
        n410 = Index Array(array=w1684, index=0 ("Index")) -> (element=w1681:dbl)
        n411 = call "4155C Config VSU2 Stress.vi"("error in (no error)"=w1713, "VSU2"=w1681, "Display on/off"=TRUE, "VISA session"=w1714) -> ("error out"=w1715:errorcluster, "dup VISA resource name"=w1716:refnum<visa-resource-name>)
        n412 = call "4155C Apply Stress.vi"("error in (no error)"=w1715, "Duration"=w1683, "Emergency Stop"=w1695, "VISA resource name in"=w1716) -> ("error out"=w1693:errorcluster, "VISA Resource Name out"=w1691:refnum<visa-resource-name>)
        n413 = VISA Write(VISA resource name=w1691, write buffer=":DISP ON" ("write buffer (\"\")"), error in (no error)=w1693) -> (VISA resource name out=w1690:refnum<visa-resource-name>, error out=w1692:errorcluster)  [unwired: 1 out]
        n414 = call <vilib>:"compatOverwrite.vi"("overwrite (F)"=TRUE) -> ("overwrite?"=w1680:T8)
        n415 = Open/Create/Replace File(file path (use dialog)=w1700, error in=w1692, operation (0:open)=w1680) -> (refnum out=w1703:refnum<file>, error out=w1702:errorcluster)  [unwired: 3 in, 1 out]
        n416 = call "4155C Write array to file.vi"("Byte Stream File Refnum"=w1703, "Header"=string[] ["VSU2 pulse completed successfully", ""], "error in (no error)"=w1702) -> ("dup refnum"=w1705:refnum<file>, "error out"=w1704:errorcluster)  [unwired: 2 in]
        n417 = Close File(refnum=w1705, error in=w1704) -> (error out=w1698:errorcluster)  [unwired: 1 out]
      }
      frame "sample-fpp" {
        w1748 = string[] ["Time /s", "Id VgVd /A", "Ig VgVd /A", "Vp1 VgVd /V", "Vp2 VgVd /V"] ("Header")
        w1752 = "%d" ("format string")
        n418 = Number To Decimal String(number=w1737) -> (decimal integer string=w1800:string)  [unwired: 1 in]
        n419 = Fract/Exp String To Number(string=w1797) -> (number=w1785:dbl[])  [unwired: 3 in, 1 out]
        n420 = Concatenate Strings(w1791, "-samplefpp-" ("Substring"), w1800, w1736, ".txt" ("Substring")) -> (w1798:string)
        n421 = String To Path(string=w1798) -> (path=w1760:path)
        n422 = Index Array(array=w1785, index=0 ("Index")) -> (element=w1746:dbl)
        n423 = Index Array(array=w1785, index=1 ("Index")) -> (element=w1745:dbl)
        n424 = Index Array(array=w1785, index=2 ("Index")) -> (element=w1793:dbl)
        n425 = Index Array(array=w1785, index=3 ("Index")) -> (element=w1783:dbl)
        n426 = call "4155C Config Sampling Measurements FPP.vi"("VISA session"=w1803, "Num Points"=w1793, "Vg"=w1746, "Display on/off"=TRUE, "Gate Compliance"=w1792, "Drain Compliance"=w1801, "Standby"="Standby", "error in (no error)"=w1802, "Timings"=w1790, "Vd"=w1745, "Sample time"=w1783) -> ("dup VISA resource name"=w1762:refnum<visa-resource-name>, "error out"=w1761:errorcluster)  [unwired: 3 in]
        n427 = Number To Decimal String(number=w1746) -> (decimal integer string=w1772:string)  [unwired: 1 in]
        n428 = call "4155C Take Sample FPP.vi"("VISA resource name in"=w1762, "error in (no error)"=w1761, "Emergency Stop"=w1763) -> ("Time"=w1767:dbl[], "Vp1"=w1777:dbl[], "VISA Resource Name out"=w1743:refnum<visa-resource-name>, "Ig"=w1765:dbl[], "Id"=w1766:dbl[], "Vp2"=w1775:dbl[], "error out"=w1764:errorcluster)  [unwired: 10 in]
        n429 = Insert Into Array(array=dbl[][] [] ("Input Array"), new element=w1767) -> (w1781:dbl[][])  [unwired: 2 in]
        n430 = Number To Decimal String(number=w1745) -> (decimal integer string=w1770:string)  [unwired: 1 in]
        n431 = Insert Into Array(array=w1781, new element=w1766) -> (w1780:dbl[][])  [unwired: 2 in]
        n432 = Concatenate Strings("(Vg = " ("Substring"), w1772, "V, Vd = " ("Substring"), w1770, "V)" ("Substring")) -> (w1768:string)
        n433 = Insert Into Array(array=w1780, new element=w1765) -> (w1779:dbl[][])  [unwired: 2 in]
        n434 = Insert Into Array(array=w1779, new element=w1777) -> (w1776:dbl[][])  [unwired: 2 in]
        n435 = Insert Into Array(array=w1776, new element=w1775) -> (w1744:dbl[][])  [unwired: 2 in]
        n436 = Transpose 2D Array(2D array=w1744) -> (transposed array=w1774:dbl[][])
        n437 = call <vilib>:"compatOverwrite.vi"("overwrite (F)"=TRUE) -> ("overwrite?"=w1741:T8)
        n438 = Open/Create/Replace File(file path (use dialog)=w1760, error in=w1764, operation (0:open)=w1741) -> (refnum out=w1757:refnum<file>, error out=w1758:errorcluster)  [unwired: 3 in, 1 out]
        n439 = Array To Spreadsheet String(array=w1748, 3:w1752) -> (spreadsheet string=w1754:string)  [unwired: 1 in]
        n440 = Search and Replace String(replace all?=TRUE ("replace all? (F)"), input string=w1754, search string="VgVd", replace string=w1768) -> (result string=w1750:string)  [unwired: 4 in, 3 out]
        n441 = Spreadsheet String To Array(format string=w1752, spreadsheet string=w1750, array type (2D Dbl)=w1748) -> (array=w1749:string[])  [unwired: 1 in]
        n442 = call "4155C Write array to file.vi"("Byte Stream File Refnum"=w1757, "Header"=w1749, "Data Array"=w1774, "error in (no error)"=w1758) -> ("dup refnum"=w1755:refnum<file>, "error out"=w1756:errorcluster)  [unwired: 1 in]
        n443 = Close File(refnum=w1755, error in=w1756) -> (error out=w1742:errorcluster)  [unwired: 1 out]
      }
      frame "resample-fpp" {
        w1837 = string[] ["Time /s", "Id VgVd /A", "Ig VgVd /A", "Vp1 VgVd /V", "Vp2 VgVd /V"] ("Header")
        w1841 = "%d" ("format string")
        n444 = Number To Decimal String(number=w1823) -> (decimal integer string=w1881:string)  [unwired: 1 in]
        n445 = Fract/Exp String To Number(string=w1878) -> (number=w1830:dbl[])  [unwired: 3 in, 1 out]
        n446 = Concatenate Strings(w1874, "-resamplefpp-" ("Substring"), w1881, w1824, ".txt" ("Substring")) -> (w1879:string)
        n447 = String To Path(string=w1879) -> (path=w1849:path)
        n448 = Index Array(array=w1830, index=0 ("Index")) -> (element=w1836:dbl)
        n449 = Index Array(array=w1830, index=1 ("Index")) -> (element=w1835:dbl)
        n450 = Number To Decimal String(number=w1836) -> (decimal integer string=w1859:string)  [unwired: 1 in]
        n451 = call "4155C Take Sample FPP.vi"("VISA resource name in"=w1832, "error in (no error)"=w1831, "Emergency Stop"=w1850) -> ("Time"=w1854:dbl[], "Vp1"=w1864:dbl[], "VISA Resource Name out"=w1834:refnum<visa-resource-name>, "Ig"=w1852:dbl[], "Id"=w1853:dbl[], "Vp2"=w1862:dbl[], "error out"=w1851:errorcluster)  [unwired: 10 in]
        n452 = Insert Into Array(array=dbl[][] [] ("Input Array"), new element=w1854) -> (w1868:dbl[][])  [unwired: 2 in]
        n453 = Number To Decimal String(number=w1835) -> (decimal integer string=w1857:string)  [unwired: 1 in]
        n454 = Insert Into Array(array=w1868, new element=w1853) -> (w1867:dbl[][])  [unwired: 2 in]
        n455 = Concatenate Strings("(Vg = " ("Substring"), w1859, "V, Vd = " ("Substring"), w1857, "V)" ("Substring")) -> (w1855:string)
        n456 = Insert Into Array(array=w1867, new element=w1852) -> (w1866:dbl[][])  [unwired: 2 in]
        n457 = Insert Into Array(array=w1866, new element=w1864) -> (w1863:dbl[][])  [unwired: 2 in]
        n458 = Insert Into Array(array=w1863, new element=w1862) -> (w1829:dbl[][])  [unwired: 2 in]
        n459 = call <vilib>:"compatOverwrite.vi"("overwrite (F)"=TRUE) -> ("overwrite?"=w1828:T8)
        n460 = Open/Create/Replace File(file path (use dialog)=w1849, error in=w1851, operation (0:open)=w1828) -> (refnum out=w1846:refnum<file>, error out=w1847:errorcluster)  [unwired: 3 in, 1 out]
        n461 = Array To Spreadsheet String(array=w1837, 3:w1841) -> (spreadsheet string=w1843:string)  [unwired: 1 in]
        n462 = Transpose 2D Array(2D array=w1829) -> (transposed array=w1861:dbl[][])
        n463 = Search and Replace String(replace all?=TRUE ("replace all? (F)"), input string=w1843, search string="VgVd", replace string=w1855) -> (result string=w1839:string)  [unwired: 4 in, 3 out]
        n464 = Spreadsheet String To Array(format string=w1841, spreadsheet string=w1839, array type (2D Dbl)=w1837) -> (array=w1838:string[])  [unwired: 1 in]
        n465 = call "4155C Write array to file.vi"("Byte Stream File Refnum"=w1846, "Header"=w1838, "Data Array"=w1861, "error in (no error)"=w1847) -> ("dup refnum"=w1844:refnum<file>, "error out"=w1845:errorcluster)  [unwired: 1 in]
        n466 = Close File(refnum=w1844, error in=w1845) -> (error out=w1833:errorcluster)  [unwired: 1 out]
      }
      frame "serial" {
        n467 = local read "Termination char\n(0xA = '\\n' = LF)\n(0xD = '\\r' = CR)"() -> (w1909:u8)
        n468 = local read "Enable Termination\nChar (T)"() -> (w1910:bool)
        n469 = Index Array(array=w1917, index=0 ("Index")) -> (element=w1916:string)
        n470 = local read "parity"() -> (w1900:u16)
        n471 = local read "Delay before read (ms)"() -> (w1911:u32)
        n472 = local read "byte count"() -> (w1908:u32)
        n473 = local read "Timeout (ms)"() -> (w1907:u32)
        n474 = local read "VISA resource name"() -> (w1904:refnum<visa-resource-name>)
        n475 = local read "baud rate"() -> (w1903:u32)
        n476 = local read "Serial End Mode for Reads"() -> (w1902:u16)
        n477 = local read "data bits"() -> (w1901:u16)
        n478 = local read "stop bits"() -> (w1906:u16)
        n479 = local read "flow control"() -> (w1905:u16)
        n480 = call "Serial write and read v0.5.vi"("Delay before read (ms)"=w1911, "Termination char\n(0xA = '\\n' = LF)\n(0xD = '\\r' = CR)"=w1909, "Enable Termination\nChar (T)"=w1910, "parity"=w1900, "stop bits"=w1906, "string to write"=w1916, "flow control"=w1905, "byte count"=w1908, "Serial Settings:Serial End Mode for Reads"=w1902, "Timeout (ms)"=w1907, "error in (no error)"=w1922, "VISA resource name"=w1904, "baud rate"=w1903, "data bits"=w1901) -> ("read string"=w1912:string, "error out"=w1921:errorcluster)
        n481 = Build Array (concatenate)(w1912, w1913) -> (w1914:string[])
      }
      frame "pump" {
        # "Time array for valve position"
        # "Time array for absolute plunger position"
        # "Valve position"
        # "Absolute plunger position"
        # "Remove \"_\""
        # "Check if hard stop is pressed."
        # "Check if halt is pressed."
        # "Check if pump is idle. Else halt."
        n482 = Index Array(array=w1987, index=0 ("Index")) -> (element=w1964:string)
        n483 = case shown="\"No error\", Default" w1962 {
          tunnel: w1964 -> [w2023 _ w2025 w2026 w2027 w2028 _ _ w2031 w2032 _]
          tunnel: [w2023 "/1H" w2025 w2026 w2027 w2028 "/1H" "/1H" w2031 w2032 "/1H"] -> w1963
          frame "No error", Default {
          }
          frame "Initialization" {
          }
          frame "Invalid command" {
          }
          frame "Invalid operand" {
          }
          frame "Device not initialized" {
          }
          frame "Internal failure" {
          }
          frame "Plunger overload" {
          }
          frame "Valve overload" {
          }
          frame "Plunger move not allowed" {
          }
          frame "A/D converter failure" {
          }
          frame "Command overflow" {
          }
        }
        n484 = local read "Hard stop pump"() -> (w1966:bool)
        n485 = local read "Halt pump"() -> (w1969:bool)
        n486 = local read "Serial End Mode for Reads"() -> (w1975:u16)
        n487 = local read "flow control"() -> (w1978:u16)
        n488 = local read "stop bits"() -> (w1979:u16)
        n489 = local read "parity"() -> (w1973:u16)
        n490 = local read "Delay before read (ms)"() -> (w1984:u32)
        n491 = local read "byte count"() -> (w1981:u32)
        n492 = local read "Timeout (ms)"() -> (w1980:u32)
        n493 = local read "VISA resource name"() -> (w1977:refnum<visa-resource-name>)
        n494 = local read "baud rate"() -> (w1976:u32)
        n495 = local read "Enable Termination\nChar (T)"() -> (w1983:bool)
        n496 = local read "Termination char\n(0xA = '\\n' = LF)\n(0xD = '\\r' = CR)"() -> (w1982:u8)
        n497 = case shown="True" w1969 {
          tunnel: [w2037 "/1H"] -> w1968
          tunnel: w1963 -> [w2037 _]
          frame False {
          }
          frame True {
            n498 = local write "Halt pump"(FALSE) -> ()
          }
        }
        n499 = case shown="True" w1966 {
          tunnel: [w2034 "/1T"] -> w1967
          tunnel: w1968 -> [w2034 _]
          frame False {
          }
          frame True {
            n500 = local write "Hard stop pump"(FALSE) -> ()
          }
        }
        n501 = local read "data bits"() -> (w1974:u16)
        n502 = String Subset(string=w1958, offset (0)=1) -> (substring=w1956:string)  [unwired: 1 in]
        n503 = call "SPM Pump v0.6.vi"("Termination char\n(0xA = '\\n' = LF)\n(0xD = '\\r' = CR)"=w1982, "Enable Termination\nChar (T)"=w1983, "Timeout (ms)"=w1980, "Serial Settings:Serial End Mode for Reads"=w1975, "byte count"=w1981, "Delay before read (ms)"=w1984, "Time <input>"=w1961, "error in (no error)"=w1992, "Serial port input"=w1967, "VISA resource name"=w1977, "parity"=w1973, "baud rate"=w1976, "stop bits"=w1979, "data bits"=w1974, "flow control"=w1978, "Time units <input>"=w1956) -> ("Input command"=w1955:string, "Serial port data"=w1945:string[], "Pump status"=w1951:string, "Valve position"=w1953:i32, "Absolute plunger position"=w1965:i32, "Serial port"=w1960:string, "error out"=w1991:errorcluster)  [unwired: 1 in, 4 out]
        n504 = case shown="\"?6\"" w1955 {
          tunnel: [w2004 w2012 w2018] -> w1972
          tunnel: w1971 -> [w2004 w2011 w2018]
          tunnel: w1965 -> [_ w2010 _]
          tunnel: w1952 -> [w2003 w2009 w2019]
          tunnel: [w2003 w2009 w2021] -> w1954
          tunnel: w1953 -> [_ _ w2020]
          tunnel: w1950 -> [_ w2008 w2016]
          tunnel: w1949 -> [w2002 w2007 w2017]
          tunnel: [w2002 w2006 w2017] -> w1948
          tunnel: [w2001 w2005 w2015] -> w1947
          tunnel: w1946 -> [w2001 w2005 w2014]
          frame "Q", Default {
          }
          frame "?" {
            n505 = Build Array (concatenate)(w2011, w2010) -> (w2012:i32[])
            n506 = Build Array (concatenate)(w2007, w2008) -> (w2006:i32[])
            n507 = call "4155C Split array.vi"("X data in"=w2006, "Y1 data in"=w2012) -> ("Array of clusters"=w2013:cluster{"Y data in":dbl[], "X data in":dbl[]}[])  [unwired: 5 in, 1 out]
            n508 = local write "Absolute plunger position vs time"(w2013) -> ()
          }
          frame "?6" {
            n509 = Build Array (concatenate)(w2019, w2020) -> (w2021:i32[])
            n510 = Build Array (concatenate)(w2014, w2016) -> (w2015:i32[])
            n511 = call "4155C Split array.vi"("X data in"=w2015, "Y1 data in"=w2021) -> ("Array of clusters"=w2022:cluster{"Y data in":dbl[], "X data in":dbl[]}[])  [unwired: 5 in, 1 out]
            n512 = local write "Valve position vs time"(w2022) -> ()
          }
        }
        n513 = Build Array (concatenate)(w1943, w1945) -> (w1944:string[][])
        n514 = Build Array (concatenate)(w1959, w1960) -> (w1985:string[])
      }
      frame "filename" {
        n515 = Index Array(array=w2041, index=0 ("Index")) -> (element=w2040:string)
      }
    }
    n516 = Build Array(w135, w64, w74, w73, w72, w71, w70, w69, w68, w67, w66, w65, w63) -> (w174:dbl[][])
    n517 = Transpose 2D Array(2D array=w174) -> (transposed array=w173:dbl[][])
    n518 = Concatenate Strings(w115, w58, "Imax_Imin_Ion_Ioff_vs_time.txt" ("Suffix (Imax,Imin,Ion,Ioff)")) -> (w184:string)
    n519 = Build Array(w96, "Is max (A)" ("VAR2 Name"), "Is min (A)" ("VAR2 Name"), "Id max (A)" ("VAR2 Name"), "Id min (A)" ("VAR2 Name"), "Ig max (A)" ("VAR2 Name"), "Ig min (A)" ("VAR2 Name"), "Is on (A)" ("VAR2 Name"), "Is off (A)" ("VAR2 Name"), "Id on (A)" ("VAR2 Name"), "Id off (A)" ("VAR2 Name"), "Ig on (A)" ("VAR2 Name"), "Ig off (A)" ("VAR2 Name")) -> (w179:string[])
    n520 = Array To Spreadsheet String(array=w173, 3:"%e" ("format string")) -> (spreadsheet string=w177:string)  [unwired: 1 in]
    n521 = Array To Spreadsheet String(array=w179, 3:"" ("format string")) -> (spreadsheet string=w178:string)  [unwired: 1 in]
    n522 = String To Path(string=w184) -> (path=w183:path)
    n523 = Build Array(w178, w177) -> (w176:string[])
    n524 = Write to Text File(file (use dialog)=w183, text=w176, error in=w131) -> (refnum out=w185:refnum<file>, error out=w175:errorcluster)  [unwired: 1 in, 1 out]
    n525 = Close File(refnum=w185, error in=w175) -> (error out=w114:errorcluster)  [unwired: 1 out]
    n526 = Build Array(w110, w136) -> (w141:i32[][])
    n527 = Build Array(w96, "Absolute plunger position" ("VAR2 Name")) -> (w144:string[])
    n528 = Transpose 2D Array(2D array=w141) -> (transposed array=w134:i32[][])
    n529 = Array To Spreadsheet String(array=w144, 3:"" ("format string")) -> (spreadsheet string=w143:string)  [unwired: 1 in]
    n530 = Array To Spreadsheet String(array=w134, 3:"%e" ("format string")) -> (spreadsheet string=w140:string)  [unwired: 1 in]
    n531 = Build Array(w143, w140) -> (w146:string[])
    n532 = Concatenate Strings(w115, w58, "plunger_vs_time.txt" ("Suffix (plunger)")) -> (w138:string)
    n533 = String To Path(string=w138) -> (path=w137:path)
    n534 = Write to Text File(file (use dialog)=w137, text=w146, error in=w114) -> (refnum out=w139:refnum<file>, error out=w148:errorcluster)  [unwired: 1 in, 1 out]
    n535 = Close File(refnum=w139, error in=w148) -> (error out=w113:errorcluster)  [unwired: 1 out]
    n536 = Concatenate Strings(w115, w58, "serial_port_output.txt" ("Suffix (serial port log)")) -> (w154:string)
    n537 = String To Path(string=w154) -> (path=w153:path)
    n538 = Build Array(w96, "Serial port input" ("VAR2 Name"), "Pump status" ("VAR2 Name"), "Serial port output: ") -> (w100:string[])
    n539 = Array To Spreadsheet String(array=w106, 3:"" ("format string")) -> (spreadsheet string=w97:string)  [unwired: 1 in]
    n540 = Array To Spreadsheet String(array=w100, 3:"" ("format string")) -> (spreadsheet string=w98:string)  [unwired: 1 in]
    n541 = Build Array(w98, w97) -> (w99:string[])
    n542 = Array To Spreadsheet String(array=w105, 3:"" ("format string")) -> (spreadsheet string=w159:string)  [unwired: 1 in]
    n543 = Write to Text File(file (use dialog)=w153, text=w99, error in=w113) -> (refnum out=w155:refnum<file>, error out=w156:errorcluster)  [unwired: 1 in, 1 out]
    n544 = Close File(refnum=w155, error in=w156) -> (error out=w112:errorcluster)  [unwired: 1 out]
    n545 = local write "Serial port data"(w159) -> ()
    n546 = Build Array(w109, w117) -> (w123:i32[][])
    n547 = Build Array(w96, "Valve port" ("VAR2 Name")) -> (w126:string[])
    n548 = Transpose 2D Array(2D array=w123) -> (transposed array=w118:i32[][])
    n549 = Array To Spreadsheet String(array=w126, 3:"" ("format string")) -> (spreadsheet string=w125:string)  [unwired: 1 in]
    n550 = Array To Spreadsheet String(array=w118, 3:"%e" ("format string")) -> (spreadsheet string=w122:string)  [unwired: 1 in]
    n551 = Build Array(w125, w122) -> (w128:string[])
    n552 = Concatenate Strings(w115, w58, "valve_port_vs_time.txt" ("Suffix (valve)")) -> (w120:string)
    n553 = String To Path(string=w120) -> (path=w119:path)
    n554 = Write to Text File(file (use dialog)=w119, text=w128, error in=w112) -> (refnum out=w121:refnum<file>, error out=w130:errorcluster)  [unwired: 1 in, 1 out]
    n555 = Close File(refnum=w121, error in=w130) -> (error out=w111:errorcluster)  [unwired: 1 out]
  }
  "error out" <- w20
  "Timings Indicator" <- w2
